vi "MC_8_27_12e_JW.vi"() -> ()   [LabVIEW 2011]
uses:
  <vilib>/Utility/file.llb/Read From Spreadsheet File (string).vi
  <vilib>/Utility/inputDevices.llb/keyboardAcquire.vi
  <vilib>/Utility/file.llb/Write To Spreadsheet File (DBL).vi
  <vilib>/Utility/file.llb/Write To Spreadsheet File (string).vi
  <vilib>/regexp/Match Regular Expression.xnode
panel:
  out "Vg Column":dbl[](array[numeric])
  out "Data Length":dbl
  in  "default (0 dbl) 6":ext format="%.2e"
  in  "default (0 dbl) 5":ext format="%.2e"
  in  "default (0 dbl) 4":ext format="%.2e"
  in  "default (0 dbl) 3":ext format="%.2e"
  in  "default (0 dbl)":ext format="%.2e"
  out "X Axis Display Type":string
  out "Opj X Axis":string
  in  "Room Temp":dbl=294.0
  out "No Image 2":path=path "\\\\acad1\\physics/Jurchescu-group/JW-PD/Image Not Found.png"
  out "Save1 Array":string[][](array[string])
  out "Lin Vd":dbl
  out "Lin-Vg Array-Used":dbl[](array[numeric])
  out "Lin Id-Used":dbl[](array[numeric])
  out "Rec: Comments":string
  out "Folder Index":dbl caption="Length"
  out "Current \nRecord":string[](array[string])
  out "Transformer \nHeaders":string[](array[string])
  out "Current Device ID":string
  out "Column":string
  out "Row":string
  out "Rec: Concentration":dbl
  out "Rec: Solvent":string
  out "Rec: Method":string
  in  "?":T1(tab)
  in  "Transport File":path
  out "Transport Folder":path
  out "Rec: Material":string
  out "Accel (RPM/s):":dbl
  in  "Transfer File":path
  out "Transfer Folder":path
  in  "Image Folder":path
  out "Image File":path=path "D:/UserData/Desktop/Jeremy/WFU/Research/Programs/VI mods/Image Not Found.png"
  in  "Manual Comments":bool
  in  "Comments:":string
  out "Calc: On/Off":dbl caption="On/Off-Sat" format="%#.2e"
  out "Calc: Off I-Sat":dbl caption="Off I-Sat" format="%#.2e"
  in  "Manuel-Dielectric":bool
  in  "Manuel-Length":bool
  out "Calc: VT-Lin":dbl
  out "New: VT-Lin":dbl
  out "Rec: VT-Lin":dbl caption="VT-Lin" format="%#_3g"
  out "Calc: Trap Density-STS":dbl format="%#.2e"
  out "New: Trap Density-STS":dbl format="%#.2e"
  out "Rec: Trap Density-STS":dbl caption="N-Sat (STS)" format="%#.2e"
  out "Calc: Trap Density-VT":dbl format="%#.2e"
  out "New: Trap Density-VT":dbl format="%#.2e"
  out "Rec: Trap Density-VT":dbl caption="N-Sat (VT)" format="%#.2e"
  out "Calc: Mobility-Lin":dbl format="%#.2e"
  out "New: Mobility-Lin":dbl format="%#_4e"
  out "Rec: Mobility-Lin":dbl caption="Mobility-Lin" format="%#_3e"
  out "Calc: Mobility-Sat":dbl format="%#.2e"
  out "Rec: Length":dbl caption="Length" format="%#_3g"
  out "Rec: Width":dbl caption="Width" format="%#_4g"
  out "Rec: Dielectric (d)":dbl caption="Dielectric (d)" format="%#_3g"
  in  "Cancel Button":bool
  in  "Up Button":bool
  in  "Down Button":bool
  out "Data Name:":string
  in  "Save Changes?":bool
  in  "New: Dielectric":dbl
  in  "New: Length":dbl
  in  "New: Width":dbl
  out "New: Mobility-Sat":dbl format="%#.2e"
  in  "Blank Button":bool
  in  "Zoom":i16(slide)=-3 scale=-5.0..5.0
  out "Image Out 2":T2(plugin-control)
  out "Image Out":T2(plugin-control)
  in  "Magnification":u16(ring) items=["5x", "10x", "20x", "50x", "80x"]
  out "Total Width":dbl
  out "Distances":dbl[](array[numeric])
  in  "Undo Button":bool
  in  "Remove Button":bool
  out "Rec: Mobility-Sat":dbl caption="Mobility-Sat" format="%#.2e"
  in  "Export":bool
  out "Calc: VT-Sat":dbl format="%#.2g"
  out "New: VT-Sat":dbl format="%#.2g"
  in  "Manual-Width":bool caption="Manual"
  out "Calc: STS":dbl format="%#.2g"
  out "New: STS":dbl format="%#.2g"
  out "Rec: VT-Sat":dbl caption="VT-Sat" format="%#.2g"
  out "Rec: STS":dbl caption="STS-Sat" format="%#.2g"
  out "Rec: On/Off":dbl caption="On/Off-Sat" format="%#.2e"
  in  "Save Changes? 2":bool
  in  "Save Changes? 3":bool
  out "Rec: Temp":dbl caption="Sample Temp" format="%.1f"
  in  "New: Temp":dbl format="%.1f"
  out "Rec: Off I-Sat":dbl caption="Off I-Sat" format="%#.2e"
  in  "Independant Variable":string(combo)="Length (um):"
  in  "Transfer Plots":T3(tab)=enum."Saturation"
  in  "Lin-Trans Slider":dbl(slide) step=1.0 scale=-22.0..89.0 scale format="%#_1p"
  out "Sqrt-Lin":cluster{dbl[], dbl[]}[](graph)
  in  "Next Sqrt Lin":bool
  in  "Previous Sqrt Lin":bool
  in  "Sat-Trans Slider":dbl(slide) step=1.0 scale=-40.0..40.0 scale format="%#_1p"
  out "Sqrt-Sat":cluster{dbl[], dbl[]}[](graph)
  in  "Previous Sqrt Sat":bool
  in  "Next Sqrt Sat":bool
  out "Raw- Lin":cluster{dbl[], dbl[]}[](graph)
  out "Raw- Sat":cluster{dbl[], dbl[]}[](graph)
  in  "Log Plots":enum32{"Linear", "Saturation", "Transport"}(tab)=enum."Saturation"
  in  "Lin-Log Slider":dbl(slide) step=1.0 scale=-1.0..82.0 scale format="%#_1p"
  in  "Previous Log Lin":bool
  in  "Next Log Lin":bool
  out "Log-Lin":cluster{dbl[], dbl[]}[](graph)
  in  "Sat-Log Slider":dbl(slide) step=1.0 scale=-1.0..82.0 scale format="%#_1p"
  in  "Previous Log Sat":bool
  in  "Next Log Sat":bool
  out "Sat-Log":cluster{dbl[], dbl[]}[](graph)
  out "Transport":cluster{dbl[], dbl[]}[](graph)
  in  "Manual-Temp":bool caption="Manual"
  out "Date Created":string caption="Fabricated"
  out "Date Recorded":string="Date Recorded" caption="Measured"
  out "Image Name":string
  out "Index":string
  in  "Num Pts":dbl=5.0
  in  "NumPoints Log":dbl=5.0 caption="Num Pts"
  in  "Ring":u16(ring) items=["Extra Small", "Small", "Medium", "Large", "Extra Large"]
  in  "Transport Line Color":u32(colorbox)
  in  "Origin Project File":path=path "\\\\acad1\\physics/Jurchescu-group/JW-PD/Group Library/Origin Project Files/DeviceData_8_10_12a_JW.opj"
  in  "No Image File":path=path "\\\\acad1\\physics/Jurchescu-group/JW-PD/Mega Awesome/Image Not Found.png"
  in  "Ramp (s):":dbl=3.0
  in  "Fabricator:":string="NaN"
  in  "Sample #:":dbl=1.0
  in  "Wait Time (s):":dbl=nan
  in  "RPM:":dbl=nan
  in  "Time (s):":dbl=nan
  in  "Room Temp (F):":dbl=nan
  in  "Relative Humidity (%):":dbl=nan
  in  "Solution Temp (C):":dbl=nan
  in  "# Drops*:":dbl=inf
  in  "Surface Treatment:":string="NaN"
  in  "Treatment Concentration (mM):":dbl=nan
  out "String":string
  out "Index 2":dbl
  out "Sat Id-Log-Used":dbl[](array[numeric])
  out "Vg Array-Log-Used":dbl[](array[numeric])
  out "ROI Descriptor out":T4 {"Contours"."Type" items=["No Selection", "Point", "Line", "Rectangle", "Oval", "Polygon", "Freehand Region", "Annulus", "Unused2", "Unused3", "Broken Line", "Freehand Line", "Rotated Rectangle"]}
  out "ROI Descriptor":T4 {"Contours"."Type" items=["No Selection", "Point", "Line", "Rectangle", "Oval", "Polygon", "Freehand Region", "Annulus", "Unused2", "Unused3", "Broken Line", "Freehand Line", "Rotated Rectangle"]}
  out "Numeric 3":dbl
  out "Array 6":dbl[][](array[numeric])
  out "Cluster":T5
  out "Array 5":dbl[](array[numeric])
  out "Array 4":dbl[](array[numeric])
  out "Array 3":dbl[](array[numeric])
  out "Numeric 2":dbl
  out "Numeric":dbl
  out "Sat Id-Used":dbl[](array[numeric])
  out "Sat Vg Array-Used":dbl[](array[numeric])
  out "MobVi Index":dbl
  in  "Row Start":dbl=20.0
  # "Data Locations"
  # "Transfer Location"
  # "Image Location"
  # "Recorded"
  # "Calculated"
  # "Re-Calculated"
  # "Manual"
  # "Used points display at y=0"
  # "Slider\nDoesn't\nWork"
  # "Slider\nDoesn't\nWork"
  # "No new points displayed"
  # "Sample Properties"
  # "*     Inf = Full coverage\n   NaN = Unknown or Not Applicable"
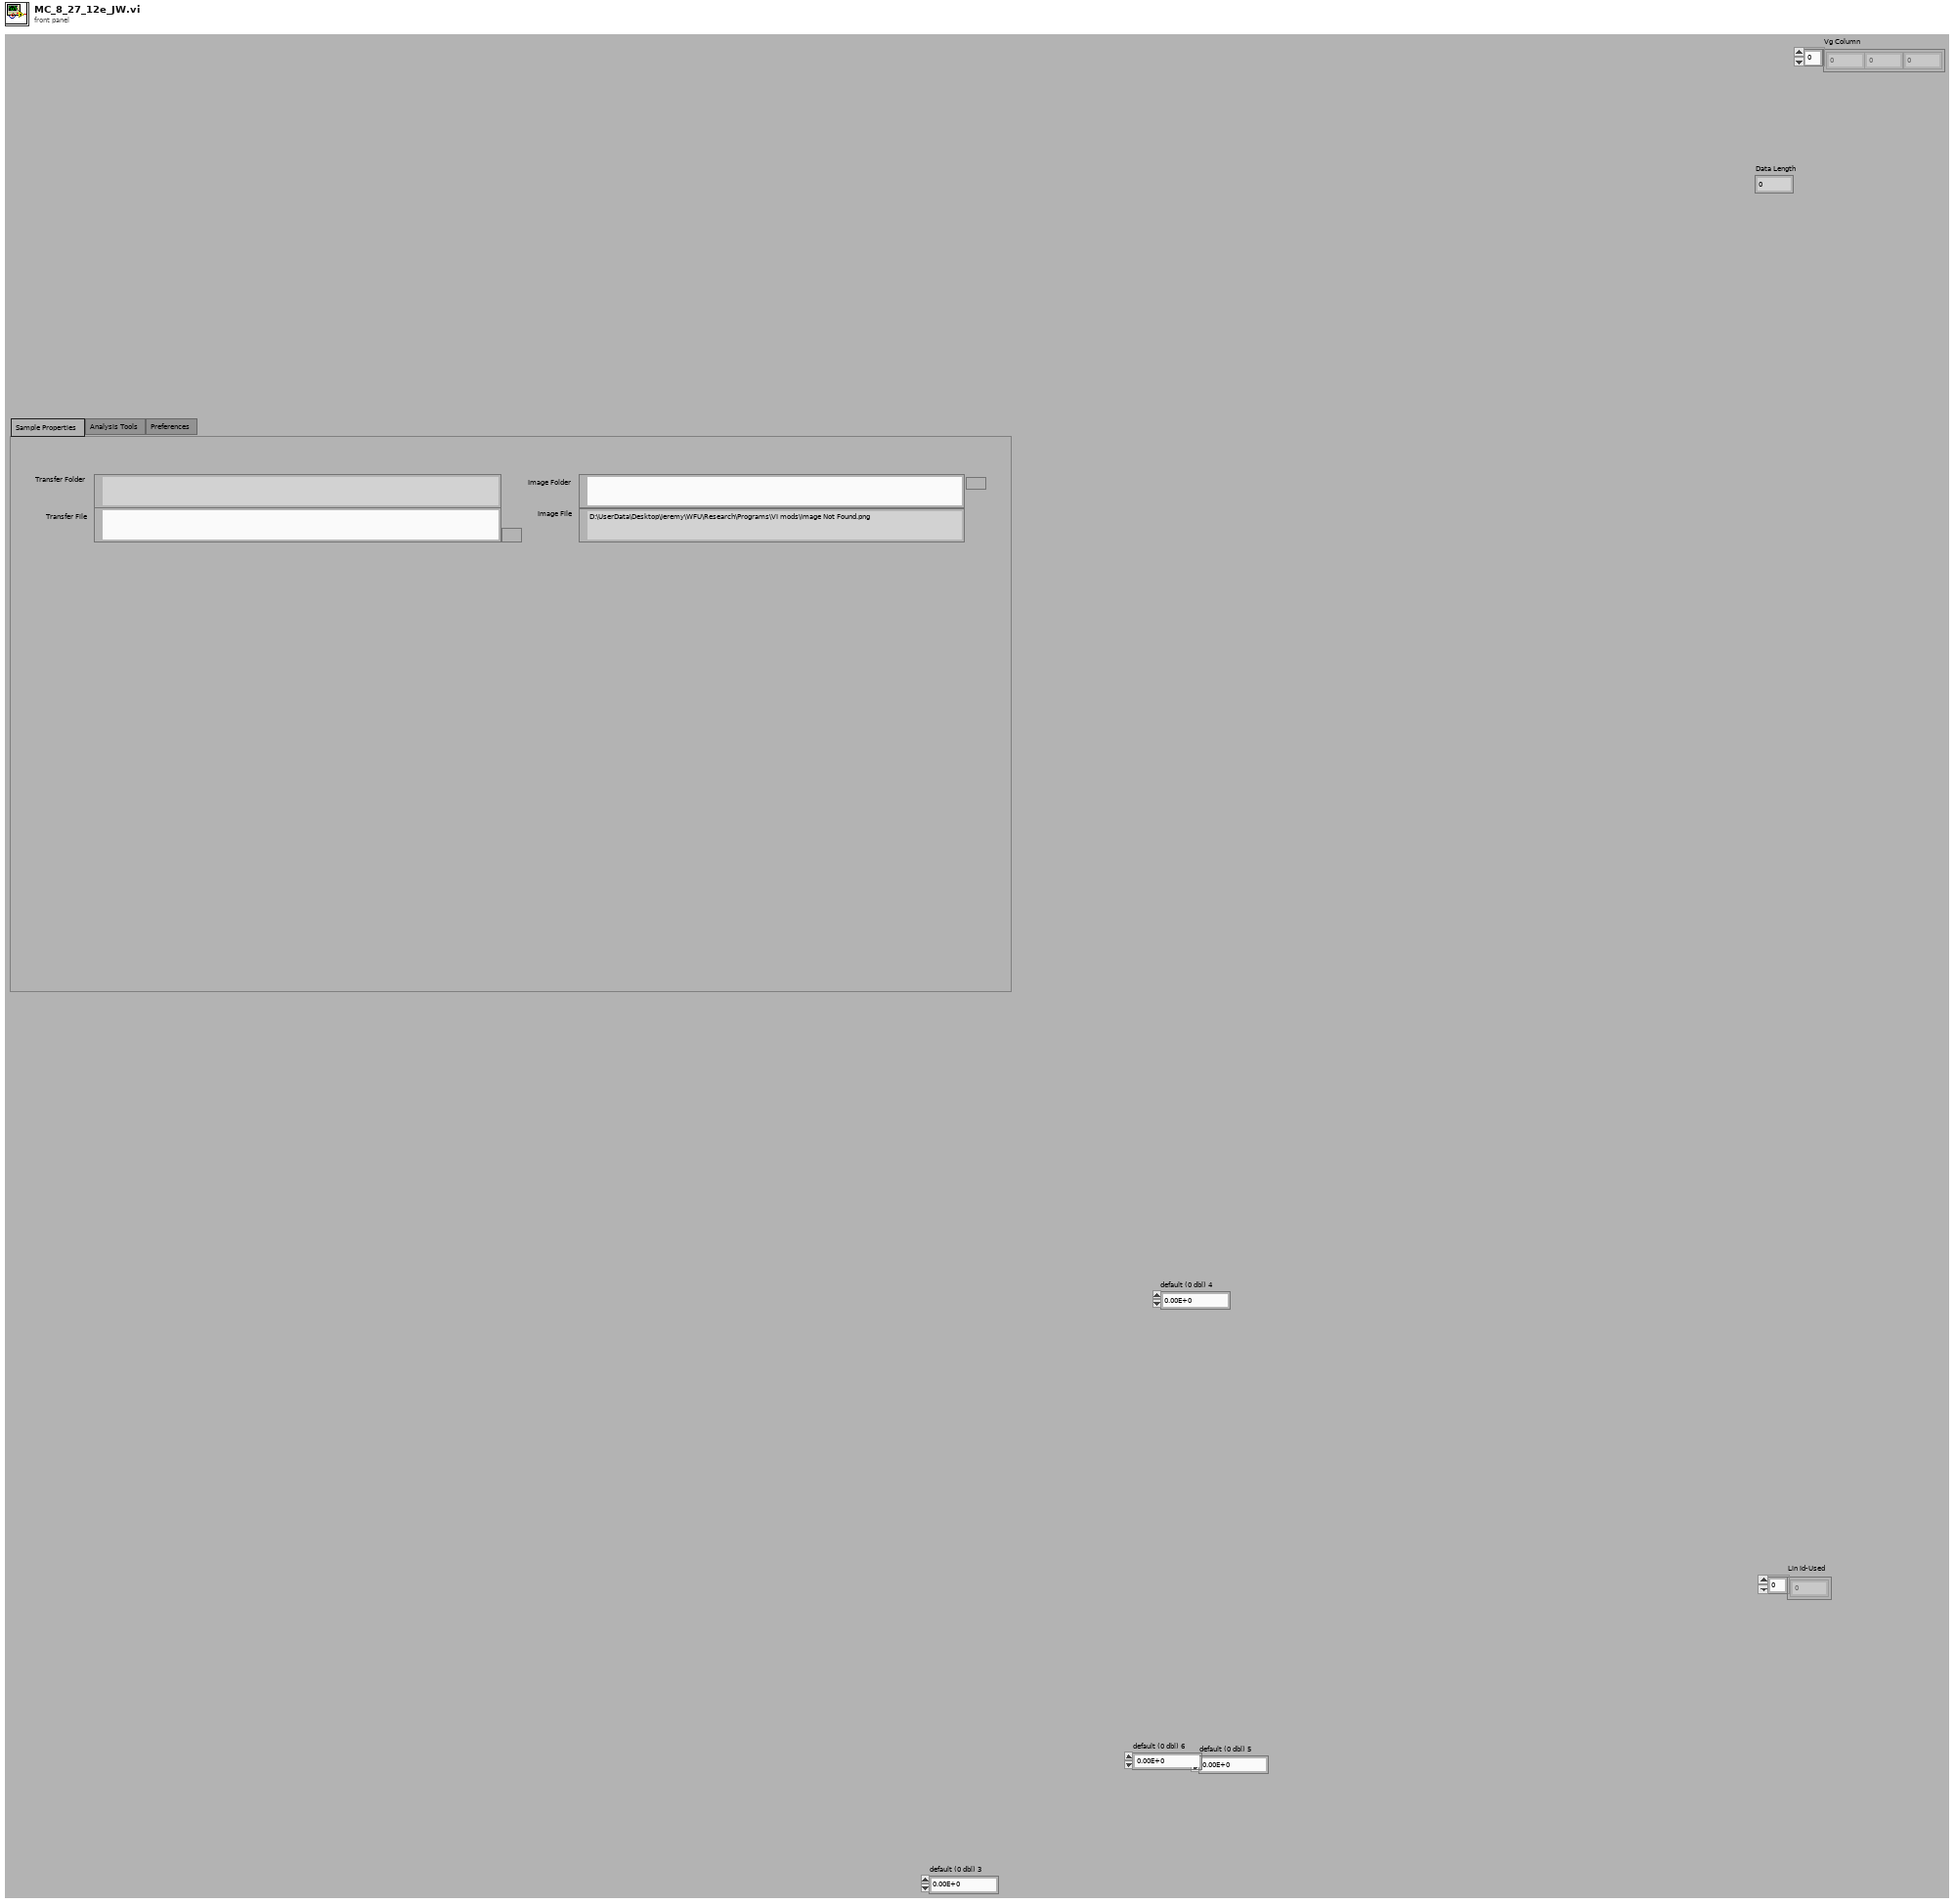
[diagram p1: front panel]
types:
  T1 = enum32{"Sample Properties", "Analysis Tools", "Preferences", "Current Database"}
  T2 = typedef "IMAQ Image.ctl" = refnum<image>
  T3 = enum32{"Linear", "Saturation", "Raw-Linear", "Raw-Saturation"}
  T4 = typedef "ROI Descriptor" = cluster{"Global Rectangle":i32[], "Contours":cluster{"ID":enum32{"External", "Internal"}, "Type":u32, "Coordinates":i32[]}[]}
  T5 = cluster{"Numeric":dbl, "Numeric 2":dbl, "Numeric 3":dbl, "Numeric 4":dbl}
  T6 = cluster{"Mobility-Sat":dbl, "Moblitity-Lin":dbl, "On/Off":dbl, "Off Current":dbl, "Vt-Sat":dbl, "STS":dbl, "Trap Density-VT":dbl, "Trap Density-STS":dbl}
  T7 = cluster{"Date Recorded":string, "Index":string, "Length":dbl, "Width":dbl, "Sample Temp":dbl}
  T8 = cluster{"Date Created":string, "Material":string, "Solvent":string, "Concentration":dbl, "Method":string, "Dielectric (nm)":dbl, "Treatment":string, "Comments":string}
  T9 = cluster{"Raw Sat":cluster{dbl[], dbl[]}[], "Sqrt Sat":cluster{dbl[], dbl[]}[], "Log Sat":cluster{dbl[], dbl[]}[], "Raw Lin":cluster{dbl[], dbl[]}[], "Sqrt Lin":cluster{dbl[], dbl[]}[], "Log Lin":cluster{dbl[], dbl[]}[]}
  T10 = cluster{"Mobility-Sat":dbl, "Vt-Sat":dbl, "Mobility-Lin":dbl, "Vt-Lin":dbl, "Off I-Sat":dbl, "On/Off I-Sat":dbl}
  T11 = cluster{"[0]":cluster{dbl[], dbl[]}, "[1]":cluster{dbl[], dbl[]}, "[2]":cluster{dbl[], dbl[]}, "[3]":cluster{dbl[], dbl[]}, "[4]":cluster{dbl[], dbl[]}, "[5]":cluster{dbl[], dbl[]}, "[6]":cluster{dbl[], dbl[]}, "[7]":cluster{dbl[], dbl[]}, "[8]":cluster{dbl[], dbl[]}}
  T12 = cluster{"Global Rectangle":i32[], "Contours":cluster{"Contour Type":u32, "ROI Type":u32, "Points":i32[]}[]}
  T13 = typedef "LVBoundsTypeDef.ctl" = cluster{"Width":u32, "Height":u32}
  T14 = enum16{"0", "1", "2", "3", "4", "5", "6", "7", "8", "9", "A", "B", "C", "D", "E", "F", "G", "H", "I", "J", "K", "L", "M", "N", "O", "P", "Q", "R", "S", "T", "U", "V", "W", "X", "Y", "Z", "F1", "F2", "F3", "F4", "F5", "F6", "F7", "F8", "F9", "F10", "F11", "F12", "F13", "F14", "F15", "ADD", "BACK", "BACKSLASH", "CAPITAL", "COMMA", "DECIMAL", "DELETE", "DIVIDE", "DOWN", "END", "EQUALS", "ESCAPE", "GRAVE (`)", "HOME", "INSERT", "LBRACKET", "LCONTROL", "LEFT", "L ALT", "LSHIFT", "LWIN", "MINUS", "MULTIPLY", "NEXT", "NUMLOCK", "NUMPAD_0", "NUMPAD_1", "NUMPAD_2", "NUMPAD_3", "NUMPAD_4", "NUMPAD_5", "NUMPAD_6", "NUMPAD_7", "NUMPAD_8", "NUMPAD_9", "PAUSE", "PERIOD", "PRIOR (PG UP)", "RBRACKET", "RCONTROL", "RETURN", "RIGHT", "R ALT", "RSHIFT", "RWIN", "SCROLL", "SEMICOLON", "SLASH", "SPACE", "SUBTRACT", "TAB", "UP", "ENTER (num pad)", "' (quote)"}[]
  T15 = enum16{"0", "1", "2", "3", "4", "5", "6", "7", "8", "9", "A", "B", "C", "D", "E", "F", "G", "H", "I", "J", "K", "L", "M", "N", "O", "P", "Q", "R", "S", "T", "U", "V", "W", "X", "Y", "Z", "F1", "F2", "F3", "F4", "F5", "F6", "F7", "F8", "F9", "F10", "F11", "F12", "F13", "F14", "F15", "ADD", "BACK", "BACKSLASH", "CAPITAL", "COMMA", "DECIMAL", "DELETE", "DIVIDE", "DOWN", "END", "EQUALS", "ESCAPE", "GRAVE (`)", "HOME", "INSERT", "LBRACKET", "LCONTROL", "LEFT", "L ALT", "LSHIFT", "LWIN", "MINUS", "MULTIPLY", "NEXT", "NUMLOCK", "NUMPAD_0", "NUMPAD_1", "NUMPAD_2", "NUMPAD_3", "NUMPAD_4", "NUMPAD_5", "NUMPAD_6", "NUMPAD_7", "NUMPAD_8", "NUMPAD_9", "PAUSE", "PERIOD", "PRIOR (PG UP)", "RBRACKET", "RCONTROL", "RETURN", "RIGHT", "R ALT", "RSHIFT", "RWIN", "SCROLL", "SEMICOLON", "SLASH", "SPACE", "SUBTRACT", "TAB", "UP", "ENTER (num pad)", "' (quote)"}
  T16 = cluster{"Contour Type":u32, "ROI Type":u32, "Points":i32[]}[]
  T17 = cluster{i32[], cluster{"Contour Type":u32, "ROI Type":u32, "Points":i32[]}[]}
  T18 = cluster{"Independant  Variable Indicator":string, "Parameter String Indicator":string}
  T19 = cluster{string, sgl, bool, bool, bool, bool, bool, bool, i32}
  T20 = cluster{i32, cluster{string, sgl, bool, bool, bool, bool, bool, bool, i32}, i32, i32}
  T21 = cluster{"Contour Type":u32, "ROI Type":u32, "Points":i32[]}
  T22 = cluster{"Points[0]":i32, "Points[1]":i32, "Points[2]":i32, "Points[3]":i32, "Points[4]":i32, "Points[5]":i32, "Points[6]":i32, "Points[7]":i32, "Points[8]":i32}
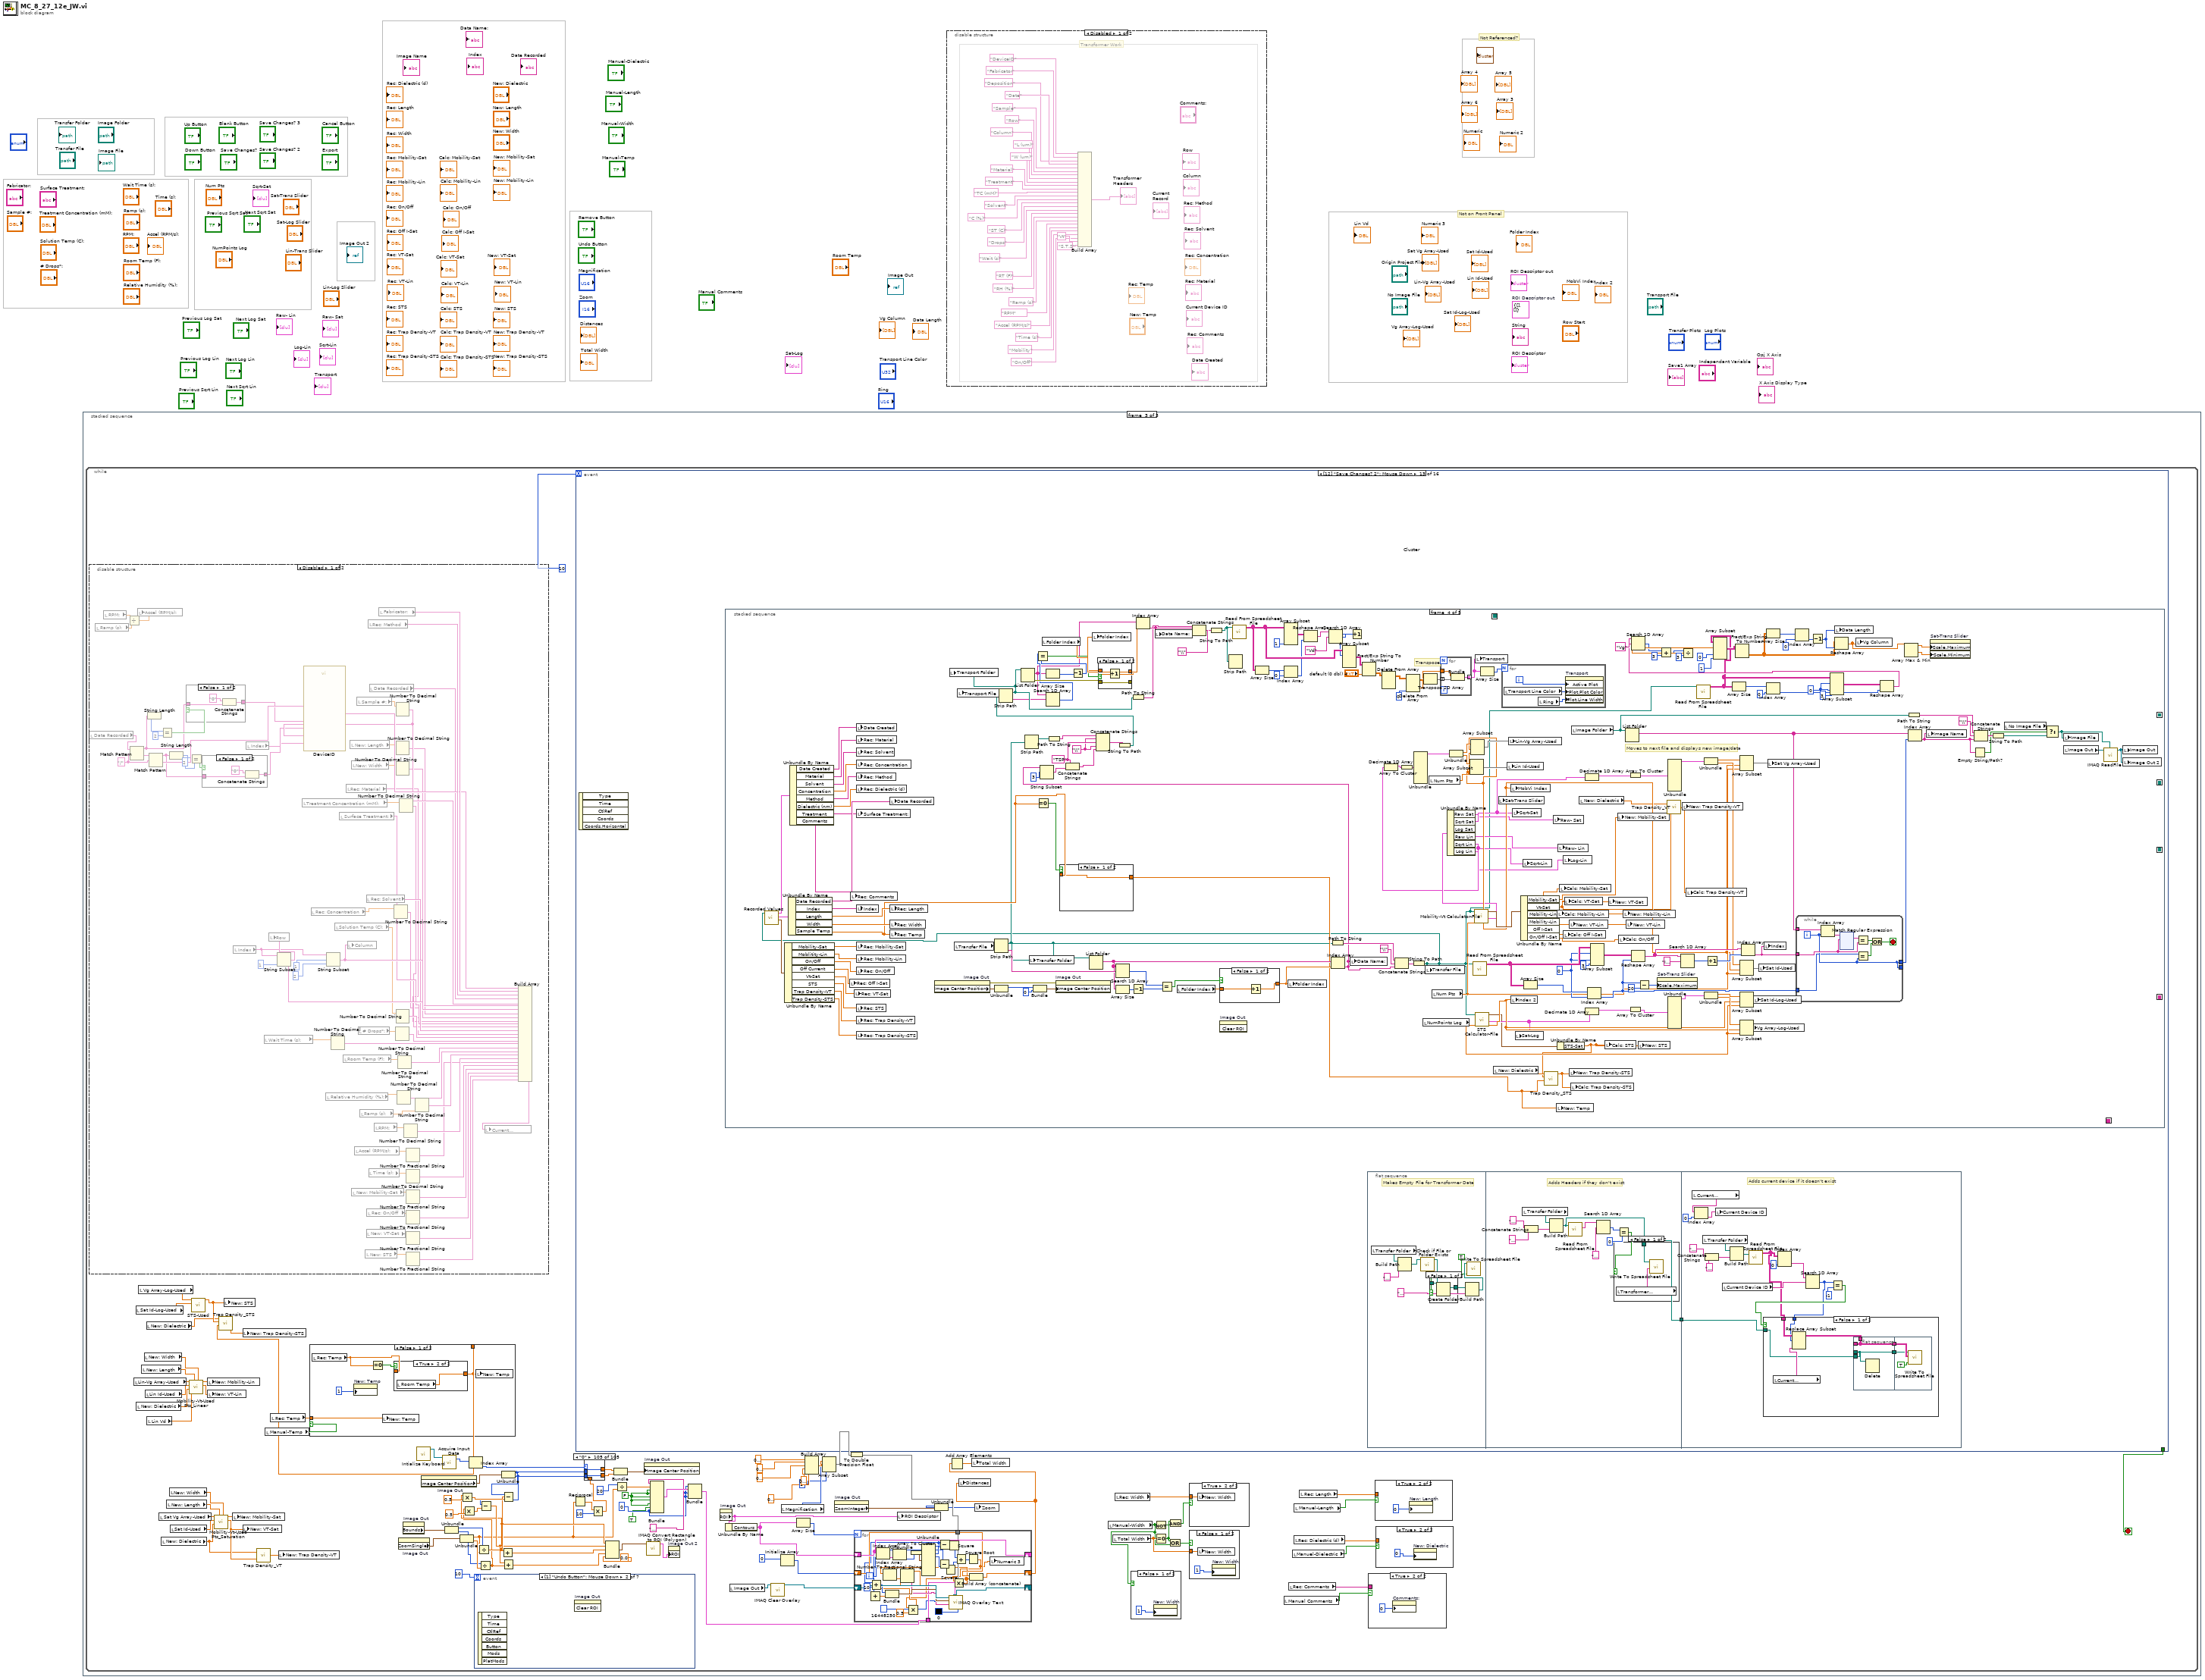
[diagram p0: block diagram]
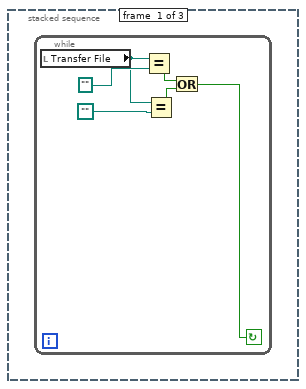
[diagram p3: hidden frame]
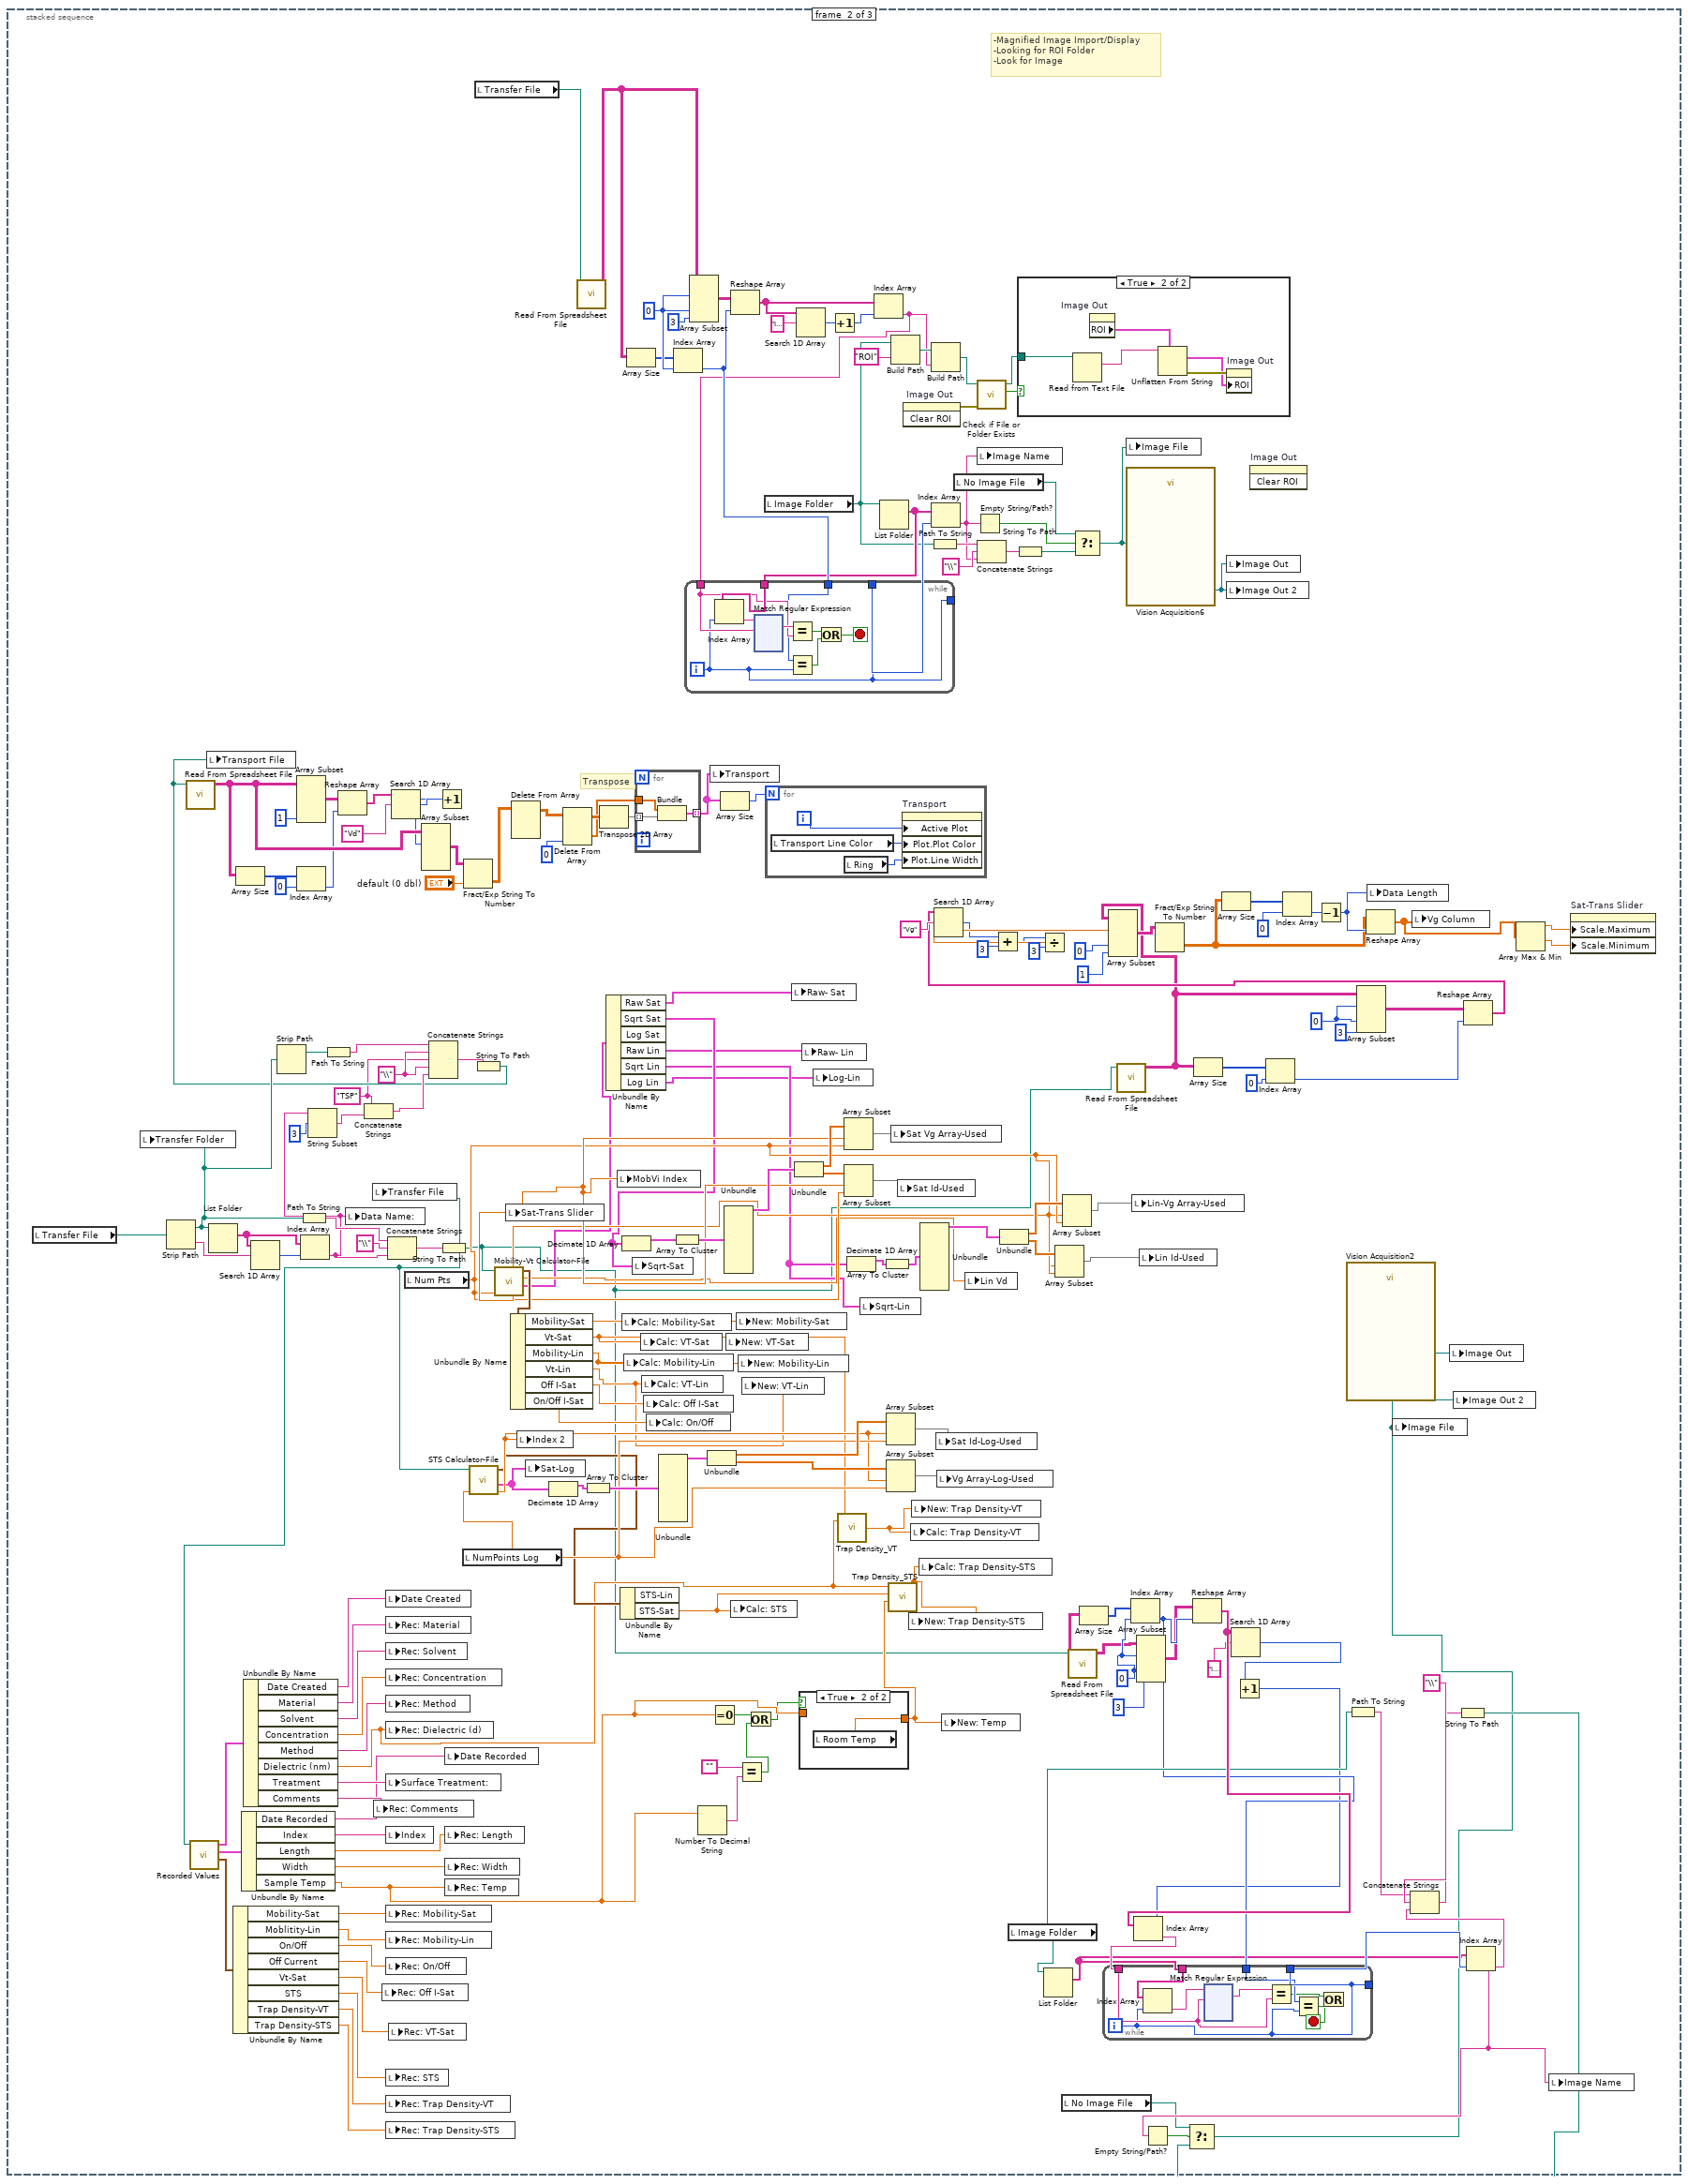
[diagram p4: hidden frame]
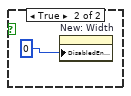
[diagram p10: hidden frame]
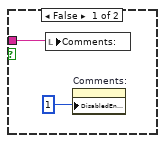
[diagram p11: hidden frame]
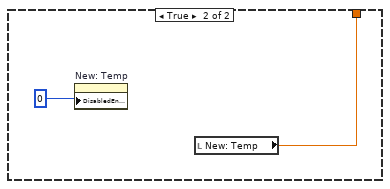
[diagram p13: hidden frame]
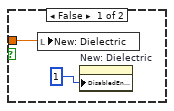
[diagram p14: hidden frame]
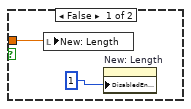
[diagram p15: hidden frame]
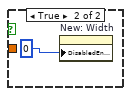
[diagram p17: hidden frame]
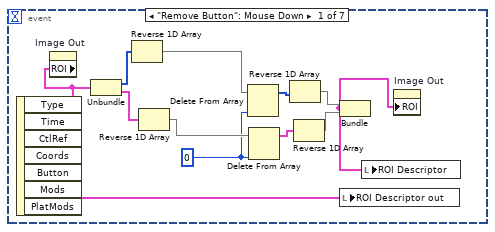
[diagram p18: hidden frame]
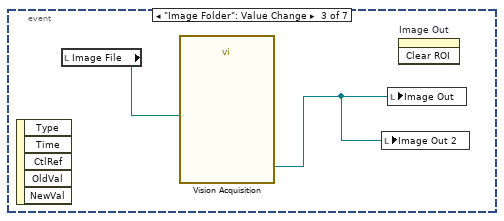
[diagram p19: hidden frame]
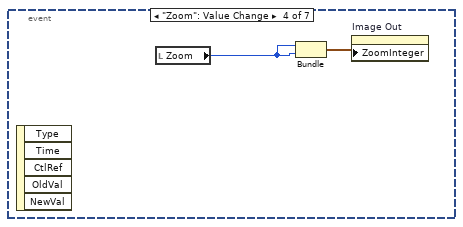
[diagram p20: hidden frame]
diagram:
  (unwired) T4 {"Global Rectangle"=[], "Contours"=[]}  # ROI Descriptor out
  # "Not Referenced?"
  # "Not on Front Panel"
  n1 = stacked-sequence {
    frame #0 {
      n2 = while {
        stop <- w1 continue-if-true
        n3 = local read "Transfer File"() -> (w3:path)
        n4 = Equal?(x=w3, y=path "") -> (x = y?=w5:bool)
        n5 = Equal?(x=w3, y=path "") -> (x = y?=w4:bool)
        n6 = Or(x=w5, y=w4) -> (x .or. y?=w1:bool)
      }
    }
    frame #1 {
      w29 = 0
      w35 = "\\"
      w34 = "TSP"
      w164 = 0
      w187 = 0
      # "Transpose"
      # "-Magnified Image Import/Display\n-Looking for ROI Folder\n-Look for Image"
      n7 = local read "Transfer File"() -> (w168:path)
      n8 = Strip Path(path=w168) -> (stripped path=w44:path, name=w155:string)
      n9 = local write "Transfer Folder"(w44) -> ()
      n10 = List Folder(path=w44) -> (filenames=w159:string[])  [unwired: 3 in, 3 out]
      n11 = Search 1D Array(1D array=w159, element=w155) -> (index of element=w158:i32)  [unwired: 1 in]
      n12 = Strip Path(path=w44) -> (stripped path=w40:path)  [unwired: 1 out]
      n13 = Path To String(path=w44) -> (string=w154:string)
      n14 = Index Array(array=w159, index=w158) -> (element=w43:string)
      n15 = String Subset(string=w43, offset (0)=3) -> (substring=w41:string)  [unwired: 1 in]
      n16 = Path To String(path=w40) -> (string=w36:string)
      n17 = local write "Data Name:"(w43) -> ()
      n18 = Concatenate Strings(w34, w41) -> (w39:string)
      n19 = Concatenate Strings(w154, "\\", w43) -> (w156:string)
      n20 = local read "Num Pts"() -> (w93:dbl)
      n21 = Concatenate Strings(w36, w35, w34, w35, w39) -> (w38:string)
      n22 = String To Path(string=w156) -> (path=w7:path)
      n23 = call "Recorded Values.vi"("Path"=w7) -> ("Recorded Char"=w123:T6, "Recorded Prop"=w122:T7, "Fabrication Prop"=w124:T8)  [unwired: 8 in]
      n24 = Unbundle By Name(w123) -> ("Mobility-Sat"=w111:dbl, "Moblitity-Lin"=w110:dbl, "On/Off"=w109:dbl, "Off Current"=w108:dbl, "Vt-Sat"=w74:dbl, "STS"=w107:dbl, "Trap Density-VT"=w106:dbl, "Trap Density-STS"=w105:dbl)
      n25 = Unbundle By Name(w122) -> ("Date Recorded"=w115:string, "Index"=w114:string, "Length"=w113:dbl, "Width"=w112:dbl, "Sample Temp"=w80:dbl)
      n26 = Unbundle By Name(w124) -> ("Date Created"=w104:string, "Material"=w121:string, "Solvent"=w120:string, "Concentration"=w119:dbl, "Method"=w118:string, "Dielectric (nm)"=w84:dbl, "Treatment"=w117:string, "Comments"=w116:string)
      n27 = local write "Transfer File"(w7) -> ()
      n28 = local write "Rec: Comments"(w116) -> ()
      n29 = local write "Rec: Off I-Sat"(w108) -> ()
      n30 = local write "Date Created"(w104) -> ()
      n31 = local write "Rec: Material"(w121) -> ()
      n32 = local write "Rec: Solvent"(w120) -> ()
      n33 = local write "Rec: Concentration"(w119) -> ()
      n34 = local write "Rec: Method"(w118) -> ()
      n35 = local write "Rec: Dielectric (d)"(w84) -> ()
      n36 = local write "Surface Treatment:"(w117) -> ()
      n37 = local write "Index"(w114) -> ()
      n38 = local write "Rec: Mobility-Sat"(w111) -> ()
      n39 = local write "Rec: Mobility-Lin"(w110) -> ()
      n40 = local write "Rec: On/Off"(w109) -> ()
      n41 = local write "Rec: STS"(w107) -> ()
      n42 = local write "Rec: Trap Density-VT"(w106) -> ()
      n43 = local write "Rec: Trap Density-STS"(w105) -> ()
      n44 = local write "Rec: VT-Sat"(w74) -> ()
      n45 = local write "Date Recorded"(w115) -> ()
      n46 = local write "Rec: Length"(w113) -> ()
      n47 = local write "Rec: Width"(w112) -> ()
      n48 = local write "Rec: Temp"(w80) -> ()
      n49 = local read "NumPoints Log"() -> (w101:dbl)
      n50 = call "STS Calculator-File.vi"("NumPts"=w101, "Path"=w7) -> ("STS Index-Sat"=w100:dbl, "XY Graph-Sat"=w33:cluster{dbl[], dbl[]}[], "Ouput"=w99:cluster{"STS-Sat":dbl, "STS-Lin":dbl})  [unwired: 5 in, 2 out]
      n51 = String To Path(string=w38) -> (path=w37:path)
      n52 = call-poly <vilib>:"Read From Spreadsheet File.vi"("file path (dialog if empty)"=w37) -> ("all rows"=w58:string[][])  [unwired: 6 in, 4 out]
      n53 = local write "Transport File"(w37) -> ()
      n54 = Array Size(array=w58) -> (size(s)=w64:i32[])
      n55 = Array Subset(array=w58, length (col)=1) -> (w60:string[][])  [unwired: 3 in]
      n56 = Index Array(array=w64, index=0) -> (element=w53:i32)
      n57 = Reshape Array(w60, w53) -> (w59:string[])
      n58 = Search 1D Array(1D array=w59, element="Vd") -> (index of element=w57:i32)  [unwired: 1 in]
      n59 = Increment(x=w57) -> (x+1=w56:i32)
      n60 = Array Subset(array=w58, index (row)=w56) -> (w54:string[][])  [unwired: 3 in]
      n61 = Fract/Exp String To Number(string=w54, default (0 dbl)="default (0 dbl)") -> (number=w46:ext[][])  [unwired: 2 in, 1 out]
      n62 = local read "Transfer File"() -> (w182:path)
      n63 = call "Mobility-Vt Calculator-File.vi"("NumPts"=w93, "Path"=w7) -> ("Graph Cluster"=w65:T9, "Lin Vd"=w89:dbl, "Output"=w103:T10, "Index-Sat"=w102:dbl, "Index-Lin"=w92:dbl)  [unwired: 5 in]
      n64 = local write "Sat-Trans Slider"(w102) -> ()
      n65 = Unbundle By Name(w103) -> ("Mobility-Sat"=w83:dbl, "Vt-Sat"=w82:dbl, "Mobility-Lin"=w73:dbl, "Vt-Lin"=w71:dbl, "Off I-Sat"=w88:dbl, "On/Off I-Sat"=w72:dbl)
      n66 = Delete From Array(array=w46) -> (array with subset deleted=w45:ext[][])  [unwired: 3 in, 1 out]
      n67 = local write "Index 2"(w100) -> ()
      n68 = local write "Sat-Log"(w33) -> ()
      n69 = Decimate 1D Array(w33) -> (w146:cluster{dbl[], dbl[]}[])  [unwired: 1 out]
      n70 = Delete From Array(array=w45, index (col)=0 ("Deaktivierter Index (Spalte)")) -> (deleted portion=w50:ext[], array with subset deleted=w51:ext[][])  [unwired: 2 in]
      n71 = call-poly <vilib>:"Read From Spreadsheet File.vi"("file path (dialog if empty)"=w182) -> ("all rows"=w185:string[][])  [unwired: 6 in, 4 out]
      n72 = Array To Cluster(array=w146) -> (cluster=w148:T11)
      n73 = Transpose 2D Array(2D array=w51) -> (transposed array=w52:ext[][])
      n74 = Unbundle By Name(w65) -> ("Raw Sat"=w68:cluster{dbl[], dbl[]}[], "Sqrt Sat"=w70:cluster{dbl[], dbl[]}[], "Raw Lin"=w67:cluster{dbl[], dbl[]}[], "Sqrt Lin"=w69:cluster{dbl[], dbl[]}[], "Log Lin"=w66:cluster{dbl[], dbl[]}[])  [unwired: 1 out]
      n75 = local write "MobVi Index"(w102) -> ()
      n76 = Unbundle By Name(w99) -> ("STS-Sat"=w87:dbl)  [unwired: 1 out]
      n77 = Decimate 1D Array(w70) -> (w181:cluster{dbl[], dbl[]}[])  [unwired: 1 out]
      n78 = local write "Calc: Mobility-Sat"(w83) -> ()
      n79 = local write "Calc: Mobility-Lin"(w73) -> ()
      n80 = Array Size(array=w185) -> (size(s)=w186:i32[])
      n81 = local write "Sqrt-Sat"(w70) -> ()
      n82 = for {
        tunnel: w50 -> [w203]
        tunnel: w52 -> [w204] mode=indexing
        tunnel: [w202] -> w48 mode=indexing
        n83 = Bundle(w203, w204) -> (w202:cluster{ext[], ext[]})  [unwired: 1 in]
      }
      n84 = local write "Calc: VT-Sat"(w82) -> ()
      n85 = local write "Calc: VT-Lin"(w71) -> ()
      n86 = local write "Calc: Off I-Sat"(w88) -> ()
      n87 = local write "Calc: On/Off"(w72) -> ()
      n88 = Unbundle(w148) -> ("[0]"=w147:cluster{dbl[], dbl[]})  [unwired: 8 out]
      n89 = Array To Cluster(array=w181) -> (cluster=w179:T11)
      n90 = Index Array(array=w186, index=w187) -> (element=w193:i32)
      n91 = Array Subset(array=w185, index (row)=w187, index (col)=w187, length (col)=3) -> (w184:string[][])  [unwired: 1 in]
      n92 = Number To Decimal String(number=w80) -> (decimal integer string=w78:string)  [unwired: 1 in]
      n93 = Unbundle(w147) -> (w144:dbl[], w143:dbl[])
      n94 = local write "Transport"(w48) -> ()
      n95 = Equal To 0?(x=w80) -> (x = 0?=w79:bool)
      n96 = Array Size(array=w48) -> (size(s)=w47:i32)
      n97 = Unbundle(w179) -> ("[0]"=w180:cluster{dbl[], dbl[]})  [unwired: 8 out]
      n98 = local write "New: VT-Sat"(w82) -> ()
      n99 = Reshape Array(w184, w193) -> (w198:string[])
      n100 = local write "Calc: STS"(w87) -> ()
      n101 = local write "New: Mobility-Sat"(w83) -> ()
      n102 = Equal?(x="", y=w78) -> (x = y?=w76:bool)
      n103 = local write "New: Mobility-Lin"(w73) -> ()
      n104 = local write "New: VT-Lin"(w71) -> ()
      n105 = Or(x=w79, y=w76) -> (x .or. y?=w75:bool)
      n106 = local read "Image Folder"() -> (w125:path)
      n107 = for {
        N: w47 -> [_]
        i -> [w201]
        n108 = local read "Transport Line Color"() -> (w200:u32)
        n109 = local read "Ring"() -> (w199:u16)
        n110 = property on="Transport" class="XYGraph (strict)"("Active Plot"=w201, "Plot.Plot Color"=w200, "Plot.Line Width"=w199) -> ()  [unwired: 2 in, 2 out]
      }
      n111 = local write "Raw- Sat"(w68) -> ()
      n112 = Unbundle(w180) -> (w145:dbl[], w149:dbl[])
      n113 = Search 1D Array(1D array=w198, element="Index:") -> (index of element=w190:i32)  [unwired: 1 in]
      n114 = case shown="True" w75 {
        tunnel: [w205 w206] -> w86
        tunnel: w80 -> [w205 _]
        frame False {
        }
        frame True {
          n115 = local read "Room Temp"() -> (w206:dbl)
        }
      }
      n116 = local write "Raw- Lin"(w67) -> ()
      n117 = local write "Log-Lin"(w66) -> ()
      n118 = Increment(x=w190) -> (x+1=w189:i32)
      n119 = call "Trap Density_VT.vi"("VT"=w82, "Dielectric"=w84) -> ("Trap Density-VT"=w81:dbl)
      n120 = Array Subset(array=w145, index=w102, length=w93) -> (w152:dbl[])
      n121 = Array Subset(array=w149, index=w102, length=w93) -> (w153:dbl[])
      n122 = Decimate 1D Array(w69) -> (w98:cluster{dbl[], dbl[]}[])  [unwired: 1 out]
      n123 = local write "Sqrt-Lin"(w69) -> ()
      n124 = Index Array(array=w198, index=w189) -> (element=w126:string)
      n125 = List Folder(path=w125) -> (filenames=w191:string[])  [unwired: 3 in, 3 out]
      n126 = while {
        tunnel: w191 -> [w339]
        tunnel: w126 -> [w337]
        tunnel: [w336] -> _
        tunnel: [w336] -> w192
        tunnel: w193 -> [w335]
        i -> [w336]
        stop <- w332 stop-if-true
        n127 = Index Array(array=w339, index=w336) -> (element=w340:string)
        n128 = xnode "Match Regular Expression"("input string"=w340, "regular expression"=w337) -> ("whole match"=w338:string)  [unwired: 4 in, 4 out]
        n129 = Equal?(x=w338, y=w337) -> (x = y?=w334:bool)
        n130 = Equal?(x=w335, y=w336) -> (x = y?=w333:bool)
        n131 = Or(x=w334, y=w333) -> (x .or. y?=w332:bool)
      }
      n132 = Array To Cluster(array=w98) -> (cluster=w97:T11)
      n133 = Array Subset(array=w144, index=w100, length=w101) -> (w151:dbl[])
      n134 = Array Subset(array=w143, index=w100, length=w101) -> (w150:dbl[])
      n135 = call "Trap Density_STS.vi"("Temp (T) [K]"=w86, "S.T.S. (S)"=w87, "Dielectric"=w84) -> ("Trap Density (N)"=w85:dbl)  [unwired: 8 in]
      n136 = Build Path(base path=w125, name or relative path="ROI") -> (appended path=w128:path)
      n137 = local write "Sat Vg Array-Used"(w152) -> ()
      n138 = local write "Sat Id-Used"(w153) -> ()
      n139 = invoke on="Image Out" class="ImageControl" method="Clear ROI"() -> (error out=w132:errorcluster)  [unwired: 3 in, 2 out]
      n140 = local write "New: Trap Density-STS"(w85) -> ()
      n141 = local write "Calc: Trap Density-VT"(w81) -> ()
      n142 = local write "New: Trap Density-VT"(w81) -> ()
      n143 = local write "Calc: Trap Density-STS"(w85) -> ()
      n144 = Unbundle(w97) -> ("[0]"=w96:cluster{dbl[], dbl[]})  [unwired: 8 out]
      n145 = Path To String(path=w125) -> (string=w195:string)
      n146 = Build Path(base path=w128, name or relative path=w126) -> (appended path=w127:path)
      n147 = Index Array(array=w191, index=w192) -> (element=w142:string)
      n148 = local write "Sat Id-Log-Used"(w151) -> ()
      n149 = local write "Vg Array-Log-Used"(w150) -> ()
      n150 = local write "New: Temp"(w86) -> ()
      n151 = local read "No Image File"() -> (w133:path)
      n152 = local write "Lin Vd"(w89) -> ()
      n153 = Empty String/Path?(string/path=w142) -> (empty?=w141:bool)
      n154 = call <vilib>:"Check if File or Folder Exists.vi"("error in (no error)"=w132, "path"=w127) -> ("file or folder exists?"=w130:bool, "dup path"=w131:path)  [unwired: 7 in, 1 out]
      n155 = local write "Image Name"(w142) -> ()
      n156 = Concatenate Strings(w195, "\\", w142) -> (w196:string)
      n157 = Unbundle(w96) -> (w95:dbl[], w94:dbl[])
      n158 = local read "Image Folder"() -> (w174:path)
      n159 = String To Path(string=w196) -> (path=w140:path)
      n160 = case shown="True" w130 {
        tunnel: w131 -> [_ w207]
        frame False {
        }
        frame True {
          n161 = Read from Text File(file (use dialog)=w207) -> (text=w211:string)  [unwired: 3 in, 3 out]
          n162 = property on="Image Out" class="ImageControl"() -> ("ROI"=w208:T12)  [unwired: 2 in, 2 out]
          n163 = Unflatten From String(type=w208, binary string=w211) -> (value=w209:T12, error out=w210:errorcluster)  [unwired: 3 in, 1 out]
          n164 = property on="Image Out" class="ImageControl"(error in=w210, "ROI"=w209) -> ()  [unwired: 1 in, 2 out]
        }
      }
      n165 = List Folder(path=w174) -> (filenames=w170:string[])  [unwired: 3 in, 3 out]
      n166 = Array Subset(array=w94, index=w92, length=w93) -> (w90:dbl[])
      n167 = local read "No Image File"() -> (w134:path)
      n168 = Array Subset(array=w95, index=w92, length=w93) -> (w91:dbl[])
      n169 = call-poly <vilib>:"Read From Spreadsheet File.vi"("file path (dialog if empty)"=w7) -> ("all rows"=w162:string[][])  [unwired: 6 in, 4 out]
      n170 = Select(t=w133, s=w141, f=w140) -> (s? t:f=w139:path)
      n171 = Array Size(array=w162) -> (size(s)=w163:i32[])
      n172 = call-poly <vilib>:"Read From Spreadsheet File.vi"("file path (dialog if empty)"=w7) -> ("all rows"=w11:string[][])  [unwired: 6 in, 4 out]
      n173 = local write "Image File"(w139) -> ()
      n174 = call "Vision Acquisition6"("Image Path"=w139) -> ("Image Out"=w194:T2)  [unwired: 25 in, 1 out]
      n175 = Index Array(array=w163, index=w164) -> (element=w173:i32)
      n176 = local write "Lin-Vg Array-Used"(w91) -> ()
      n177 = Array Subset(array=w162, index (row)=w164, index (col)=w164, length (col)=3) -> (w161:string[][])  [unwired: 1 in]
      n178 = local write "Lin Id-Used"(w90) -> ()
      n179 = Reshape Array(w161, w173) -> (w178:string[])
      n180 = Array Size(array=w11) -> (size(s)=w30:i32[])
      n181 = local write "Image Out"(w194) -> ()
      n182 = local write "Image Out 2"(w194) -> ()
      n183 = Search 1D Array(1D array=w178, element="Index:") -> (index of element=w167:i32)  [unwired: 1 in]
      n184 = Increment(x=w167) -> (x+1=w166:i32)
      n185 = Index Array(array=w178, index=w166) -> (element=w171:string)
      n186 = while {
        tunnel: w170 -> [w219]
        tunnel: w171 -> [w217]
        tunnel: [w216] -> _
        tunnel: [w216] -> w172
        tunnel: w173 -> [w215]
        i -> [w216]
        stop <- w212 stop-if-true
        n187 = Index Array(array=w219, index=w216) -> (element=w220:string)
        n188 = xnode "Match Regular Expression"("input string"=w220, "regular expression"=w217) -> ("whole match"=w218:string)  [unwired: 4 in, 4 out]
        n189 = Equal?(x=w218, y=w217) -> (x = y?=w214:bool)
        n190 = Equal?(x=w215, y=w216) -> (x = y?=w213:bool)
        n191 = Or(x=w214, y=w213) -> (x .or. y?=w212:bool)
      }
      n192 = invoke on="Image Out" class="ImageControl" method="Clear ROI"() -> ()  [unwired: 3 in, 3 out]
      n193 = Index Array(array=w30, index=0) -> (element=w28:i32)
      n194 = Path To String(path=w174) -> (string=w175:string)
      n195 = Array Subset(array=w11, index (row)=w29, index (col)=w29, length (col)=3) -> (w31:string[][])  [unwired: 1 in]
      n196 = Reshape Array(w31, w28) -> (w13:string[])
      n197 = Search 1D Array(1D array=w13, element="Vg") -> (index of element=w17:i32)  [unwired: 1 in]
      n198 = Add(x=w17, y=3) -> (x+y=w15:i32)
      n199 = Divide(x=w15, y=3) -> (x/y=w22:dbl)
      n200 = Array Subset(array=w11, index (row)=w22, index (col)=0, length (col)=1) -> (w21:string[][])  [unwired: 1 in]
      n201 = Fract/Exp String To Number(string=w21) -> (number=w25:dbl[][])  [unwired: 3 in, 1 out]
      n202 = Array Size(array=w25) -> (size(s)=w12:i32[])
      n203 = Index Array(array=w12, index=0) -> (element=w23:i32)
      n204 = Decrement(x=w23) -> (x-1=w26:i32)
      n205 = Reshape Array(w25, w26) -> (w10:dbl[])
      n206 = local write "Data Length"(w26) -> ()
      n207 = local write "Vg Column"(w10) -> ()
      n208 = Index Array(array=w170, index=w172) -> (element=w137:string)
      n209 = Empty String/Path?(string/path=w137) -> (empty?=w138:bool)
      n210 = Concatenate Strings(w175, "\\", w137) -> (w176:string)
      n211 = String To Path(string=w176) -> (path=w136:path)
      n212 = Select(t=w134, s=w138, f=w136) -> (s? t:f=w135:path)
      n213 = call "Vision Acquisition2"("Image Path"=w135) -> ("Image Out"=w169:T2)  [unwired: 25 in, 1 out]
      n214 = local write "Image File"(w135) -> ()
      n215 = local write "Image Out"(w169) -> ()
      n216 = local write "Image Out 2"(w169) -> ()
      n217 = Array Max & Min(array=w10) -> (max value=w9:dbl, min value=w8:dbl)  [unwired: 2 out]
      n218 = local write "Image Name"(w137) -> ()
      n219 = property on="Sat-Trans Slider" class="Slide (strict)"("Scale.Maximum"=w9, "Scale.Minimum"=w8) -> ()  [unwired: 2 in, 2 out]
    }
    frame #2 {
      n220 = while {
        stop <- w551 stop-if-true
        w501 = FALSE
        w499 = 0
        n221 = disable-structure shown="Disabled" {
          frame Disabled {
            w585 = "/"
            n222 = local read "Date Recorded"() -> (w588:string)
            n223 = local read "Ramp (s):"() -> (w555:dbl)
            n224 = local read "RPM:"() -> (w556:dbl)
            n225 = Divide(x=w556, y=w555) -> (x/y=w554:dbl)
            n226 = Match Pattern(string=w588, regular expression=w585) -> (before substring=w579:string, after substring=w586:string)  [unwired: 1 in, 2 out]
            n227 = local write "Accel (RPM/s):"(w554) -> ()
            n228 = String Length(string=w579) -> (length=w582:i32)
            n229 = Match Pattern(string=w586, regular expression=w585) -> (before substring=w573:string, after substring=w584:string)  [unwired: 1 in, 2 out]
            n230 = Equal?(x=w582, y=2) -> (x = y?=w580:bool)
            n231 = String Length(string=w573) -> (length=w575:i32)
            n232 = case shown="False" w580 {
              tunnel: w579 -> [w625 w627]
              tunnel: [w624 w627] -> w578
              frame False {
                n233 = Concatenate Strings("0", w625) -> (w624:string)
              }
              frame True {
              }
            }
            n234 = Equal?(x=w575, y=2) -> (x = y?=w577:bool)
            n235 = case shown="False" w577 {
              tunnel: w573 -> [w621 w623]
              tunnel: [w620 w623] -> w574
              frame False {
                n236 = Concatenate Strings("0", w621) -> (w620:string)
              }
              frame True {
              }
            }
            n237 = local read "Index"() -> (w558:string)
            n238 = local read "Index"() -> (w572:string)
            n239 = local read "Wait Time (s):"() -> (w618:dbl)
            n240 = String Subset(string=w558, length (rest)=1) -> (substring=w613:string)  [unwired: 1 in]
            n241 = local write "Row"(w613) -> ()
            n242 = local read "Treatment Concentration (mM):"() -> (w566:dbl)
            n243 = local read "Rec: Concentration"() -> (w553:dbl)
            n244 = local read "Relative Humidity (%):"() -> (w563:dbl)
            n245 = String Subset(string=w558, offset (0)=1, length (rest)=2) -> (substring=w614:string)
            n246 = Number To Decimal String(number=w618) -> (decimal integer string=w619:string)  [unwired: 1 in]
            n247 = local read "Solution Temp (C):"() -> (w607:dbl)
            n248 = local read "Surface Treatment:"() -> (w565:string)
            n249 = local read "Room Temp (F):"() -> (w611:dbl)
            n250 = local read "Rec: Material"() -> (w561:string)
            n251 = local write "Column"(w614) -> ()
            n252 = local read "New: Length"() -> (w571:dbl)
            n253 = local read "New: Width"() -> (w570:dbl)
            n254 = local read "New: Mobility-Sat"() -> (w600:dbl)
            n255 = local read "Accel (RPM/s):"() -> (w598:dbl)
            n256 = local read "Sample #:"() -> (w590:dbl)
            n257 = local read "# Drops*:"() -> (w608:dbl)
            n258 = local read "Ramp (s):"() -> (w616:dbl)
            n259 = local read "New: STS"() -> (w592:dbl)
            n260 = local read "Rec: Solvent"() -> (w567:string)
            n261 = local read "New: VT-Sat"() -> (w594:dbl)
            n262 = local read "Rec: On/Off"() -> (w596:dbl)
            n263 = local read "Rec: Method"() -> (w591:string)
            n264 = local read "Time (s):"() -> (w603:dbl)
            n265 = local read "Date Recorded"() -> (w587:string)
            n266 = local read "RPM:"() -> (w604:dbl)
            n267 = local read "Fabricator:"() -> (w612:string)
            n268 = Number To Decimal String(number=w553) -> (decimal integer string=w552:string)  [unwired: 1 in]
            n269 = Number To Decimal String(number=w608) -> (decimal integer string=w609:string)  [unwired: 1 in]
            n270 = Number To Decimal String(number=w590) -> (decimal integer string=w583:string)  [unwired: 1 in]
            n271 = call "DeviceID"("Sample"=w583, "Year"=w584, "Month"=w578, "Day"=w574, "Index"=w572) -> ("Result"=w589:string)  [unwired: 9 in, 1 out]
            n272 = Number To Decimal String(number=w571) -> (decimal integer string=w569:string)  [unwired: 1 in]
            n273 = Number To Decimal String(number=w570) -> (decimal integer string=w568:string)  [unwired: 1 in]
            n274 = Number To Decimal String(number=w607) -> (decimal integer string=w606:string)  [unwired: 1 in]
            n275 = Number To Decimal String(number=w563) -> (decimal integer string=w562:string)  [unwired: 1 in]
            n276 = Number To Decimal String(number=w611) -> (decimal integer string=w610:string)  [unwired: 1 in]
            n277 = Number To Decimal String(number=w566) -> (decimal integer string=w564:string)  [unwired: 1 in]
            n278 = Number To Decimal String(number=w604) -> (decimal integer string=w605:string)  [unwired: 1 in]
            n279 = Number To Fractional String(number=w598) -> (F-format string=w599:string)  [unwired: 3 in]
            n280 = Number To Decimal String(number=w603) -> (decimal integer string=w602:string)  [unwired: 1 in]
            n281 = Number To Fractional String(number=w600) -> (F-format string=w601:string)  [unwired: 3 in]
            n282 = Number To Fractional String(number=w596) -> (F-format string=w597:string)  [unwired: 3 in]
            n283 = Number To Fractional String(number=w594) -> (F-format string=w595:string)  [unwired: 3 in]
            n284 = Number To Fractional String(number=w592) -> (F-format string=w593:string)  [unwired: 3 in]
            n285 = Number To Decimal String(number=w616) -> (decimal integer string=w617:string)  [unwired: 1 in]
            n286 = Build Array(w589, w612, w591, w587, w583, w613, w614, w569, w568, w561, w565, w564, w567, w552, w606, w609, w619, w610, w562, w617, w605, w599, w602, w601, w597, w595, w593) -> (w615:string[])
            n287 = local write "Current \nRecord"(w615) -> ()
          }
          frame Enabled {
          }
        }
        n288 = local read "Lin-Vg Array-Used"() -> (w469:dbl[])
        n289 = local read "Sat Id-Log-Used"() -> (w473:dbl[])
        n290 = local read "New: Dielectric"() -> (w466:dbl)
        n291 = local read "Vg Array-Log-Used"() -> (w472:dbl[])
        n292 = local read "New: Length"() -> (w468:dbl)
        n293 = local read "New: Width"() -> (w465:dbl)
        n294 = local read "Lin Id-Used"() -> (w470:dbl[])
        n295 = local read "New: Dielectric"() -> (w462:dbl)
        n296 = local read "Lin Vd"() -> (w464:dbl)
        n297 = local read "Sat Vg Array-Used"() -> (w475:dbl[])
        n298 = local read "New: Dielectric"() -> (w460:dbl)
        n299 = local read "New: Length"() -> (w476:dbl)
        n300 = local read "New: Width"() -> (w478:dbl)
        n301 = local read "Sat Id-Used"() -> (w474:dbl[])
        n302 = call "Mobility-Vt-Used Pts_Linear.vi"("Width"=w465, "Length"=w468, "Vd"=w464, "Dielectric (d)"=w466, "Sat Id Used"=w470, "Vg Used"=w469) -> ("Vt"=w471:dbl, "Mobility"=w467:dbl)  [unwired: 3 in, 1 out]
        n303 = call "STS-Used.vi"("Id Used"=w473, "Vg-Used"=w472) -> ("STS"=w463:dbl)  [unwired: 9 in]
        n304 = local write "New: Mobility-Lin"(w467) -> ()
        n305 = local write "New: VT-Lin"(w471) -> ()
        n306 = call "Mobility-Vt-Used Pts_Saturation.vi"("Width"=w478, "Length"=w476, "Dielectric (d)"=w460, "Sat Id Used"=w474, "Vg Used"=w475) -> ("Vt"=w461:dbl, "Mobility"=w477:dbl)  [unwired: 4 in, 1 out]
        n307 = local write "New: STS"(w463) -> ()
        n308 = local write "New: Mobility-Sat"(w477) -> ()
        n309 = local write "New: VT-Sat"(w461) -> ()
        n310 = call "Trap Density_VT.vi"("VT"=w461, "Dielectric"=w460) -> ("Trap Density-VT"=w459:dbl)
        n311 = local read "Manual-Temp"() -> (w456:bool)
        n312 = local read "Rec: Temp"() -> (w457:dbl)
        n313 = local write "New: Trap Density-VT"(w459) -> ()
        n314 = case shown="False" w456 {
          tunnel: w457 -> [w637 _]
          tunnel: [w634 w641] -> w455
          frame False {
            n315 = local read "Rec: Temp"() -> (w635:dbl)
            n316 = property on="New: Temp" class="DigNum (strict)"("DisabledEnum"=1) -> ()  [unwired: 2 in, 2 out]
            n317 = Equal To 0?(x=w635) -> (x = 0?=w636:bool)
            n318 = local write "New: Temp"(w637) -> ()
            n319 = case shown="True" w636 {
              tunnel: [w638 w639] -> w634
              tunnel: w635 -> [w638 _]
              frame False {
              }
              frame True {
                n320 = local read "Room Temp"() -> (w639:dbl)
              }
            }
            n321 = local write "New: Temp"(w634) -> ()
          }
          frame True {
            n322 = property on="New: Temp" class="DigNum (strict)"("DisabledEnum"=0) -> ()  [unwired: 2 in, 2 out]
            n323 = local read "New: Temp"() -> (w641:dbl)
          }
        }
        n324 = call "Trap Density_STS.vi"("Temp (T) [K]"=w455, "S.T.S. (S)"=w463, "Dielectric"=w462) -> ("Trap Density (N)"=w458:dbl)  [unwired: 8 in]
        n325 = local write "New: Trap Density-STS"(w458) -> ()
        n326 = property on="Image Out" class="ImageControl"() -> ("ZoomSingle"=w519:cluster{"X":sgl, "Y":sgl})  [unwired: 2 in, 2 out]
        n327 = property on="Image Out" class="ImageControl"() -> ("Bounds"=w520:T13)  [unwired: 2 in, 2 out]
        n328 = call <vilib>:"Intialize Keyboard.vi"() -> ("device ID"=w531:refnum<k1>)  [unwired: 10 in, 1 out]
        n329 = property on="Image Out" class="ImageControl"() -> ("Image Center Position"=w526:cluster{"X":u32, "Y":u32})  [unwired: 2 in, 2 out]
        n330 = call-poly <vilib>:"Acquire Input Data.vi"("device ID"=w531) -> ("keys pressed"=w530:T14)  [unwired: 16 in, 2 out]
        n331 = Unbundle(w520) -> ("Width"=w517:u32, "Height"=w516:u32)
        n332 = Unbundle(w519) -> ("X"=w494:sgl, "Y"=w518:sgl)
        n333 = Index Array(array=w530) -> (element=w534:T15)  [unwired: 1 in]
        n334 = event shown="[1] \"Undo Button\": Mouse Down" {
          selector: _ -> [_ _ _ _ _ _ _]
          dyn-events: _ -> [_ _ _ _ _ _ _]
          timeout: 10 -> [_ _ _ _ _ _ _]
          event "Remove Button": Mouse Down {
            w654 = 0
            n335 = event-data() -> ()  [unwired: 1 in, 7 out]
            n336 = property on="Image Out" class="ImageControl"() -> ("ROI"=w652:T12)  [unwired: 2 in, 2 out]
            n337 = Unbundle(w652) -> ("Global Rectangle"=w655:i32[], "Contours"=w657:T16)
            n338 = Reverse 1D Array(array=w655) -> (reversed array=w656:i32[])
            n339 = Reverse 1D Array(array=w657) -> (reversed array=w658:T16)
            n340 = Delete From Array(array=w656, index=w654) -> (array with subset deleted=w659:i32[])  [unwired: 1 in, 1 out]
            n341 = Delete From Array(array=w658, index=w654) -> (array with subset deleted=w660:T16)  [unwired: 1 in, 1 out]
            n342 = Reverse 1D Array(array=w659) -> (reversed array=w661:i32[])
            n343 = Reverse 1D Array(array=w660) -> (reversed array=w662:T16)
            n344 = Bundle(w661, w662) -> (w653:T17)  [unwired: 1 in]
            n345 = local write "ROI Descriptor out"(w652) -> ()
            n346 = local write "ROI Descriptor"(w653) -> ()
            n347 = property on="Image Out" class="ImageControl"("ROI"=w653) -> ()  [unwired: 2 in, 2 out]
          }
          event "Undo Button": Mouse Down {
            n348 = event-data() -> ()  [unwired: 1 in, 7 out]
            n349 = invoke on="Image Out" class="ImageControl" method="Clear ROI"() -> ()  [unwired: 3 in, 3 out]
          }
          event "Image Folder": Value Change {
            n350 = event-data() -> ()  [unwired: 1 in, 5 out]
            n351 = local read "Image File"() -> (w664:path)
            n352 = call "Vision Acquisition"("Image Path"=w664) -> ("Image Out"=w663:T2)  [unwired: 25 in, 1 out]
            n353 = local write "Image Out 2"(w663) -> ()
            n354 = local write "Image Out"(w663) -> ()
            n355 = invoke on="Image Out" class="ImageControl" method="Clear ROI"() -> ()  [unwired: 3 in, 3 out]
          }
          event "Zoom": Value Change {
            n356 = event-data() -> ()  [unwired: 1 in, 5 out]
            n357 = local read "Zoom"() -> (w665:i16)
            n358 = Bundle("Zoom"=w665, "Zoom"=w665) -> (w666:cluster{"Zoom":i16, "Zoom":i16})  [unwired: 1 in]
            n359 = property on="Image Out" class="ImageControl"("ZoomInteger"=w666) -> ()  [unwired: 2 in, 2 out]
          }
          event Timeout {
            n360 = event-data() -> ()  [unwired: 1 in, 2 out]
          }
          event "Image Out": Mouse Enter {
            (unwired) 6
            n361 = event-data() -> ()  [unwired: 1 in, 3 out]
            n362 = call "Simulate_Keyboard.vi"("Action"=0, "Virtual Key"=162) -> ()  [unwired: 7 in, 1 out]
          }
          event "Image Out": Mouse Leave {
            n363 = event-data() -> ()  [unwired: 1 in, 3 out]
            n364 = flat-sequence {
              frame #0 {
                n365 = Wait (ms)(milliseconds to wait=10) -> ()  [unwired: 1 out]
              }
              frame #1 {
                (unwired) 6
                n366 = call "Simulate_Keyboard.vi"("Action"=2, "Virtual Key"=162) -> ()  [unwired: 7 in, 1 out]
              }
            }
          }
        }
        n367 = Divide(x=w517, y=w494) -> (x/y=w507:sgl)
        n368 = Multiply(x=w507, y=0.5) -> (x*y=w513:dbl)
        n369 = Divide(x=w516, y=w518) -> (x/y=w506:sgl)
        n370 = Multiply(x=w506, y=0.5) -> (x*y=w512:dbl)
        n371 = Unbundle(w526) -> ("X"=w508:u32, "Y"=w509:u32)
        n372 = Subtract(x=w509, y=w512) -> (x-y=w510:dbl)
        n373 = Subtract(x=w508, y=w513) -> (x-y=w511:dbl)
        n374 = Add(x=w511, y=w507) -> (x+y=w525:dbl)
        n375 = Add(x=w510, y=w506) -> (x+y=w524:dbl)
        n376 = Reciprocal(x=w494) -> (1/x=w493:sgl)
        n377 = event shown="[12] \"Save Changes? 2\": Mouse Down" {
          selector: _ -> [_ _ _ _ _ _ _ _ _ _ _ _ _ _ _ _]
          dyn-events: _ -> [_ _ _ _ _ _ _ _ _ _ _ _ _ _ _ _]
          timeout: 10 -> [_ _ _ _ _ _ _ _ _ _ _ _ _ _ _ _]
          tunnel: [_ _ _ _ _ _ _ _ _ _ _ _ _ TRUE _ TRUE] -> w551
          event Timeout {
            n378 = event-data() -> ()  [unwired: 1 in, 2 out]
          }
          event "Down Button": Mouse Down {
            w951 = "\\"
            w952 = "TSP"
            w1072 = 0
            # "Transpose"
            n379 = event-data() -> ()  [unwired: 1 in, 7 out]
            n380 = local read "Transfer File"() -> (w1076:path)
            n381 = Strip Path(path=w1076) -> (stripped path=w942:path, name=w1084:string)
            n382 = local write "Transfer Folder"(w942) -> ()
            n383 = property on="Image Out" class="ImageControl"() -> (error out=w1029:errorcluster, "Image Center Position"=w1033:cluster{"X":u32, "Y":u32})  [unwired: 2 in, 1 out]
            n384 = Strip Path(path=w942) -> (stripped path=w947:path)  [unwired: 1 out]
            n385 = List Folder(path=w942) -> (filenames=w1081:string[], error out=w1026:errorcluster)  [unwired: 3 in, 2 out]
            n386 = Path To String(path=w947) -> (string=w950:string)
            n387 = invoke on="Image Out" class="ImageControl" method="Clear ROI"() -> ()  [unwired: 3 in, 3 out]
            n388 = local read "Folder Index"() -> (w1028:dbl)
            n389 = Array Size(array=w1081) -> (size(s)=w1077:i32)
            n390 = Search 1D Array(1D array=w1081, element=w1084) -> (index of element=w1078:i32)  [unwired: 1 in]
            n391 = Unbundle(w1033) -> ("X"=w1031:u32)  [unwired: 1 out]
            n392 = Decrement(x=w1077) -> (x-1=w1079:i32)
            n393 = Equal?(x=w1078, y=w1079) -> (x = y?=w1080:bool)
            n394 = local read "Folder Index"() -> (w965:dbl)
            n395 = case shown="False" w1080 {
              tunnel: w1028 -> [w1248 _]
              tunnel: [w1247 0] -> w1027
              tunnel: w1026 -> [w1246 w1249]
              tunnel: [w1246 w1249] -> w1025
              frame False {
                n396 = Increment(x=w1248) -> (x+1=w1247:dbl)
              }
              frame True {
              }
            }
            n397 = local write "Folder Index"(w1027) -> ()
            n398 = Bundle("X"=w1031, 0) -> (w1032:cluster{"X":u32, i32})  [unwired: 1 in]
            n399 = property on="Image Out" class="ImageControl"(error in=w1029, "Image Center Position"=w1032) -> ()  [unwired: 1 in, 2 out]
            n400 = Path To String(path=w942) -> (string=w1085:string)
            n401 = Index Array(array=w1081, index=w1027) -> (element=w943:string)
            n402 = String Subset(string=w943, offset (0)=3) -> (substring=w946:string)  [unwired: 1 in]
            n403 = Concatenate Strings(w952, w946) -> (w948:string)
            n404 = Concatenate Strings(w950, w951, w952, w951, w948) -> (w949:string)
            n405 = String To Path(string=w949) -> (path=w944:path)
            n406 = local write "Transport File"(w944) -> ()
            n407 = Strip Path(path=w944) -> (stripped path=w964:path, name=w955:string)
            n408 = local write "Transport Folder"(w964) -> ()
            n409 = List Folder(path=w964) -> (filenames=w959:string[], error out=w967:errorcluster)  [unwired: 3 in, 2 out]
            n410 = Array Size(array=w959) -> (size(s)=w963:i32)
            n411 = Search 1D Array(1D array=w959, element=w955) -> (index of element=w962:i32)  [unwired: 1 in]
            n412 = Decrement(x=w963) -> (x-1=w961:i32)
            n413 = Equal?(x=w962, y=w961) -> (x = y?=w960:bool)
            n414 = case shown="False" w960 {
              tunnel: w965 -> [w1110 _]
              tunnel: [w1109 0] -> w966
              tunnel: w967 -> [w1108 w1111]
              tunnel: [w1108 w1111] -> _
              frame False {
                n415 = Increment(x=w1110) -> (x+1=w1109:dbl)
              }
              frame True {
              }
            }
            n416 = local write "Folder Index"(w966) -> ()
            n417 = local write "Data Name:"(w943) -> ()
            n418 = Path To String(path=w964) -> (string=w954:string)
            n419 = Index Array(array=w959, index=w966) -> (element=w958:string)
            n420 = local write "Data Name:"(w958) -> ()
            n421 = Concatenate Strings(w1085, "\\", w943) -> (w1083:string)
            n422 = Concatenate Strings(w954, "\\", w958) -> (w956:string)
            n423 = String To Path(string=w1083) -> (path=w1000:path)
            n424 = call "Recorded Values.vi"("Path"=w1000) -> ("Recorded Char"=w1087:T6, "Recorded Prop"=w1088:T7, "Fabrication Prop"=w1086:T8)  [unwired: 8 in]
            n425 = Unbundle By Name(w1087) -> ("Mobility-Sat"=w1100:dbl, "Moblitity-Lin"=w1101:dbl, "On/Off"=w1102:dbl, "Off Current"=w1103:dbl, "Vt-Sat"=w995:dbl, "STS"=w1104:dbl, "Trap Density-VT"=w1105:dbl, "Trap Density-STS"=w1106:dbl)
            n426 = Unbundle By Name(w1086) -> ("Date Created"=w1107:string, "Material"=w1089:string, "Solvent"=w1090:string, "Concentration"=w1091:dbl, "Method"=w1092:string, "Dielectric (nm)"=w1093:dbl, "Treatment"=w1094:string, "Comments"=w1095:string)
            n427 = Unbundle By Name(w1088) -> ("Date Recorded"=w1096:string, "Index"=w1097:string, "Length"=w1098:dbl, "Width"=w1099:dbl, "Sample Temp"=w997:dbl)
            n428 = local write "Date Created"(w1107) -> ()
            n429 = local write "Rec: Off I-Sat"(w1103) -> ()
            n430 = local write "Rec: Comments"(w1095) -> ()
            n431 = local write "Rec: Material"(w1089) -> ()
            n432 = local write "Rec: VT-Sat"(w995) -> ()
            n433 = local write "Rec: Concentration"(w1091) -> ()
            n434 = local write "Rec: Method"(w1092) -> ()
            n435 = local write "Rec: Dielectric (d)"(w1093) -> ()
            n436 = local write "Surface Treatment:"(w1094) -> ()
            n437 = local write "Index"(w1097) -> ()
            n438 = local write "Rec: Mobility-Sat"(w1100) -> ()
            n439 = local write "Rec: Mobility-Lin"(w1101) -> ()
            n440 = local write "Rec: On/Off"(w1102) -> ()
            n441 = local write "Rec: STS"(w1104) -> ()
            n442 = local write "Rec: Trap Density-VT"(w1105) -> ()
            n443 = local write "Rec: Trap Density-STS"(w1106) -> ()
            n444 = local write "Rec: Solvent"(w1090) -> ()
            n445 = local write "Date Recorded"(w1096) -> ()
            n446 = local write "Rec: Length"(w1098) -> ()
            n447 = local write "Rec: Width"(w1099) -> ()
            n448 = local write "Rec: Temp"(w997) -> ()
            n449 = Equal To 0?(x=w997) -> (x = 0?=w998:bool)
            n450 = case shown="True" w998 {
              tunnel: [w1119 w1120] -> w996
              tunnel: w997 -> [w1119 _]
              frame False {
              }
              frame True {
                n451 = local read "Room Temp"() -> (w1120:dbl)
              }
            }
            n452 = String To Path(string=w956) -> (path=w953:path)
            n453 = local read "NumPoints Log"() -> (w1021:dbl)
            n454 = local write "Transfer File"(w1000) -> ()
            n455 = local read "Num Pts"() -> (w1024:dbl)
            n456 = Strip Path(path=w953) -> ()  [unwired: 2 out]
            n457 = call-poly <vilib>:"Read From Spreadsheet File.vi"("file path (dialog if empty)"=w953) -> ("all rows"=w981:string[][])  [unwired: 6 in, 4 out]
            n458 = Array Size(array=w981) -> (size(s)=w987:i32[])
            n459 = call-poly <vilib>:"Read From Spreadsheet File.vi"("file path (dialog if empty)"=w1000) -> ("all rows"=w925:string[][])  [unwired: 6 in, 4 out]
            n460 = call "Mobility-Vt Calculator-File.vi"("NumPts"=w1024, "Path"=w1000) -> ("Graph Cluster"=w993:T9, "Output"=w1023:T10, "Index-Sat"=w1022:dbl, "Index-Lin"=w1008:dbl)  [unwired: 5 in, 1 out]
            n461 = local read "New: Dielectric"() -> (w1005:dbl)
            n462 = call "STS Calculator-File.vi"("NumPts"=w1021, "Path"=w1000) -> ("STS Index-Sat"=w1020:dbl, "XY Graph-Sat"=w1019:cluster{dbl[], dbl[]}[], "Ouput"=w1018:cluster{"STS-Sat":dbl, "STS-Lin":dbl})  [unwired: 5 in, 2 out]
            n463 = local write "Index 2"(w1020) -> ()
            n464 = Array Subset(array=w981, length (col)=1) -> (w983:string[][])  [unwired: 3 in]
            n465 = Index Array(array=w987, index=0) -> (element=w976:i32)
            n466 = local write "Sat-Trans Slider"(w1022) -> ()
            n467 = Array Size(array=w925) -> (size(s)=w1073:i32[])
            n468 = Unbundle By Name(w1023) -> ("Mobility-Sat"=w1017:dbl, "Vt-Sat"=w1004:dbl, "Mobility-Lin"=w1016:dbl, "Vt-Lin"=w1015:dbl, "Off I-Sat"=w1001:dbl, "On/Off I-Sat"=w994:dbl)
            n469 = Unbundle By Name(w1018) -> ("STS-Sat"=w999:dbl)  [unwired: 1 out]
            n470 = Reshape Array(w983, w976) -> (w982:string[])
            n471 = local write "MobVi Index"(w1022) -> ()
            n472 = local write "Sat-Log"(w1019) -> ()
            n473 = Search 1D Array(1D array=w982, element="Vd") -> (index of element=w980:i32)  [unwired: 1 in]
            n474 = Unbundle By Name(w993) -> ("Raw Sat"=w990:cluster{dbl[], dbl[]}[], "Sqrt Sat"=w992:cluster{dbl[], dbl[]}[], "Raw Lin"=w989:cluster{dbl[], dbl[]}[], "Sqrt Lin"=w991:cluster{dbl[], dbl[]}[], "Log Lin"=w988:cluster{dbl[], dbl[]}[])  [unwired: 1 out]
            n475 = local write "Sqrt-Sat"(w992) -> ()
            n476 = call "Trap Density_VT.vi"("VT"=w1004, "Dielectric"=w1005) -> ("Trap Density-VT"=w1003:dbl)
            n477 = Index Array(array=w1073, index=0) -> (element=w1057:i32)
            n478 = call "Trap Density_STS.vi"("Temp (T) [K]"=w996, "S.T.S. (S)"=w999, "Dielectric"=w1005) -> ("Trap Density (N)"=w1002:dbl)  [unwired: 8 in]
            n479 = local write "New: STS"(w999) -> ()
            n480 = local write "Calc: STS"(w999) -> ()
            n481 = Increment(x=w980) -> (x+1=w979:i32)
            n482 = Array Subset(array=w981, index (row)=w979) -> (w977:string[][])  [unwired: 3 in]
            n483 = Fract/Exp String To Number(string=w977, default (0 dbl)="default (0 dbl) 3") -> (number=w969:ext[][])  [unwired: 2 in, 1 out]
            n484 = local write "Calc: Mobility-Sat"(w1017) -> ()
            n485 = local write "Calc: Off I-Sat"(w1015) -> ()
            n486 = local write "Calc: Mobility-Lin"(w1016) -> ()
            n487 = Decimate 1D Array(w1019) -> (w1052:cluster{dbl[], dbl[]}[])  [unwired: 1 out]
            n488 = Decimate 1D Array(w992) -> (w1060:cluster{dbl[], dbl[]}[])  [unwired: 1 out]
            n489 = local write "Calc: Off I-Sat"(w1001) -> ()
            n490 = local write "Calc: On/Off"(w994) -> ()
            n491 = Decimate 1D Array(w991) -> (w1014:cluster{dbl[], dbl[]}[])  [unwired: 1 out]
            n492 = local write "Calc: VT-Sat"(w1004) -> ()
            n493 = Array Subset(array=w925, index (row)=w1072, index (col)=w1072, length (col)=3) -> (w1074:string[][])  [unwired: 1 in]
            n494 = Delete From Array(array=w969) -> (array with subset deleted=w968:ext[][])  [unwired: 3 in, 1 out]
            n495 = local write "Calc: Trap Density-VT"(w1003) -> ()
            n496 = local write "Calc: Trap Density-STS"(w1002) -> ()
            n497 = local write "New: Trap Density-STS"(w1002) -> ()
            n498 = local write "New: Trap Density-VT"(w1003) -> ()
            n499 = Array To Cluster(array=w1052) -> (cluster=w1050:T11)
            n500 = Array To Cluster(array=w1060) -> (cluster=w1062:T11)
            n501 = local write "Raw- Sat"(w990) -> ()
            n502 = local write "Sqrt-Lin"(w991) -> ()
            n503 = Delete From Array(array=w968, index (col)=0 ("Deaktivierter Index (Spalte)")) -> (deleted portion=w973:ext[], array with subset deleted=w974:ext[][])  [unwired: 2 in]
            n504 = local write "Raw- Lin"(w989) -> ()
            n505 = local write "New: VT-Lin"(w1015) -> ()
            n506 = local write "Log-Lin"(w988) -> ()
            n507 = local write "New: VT-Sat"(w1004) -> ()
            n508 = local write "New: Mobility-Sat"(w1017) -> ()
            n509 = Transpose 2D Array(2D array=w974) -> (transposed array=w975:ext[][])
            n510 = local write "New: Mobility-Lin"(w1016) -> ()
            n511 = Reshape Array(w1074, w1057) -> (w927:string[])
            n512 = Search 1D Array(1D array=w927, element="Vg") -> (index of element=w931:i32)  [unwired: 1 in]
            n513 = Add(x=w931, y=3) -> (x+y=w929:i32)
            n514 = Divide(x=w929, y=3) -> (x/y=w936:dbl)
            n515 = Array Subset(array=w925, index (row)=w936, index (col)=0, length (col)=1) -> (w935:string[][])  [unwired: 1 in]
            n516 = Fract/Exp String To Number(string=w935) -> (number=w939:dbl[][])  [unwired: 3 in, 1 out]
            n517 = Array Size(array=w939) -> (size(s)=w926:i32[])
            n518 = Index Array(array=w926, index=0) -> (element=w937:i32)
            n519 = Decrement(x=w937) -> (x-1=w940:i32)
            n520 = Reshape Array(w939, w940) -> (w924:dbl[])
            n521 = local write "Data Length"(w940) -> ()
            n522 = local write "Vg Column"(w924) -> ()
            n523 = Array To Cluster(array=w1014) -> (cluster=w1013:T11)
            n524 = for {
              tunnel: w973 -> [w1117]
              tunnel: w975 -> [w1118] mode=indexing
              tunnel: [w1116] -> w971 mode=indexing
              n525 = Bundle(w1117, w1118) -> (w1116:cluster{ext[], ext[]})  [unwired: 1 in]
            }
            n526 = Array Max & Min(array=w924) -> (max value=w923:dbl, min value=w922:dbl)  [unwired: 2 out]
            n527 = Unbundle(w1050) -> ("[0]"=w1051:cluster{dbl[], dbl[]})  [unwired: 8 out]
            n528 = Unbundle(w1062) -> ("[0]"=w1061:cluster{dbl[], dbl[]})  [unwired: 8 out]
            n529 = Unbundle(w1013) -> ("[0]"=w1010:cluster{dbl[], dbl[]})  [unwired: 8 out]
            n530 = Search 1D Array(1D array=w927, element="Index:") -> (index of element=w1069:i32)  [unwired: 1 in]
            n531 = local write "Transport"(w971) -> ()
            n532 = property on="Sat-Trans Slider" class="Slide (strict)"("Scale.Maximum"=w923, "Scale.Minimum"=w922) -> ()  [unwired: 2 in, 2 out]
            n533 = Array Size(array=w971) -> (size(s)=w970:i32)
            n534 = local read "Num Pts"() -> (w1009:dbl)
            n535 = Unbundle(w1010) -> (w1012:dbl[], w1011:dbl[])
            n536 = for {
              N: w970 -> [_]
              i -> [w1115]
              n537 = local read "Transport Line Color"() -> (w1114:u32)
              n538 = local read "Ring"() -> (w1113:u16)
              n539 = property on="Transport" class="XYGraph (strict)"("Active Plot"=w1115, "Plot.Plot Color"=w1114, "Plot.Line Width"=w1113) -> ()  [unwired: 2 in, 2 out]
            }
            n540 = Increment(x=w1069) -> (x+1=w1070:i32)
            n541 = Unbundle(w1051) -> (w1049:dbl[], w1048:dbl[])
            n542 = Unbundle(w1061) -> (w1054:dbl[], w1053:dbl[])
            n543 = Array Subset(array=w1012, index=w1008, length=w1009) -> (w1007:dbl[])
            n544 = Array Subset(array=w1011, index=w1008, length=w1009) -> (w1006:dbl[])
            n545 = Array Subset(array=w1049, index=w1020, length=w1021) -> (w1056:dbl[])
            n546 = Array Subset(array=w1048, index=w1020, length=w1021) -> (w1055:dbl[])
            n547 = Array Subset(array=w1054, index=w1022, length=w1024) -> (w1059:dbl[])
            n548 = Array Subset(array=w1053, index=w1022, length=w1024) -> (w1058:dbl[])
            n549 = Index Array(array=w927, index=w1070) -> (element=w1037:string)
            n550 = local write "Lin-Vg Array-Used"(w1007) -> ()
            n551 = local write "Sat Vg Array-Used"(w1059) -> ()
            n552 = local write "Vg Array-Log-Used"(w1055) -> ()
            n553 = local write "Lin Id-Used"(w1006) -> ()
            n554 = local read "Image Folder"() -> (w1035:path)
            n555 = local write "Sat Id-Used"(w1058) -> ()
            n556 = local write "Sat Id-Log-Used"(w1056) -> ()
            n557 = List Folder(path=w1035, error in=w1025) -> (filenames=w1068:string[], error out=w1038:errorcluster)  [unwired: 2 in, 2 out]
            n558 = while {
              tunnel: w1068 -> [w1133]
              tunnel: w1037 -> [w1131]
              tunnel: [w1130] -> _
              tunnel: [w1130] -> w1067
              tunnel: w1057 -> [w1129]
              i -> [w1130]
              stop <- w1126 stop-if-true
              n559 = Index Array(array=w1133, index=w1130) -> (element=w1134:string)
              n560 = xnode "Match Regular Expression"("input string"=w1134, "regular expression"=w1131) -> ("whole match"=w1132:string)  [unwired: 4 in, 4 out]
              n561 = Equal?(x=w1132, y=w1131) -> (x = y?=w1128:bool)
              n562 = Equal?(x=w1129, y=w1130) -> (x = y?=w1127:bool)
              n563 = Or(x=w1128, y=w1127) -> (x .or. y?=w1126:bool)
            }
            n564 = Build Path(base path=w1035, name or relative path="ROI") -> (appended path=w1034:path)
            n565 = Path To String(path=w1035) -> (string=w1065:string)
            n566 = Index Array(array=w1068, index=w1067) -> (element=w1046:string)
            n567 = invoke on="Image Out" class="ImageControl" method="Clear ROI"(error in=w1038) -> (error out=w1041:errorcluster)  [unwired: 2 in, 2 out]
            n568 = local write "Image Name"(w1046) -> ()
            n569 = Build Path(base path=w1034, name or relative path=w1037) -> (appended path=w1042:path)
            n570 = call <vilib>:"Check if File or Folder Exists.vi"("error in (no error)"=w1041, "path"=w1042) -> ("file or folder exists?"=w1039:bool, "dup path"=w1040:path)  [unwired: 7 in, 1 out]
            n571 = Concatenate Strings(w1065, "\\", w1046) -> (w1064:string)
            n572 = case shown="False" w1039 {
              tunnel: w1040 -> [_ w1121]
              frame False {
              }
              frame True {
                n573 = Read from Text File(file (use dialog)=w1121) -> (text=w1125:string)  [unwired: 3 in, 3 out]
                n574 = property on="Image Out" class="ImageControl"() -> ("ROI"=w1122:T12)  [unwired: 2 in, 2 out]
                n575 = Unflatten From String(type=w1122, binary string=w1125) -> (value=w1123:T12, error out=w1124:errorcluster)  [unwired: 3 in, 1 out]
                n576 = property on="Image Out" class="ImageControl"(error in=w1124, "ROI"=w1123) -> ()  [unwired: 1 in, 2 out]
              }
            }
            n577 = String To Path(string=w1064) -> (path=w1045:path)
            n578 = Empty String/Path?(string/path=w1046) -> (empty?=w1047:bool)
            n579 = local read "No Image File"() -> (w1043:path)
            n580 = Select(t=w1043, s=w1047, f=w1045) -> (s? t:f=w1044:path)
            n581 = local write "Image File"(w1044) -> ()
            n582 = call "Vision Acquisition4"("Image Path"=w1044) -> ("Image Out"=w1066:T2)  [unwired: 25 in, 1 out]
            n583 = local write "Image Out"(w1066) -> ()
            n584 = local write "Image Out 2"(w1066) -> ()
          }
          event "Transfer File": Value Change {
            w1273 = 0
            w1287 = "\\"
            w1288 = "TSP"
            w1423 = 0
            # "Transpose"
            n585 = event-data() -> ()  [unwired: 1 in, 5 out]
            n586 = local read "Transfer File"() -> (w1419:path)
            n587 = Strip Path(path=w1419) -> (stripped path=w1278:path, name=w1431:string)
            n588 = local write "Transfer Folder"(w1278) -> ()
            n589 = property on="Image Out" class="ImageControl"() -> (error out=w1377:errorcluster, "Image Center Position"=w1381:cluster{"X":u32, "Y":u32})  [unwired: 2 in, 1 out]
            n590 = List Folder(path=w1278) -> (filenames=w1428:string[], error out=w1387:errorcluster)  [unwired: 3 in, 2 out]
            n591 = Strip Path(path=w1278) -> (stripped path=w1283:path)  [unwired: 1 out]
            n592 = Search 1D Array(1D array=w1428, element=w1431) -> (index of element=w1376:i32)  [unwired: 1 in]
            n593 = Path To String(path=w1283) -> (string=w1286:string)
            n594 = local write "Folder Index"(w1376) -> ()
            n595 = Unbundle(w1381) -> ("X"=w1379:u32)  [unwired: 1 out]
            n596 = Path To String(path=w1278) -> (string=w1432:string)
            n597 = Index Array(array=w1428, index=w1376) -> (element=w1279:string)
            n598 = String Subset(string=w1279, offset (0)=3) -> (substring=w1282:string)  [unwired: 1 in]
            n599 = Concatenate Strings(w1288, w1282) -> (w1284:string)
            n600 = Concatenate Strings(w1286, w1287, w1288, w1287, w1284) -> (w1285:string)
            n601 = Bundle("X"=w1379, 0) -> (w1380:cluster{"X":u32, i32})  [unwired: 1 in]
            n602 = String To Path(string=w1285) -> (path=w1280:path)
            n603 = local write "Transport File"(w1280) -> ()
            n604 = Strip Path(path=w1280) -> (stripped path=w1309:path, name=w1314:string)
            n605 = local write "Transport Folder"(w1309) -> ()
            n606 = local write "Data Name:"(w1279) -> ()
            n607 = property on="Image Out" class="ImageControl"(error in=w1377, "Image Center Position"=w1380) -> ()  [unwired: 1 in, 2 out]
            n608 = List Folder(path=w1309) -> (filenames=w1310:string[])  [unwired: 3 in, 3 out]
            n609 = Search 1D Array(1D array=w1310, element=w1314) -> (index of element=w1277:i32)  [unwired: 1 in]
            n610 = Concatenate Strings(w1432, "\\", w1279) -> (w1430:string)
            n611 = String To Path(string=w1430) -> (path=w1251:path)
            n612 = call "Recorded Values.vi"("Path"=w1251) -> ("Recorded Char"=w1374:T6, "Recorded Prop"=w1373:T7, "Fabrication Prop"=w1375:T8)  [unwired: 8 in]
            n613 = Unbundle By Name(w1374) -> ("Mobility-Sat"=w1361:dbl, "Moblitity-Lin"=w1360:dbl, "On/Off"=w1359:dbl, "Off Current"=w1358:dbl, "Vt-Sat"=w1325:dbl, "STS"=w1357:dbl, "Trap Density-VT"=w1356:dbl, "Trap Density-STS"=w1355:dbl)
            n614 = Unbundle By Name(w1375) -> ("Date Created"=w1354:string, "Material"=w1372:string, "Solvent"=w1371:string, "Concentration"=w1370:dbl, "Method"=w1369:string, "Dielectric (nm)"=w1368:dbl, "Treatment"=w1367:string, "Comments"=w1366:string)
            n615 = Unbundle By Name(w1373) -> ("Date Recorded"=w1365:string, "Index"=w1364:string, "Length"=w1363:dbl, "Width"=w1362:dbl, "Sample Temp"=w1327:dbl)
            n616 = local write "Date Created"(w1354) -> ()
            n617 = local write "Rec: Material"(w1372) -> ()
            n618 = local write "Rec: Off I-Sat"(w1358) -> ()
            n619 = local write "Rec: Comments"(w1366) -> ()
            n620 = local write "Rec: VT-Sat"(w1325) -> ()
            n621 = local write "Rec: Concentration"(w1370) -> ()
            n622 = local write "Rec: Method"(w1369) -> ()
            n623 = local write "Rec: Dielectric (d)"(w1368) -> ()
            n624 = local write "Surface Treatment:"(w1367) -> ()
            n625 = local write "Index"(w1364) -> ()
            n626 = local write "Rec: Mobility-Sat"(w1361) -> ()
            n627 = local write "Rec: Mobility-Lin"(w1360) -> ()
            n628 = local write "Rec: On/Off"(w1359) -> ()
            n629 = local write "Rec: STS"(w1357) -> ()
            n630 = local write "Rec: Trap Density-VT"(w1356) -> ()
            n631 = local write "Rec: Trap Density-STS"(w1355) -> ()
            n632 = local write "Rec: Solvent"(w1371) -> ()
            n633 = local write "Date Recorded"(w1365) -> ()
            n634 = local write "Rec: Length"(w1363) -> ()
            n635 = local write "Rec: Width"(w1362) -> ()
            n636 = local write "Rec: Temp"(w1327) -> ()
            n637 = Equal To 0?(x=w1327) -> (x = 0?=w1328:bool)
            n638 = case shown="True" w1328 {
              tunnel: [w1439 w1440] -> w1326
              tunnel: w1327 -> [w1439 _]
              frame False {
              }
              frame True {
                n639 = local read "Room Temp"() -> (w1440:dbl)
              }
            }
            n640 = local write "Folder Index"(w1277) -> ()
            n641 = local read "NumPoints Log"() -> (w1350:dbl)
            n642 = local write "Transfer File"(w1251) -> ()
            n643 = local read "Num Pts"() -> (w1351:dbl)
            n644 = Path To String(path=w1309) -> (string=w1315:string)
            n645 = call-poly <vilib>:"Read From Spreadsheet File.vi"("file path (dialog if empty)"=w1251) -> ("all rows"=w1425:string[][])  [unwired: 6 in, 4 out]
            n646 = Index Array(array=w1310, index=w1277) -> (element=w1311:string)
            n647 = local read "New: Dielectric"() -> (w1334:dbl)
            n648 = call "STS Calculator-File.vi"("NumPts"=w1350, "Path"=w1251) -> ("STS Index-Sat"=w1348:dbl, "XY Graph-Sat"=w1349:cluster{dbl[], dbl[]}[], "Ouput"=w1347:cluster{"STS-Sat":dbl, "STS-Lin":dbl})  [unwired: 5 in, 2 out]
            n649 = call "Mobility-Vt Calculator-File.vi"("NumPts"=w1351, "Path"=w1251) -> ("Graph Cluster"=w1322:T9, "Output"=w1352:T10, "Index-Sat"=w1353:dbl, "Index-Lin"=w1340:dbl)  [unwired: 5 in, 1 out]
            n650 = local write "Data Name:"(w1311) -> ()
            n651 = Unbundle By Name(w1352) -> ("Mobility-Sat"=w1336:dbl, "Vt-Sat"=w1330:dbl, "Mobility-Lin"=w1335:dbl, "Vt-Lin"=w1323:dbl, "Off I-Sat"=w1329:dbl, "On/Off I-Sat"=w1324:dbl)
            n652 = local write "Index 2"(w1348) -> ()
            n653 = Unbundle By Name(w1347) -> ("STS-Sat"=w1331:dbl)  [unwired: 1 out]
            n654 = local write "MobVi Index"(w1353) -> ()
            n655 = local write "Sat-Log"(w1349) -> ()
            n656 = Concatenate Strings(w1315, "\\", w1311) -> (w1313:string)
            n657 = local write "Sat-Trans Slider"(w1353) -> ()
            n658 = Array Size(array=w1425) -> (size(s)=w1424:i32[])
            n659 = call "Trap Density_VT.vi"("VT"=w1330, "Dielectric"=w1334) -> ("Trap Density-VT"=w1333:dbl)
            n660 = call "Trap Density_STS.vi"("Temp (T) [K]"=w1326, "S.T.S. (S)"=w1331, "Dielectric"=w1334) -> ("Trap Density (N)"=w1332:dbl)  [unwired: 8 in]
            n661 = String To Path(string=w1313) -> (path=w1316:path)
            n662 = local write "Calc: Mobility-Lin"(w1335) -> ()
            n663 = local write "Calc: Mobility-Sat"(w1336) -> ()
            n664 = local write "Calc: VT-Sat"(w1330) -> ()
            n665 = local write "Calc: Off I-Sat"(w1329) -> ()
            n666 = local write "Calc: VT-Lin"(w1323) -> ()
            n667 = local write "Calc: On/Off"(w1324) -> ()
            n668 = local write "Calc: STS"(w1331) -> ()
            n669 = Strip Path(path=w1316) -> ()  [unwired: 2 out]
            n670 = Unbundle By Name(w1322) -> ("Raw Sat"=w1319:cluster{dbl[], dbl[]}[], "Sqrt Sat"=w1320:cluster{dbl[], dbl[]}[], "Raw Lin"=w1318:cluster{dbl[], dbl[]}[], "Sqrt Lin"=w1321:cluster{dbl[], dbl[]}[], "Log Lin"=w1317:cluster{dbl[], dbl[]}[])  [unwired: 1 out]
            n671 = call-poly <vilib>:"Read From Spreadsheet File.vi"("file path (dialog if empty)"=w1316) -> ("all rows"=w1295:string[][])  [unwired: 6 in, 4 out]
            n672 = Decimate 1D Array(w1321) -> (w1346:cluster{dbl[], dbl[]}[])  [unwired: 1 out]
            n673 = local write "Calc: Trap Density-VT"(w1333) -> ()
            n674 = local write "Calc: Trap Density-STS"(w1332) -> ()
            n675 = local write "New: Trap Density-STS"(w1332) -> ()
            n676 = local write "New: Trap Density-VT"(w1333) -> ()
            n677 = local write "Sqrt-Lin"(w1321) -> ()
            n678 = Array Size(array=w1295) -> (size(s)=w1289:i32[])
            n679 = local write "New: VT-Sat"(w1330) -> ()
            n680 = Decimate 1D Array(w1349) -> (w1402:cluster{dbl[], dbl[]}[])  [unwired: 1 out]
            n681 = Index Array(array=w1424, index=w1423) -> (element=w1406:i32)
            n682 = Decimate 1D Array(w1320) -> (w1409:cluster{dbl[], dbl[]}[])  [unwired: 1 out]
            n683 = local write "Sqrt-Sat"(w1320) -> ()
            n684 = local write "New: Mobility-Lin"(w1335) -> ()
            n685 = Array Subset(array=w1425, index (row)=w1423, index (col)=w1423, length (col)=3) -> (w1426:string[][])  [unwired: 1 in]
            n686 = local write "New: VT-Lin"(w1323) -> ()
            n687 = Array To Cluster(array=w1346) -> (cluster=w1345:T11)
            n688 = local write "New: STS"(w1331) -> ()
            n689 = local write "New: Mobility-Sat"(w1336) -> ()
            n690 = Array Subset(array=w1295, length (col)=1) -> (w1293:string[][])  [unwired: 3 in]
            n691 = Index Array(array=w1289, index=0) -> (element=w1300:i32)
            n692 = Array To Cluster(array=w1402) -> (cluster=w1400:T11)
            n693 = Array To Cluster(array=w1409) -> (cluster=w1411:T11)
            n694 = Reshape Array(w1426, w1406) -> (w1412:string[])
            n695 = local write "Raw- Sat"(w1319) -> ()
            n696 = Unbundle(w1345) -> ("[0]"=w1344:cluster{dbl[], dbl[]})  [unwired: 8 out]
            n697 = Reshape Array(w1293, w1300) -> (w1294:string[])
            n698 = local write "Raw- Lin"(w1318) -> ()
            n699 = local read "Num Pts"() -> (w1341:dbl)
            n700 = local write "Log-Lin"(w1317) -> ()
            n701 = Unbundle(w1344) -> (w1343:dbl[], w1342:dbl[])
            n702 = Unbundle(w1400) -> ("[0]"=w1401:cluster{dbl[], dbl[]})  [unwired: 8 out]
            n703 = Unbundle(w1411) -> ("[0]"=w1410:cluster{dbl[], dbl[]})  [unwired: 8 out]
            n704 = Search 1D Array(1D array=w1294, element="Vd") -> (index of element=w1296:i32)  [unwired: 1 in]
            n705 = Search 1D Array(1D array=w1412, element="Index:") -> (index of element=w1420:i32)  [unwired: 1 in]
            n706 = local read "Num Pts"() -> (w1337:dbl)
            n707 = Increment(x=w1296) -> (x+1=w1297:i32)
            n708 = Array Subset(array=w1295, index (row)=w1297) -> (w1299:string[][])  [unwired: 3 in]
            n709 = Array Subset(array=w1343, index=w1340, length=w1341) -> (w1339:dbl[])
            n710 = Array Subset(array=w1342, index=w1340, length=w1341) -> (w1338:dbl[])
            n711 = Increment(x=w1420) -> (x+1=w1421:i32)
            n712 = Unbundle(w1401) -> (w1398:dbl[], w1397:dbl[])
            n713 = Unbundle(w1410) -> (w1399:dbl[], w1403:dbl[])
            n714 = Fract/Exp String To Number(string=w1299, default (0 dbl)="default (0 dbl) 5") -> (number=w1307:ext[][])  [unwired: 2 in, 1 out]
            n715 = Delete From Array(array=w1307) -> (array with subset deleted=w1308:ext[][])  [unwired: 3 in, 1 out]
            n716 = local read "Image Folder"() -> (w1383:path)
            n717 = Delete From Array(array=w1308, index (col)=0 ("Deaktivierter Index (Spalte)")) -> (deleted portion=w1303:ext[], array with subset deleted=w1302:ext[][])  [unwired: 2 in]
            n718 = local write "Lin-Vg Array-Used"(w1339) -> ()
            n719 = Array Subset(array=w1398, index=w1348, length=w1350) -> (w1405:dbl[])
            n720 = Array Subset(array=w1397, index=w1348, length=w1350) -> (w1404:dbl[])
            n721 = Array Subset(array=w1399, index=w1353, length=w1337) -> (w1408:dbl[])
            n722 = Array Subset(array=w1403, index=w1353, length=w1337) -> (w1407:dbl[])
            n723 = Index Array(array=w1412, index=w1421) -> (element=w1385:string)
            n724 = local write "Lin Id-Used"(w1338) -> ()
            n725 = Transpose 2D Array(2D array=w1302) -> (transposed array=w1301:ext[][])
            n726 = local write "Sat Vg Array-Used"(w1408) -> ()
            n727 = local write "Vg Array-Log-Used"(w1404) -> ()
            n728 = for {
              tunnel: w1303 -> [w1437]
              tunnel: w1301 -> [w1438] mode=indexing
              tunnel: [w1436] -> w1305 mode=indexing
              n729 = Bundle(w1437, w1438) -> (w1436:cluster{ext[], ext[]})  [unwired: 1 in]
            }
            n730 = local write "Sat Id-Log-Used"(w1405) -> ()
            n731 = local write "Sat Id-Used"(w1407) -> ()
            n732 = local write "Index"(w1385) -> ()
            n733 = List Folder(path=w1383, error in=w1387) -> (filenames=w1417:string[], error out=w1386:errorcluster)  [unwired: 2 in, 2 out]
            n734 = Build Path(base path=w1383, name or relative path="ROI") -> (appended path=w1382:path)
            n735 = local write "Transport"(w1305) -> ()
            n736 = Array Size(array=w1305) -> (size(s)=w1306:i32)
            n737 = invoke on="Image Out" class="ImageControl" method="Clear ROI"(error in=w1386) -> (error out=w1390:errorcluster)  [unwired: 2 in, 2 out]
            n738 = Build Path(base path=w1382, name or relative path=w1385) -> (appended path=w1391:path)
            n739 = while {
              tunnel: w1417 -> [w1453]
              tunnel: w1385 -> [w1451]
              tunnel: [w1450] -> _
              tunnel: [w1450] -> w1416
              tunnel: w1406 -> [w1449]
              i -> [w1450]
              stop <- w1446 stop-if-true
              n740 = Index Array(array=w1453, index=w1450) -> (element=w1454:string)
              n741 = xnode "Match Regular Expression"("input string"=w1454, "regular expression"=w1451) -> ("whole match"=w1452:string)  [unwired: 4 in, 4 out]
              n742 = Equal?(x=w1452, y=w1451) -> (x = y?=w1448:bool)
              n743 = Equal?(x=w1449, y=w1450) -> (x = y?=w1447:bool)
              n744 = Or(x=w1448, y=w1447) -> (x .or. y?=w1446:bool)
            }
            n745 = for {
              N: w1306 -> [_]
              i -> [w1435]
              n746 = local read "Transport Line Color"() -> (w1434:u32)
              n747 = local read "Ring"() -> (w1433:u16)
              n748 = property on="Transport" class="XYGraph (strict)"("Active Plot"=w1435, "Plot.Plot Color"=w1434, "Plot.Line Width"=w1433) -> ()  [unwired: 2 in, 2 out]
            }
            n749 = call <vilib>:"Check if File or Folder Exists.vi"("error in (no error)"=w1390, "path"=w1391) -> ("file or folder exists?"=w1388:bool, "dup path"=w1389:path)  [unwired: 7 in, 1 out]
            n750 = case shown="True" w1388 {
              tunnel: w1389 -> [_ w1441]
              frame False {
              }
              frame True {
                n751 = Read from Text File(file (use dialog)=w1441) -> (text=w1445:string)  [unwired: 3 in, 3 out]
                n752 = property on="Image Out" class="ImageControl"() -> ("ROI"=w1442:T12)  [unwired: 2 in, 2 out]
                n753 = Unflatten From String(type=w1442, binary string=w1445) -> (value=w1443:T12, error out=w1444:errorcluster)  [unwired: 3 in, 1 out]
                n754 = property on="Image Out" class="ImageControl"(error in=w1444, "ROI"=w1443) -> ()  [unwired: 1 in, 2 out]
              }
            }
            n755 = invoke on="Image Out" class="ImageControl" method="Clear ROI"() -> ()  [unwired: 3 in, 3 out]
            n756 = call-poly <vilib>:"Read From Spreadsheet File.vi"("file path (dialog if empty)"=w1251) -> ("all rows"=w1255:string[][])  [unwired: 6 in, 4 out]
            n757 = Array Size(array=w1255) -> (size(s)=w1274:i32[])
            n758 = Index Array(array=w1274, index=0) -> (element=w1272:i32)
            n759 = Path To String(path=w1383) -> (string=w1415:string)
            n760 = Index Array(array=w1417, index=w1416) -> (element=w1395:string)
            n761 = Concatenate Strings(w1415, "\\", w1395) -> (w1414:string)
            n762 = Array Subset(array=w1255, index (row)=w1273, index (col)=w1273, length (col)=3) -> (w1275:string[][])  [unwired: 1 in]
            n763 = local write "Image Name"(w1395) -> ()
            n764 = String To Path(string=w1414) -> (path=w1394:path)
            n765 = Empty String/Path?(string/path=w1395) -> (empty?=w1396:bool)
            n766 = local read "No Image File"() -> (w1392:path)
            n767 = Reshape Array(w1275, w1272) -> (w1257:string[])
            n768 = Search 1D Array(1D array=w1257, element="Vg") -> (index of element=w1261:i32)  [unwired: 1 in]
            n769 = Add(x=w1261, y=3) -> (x+y=w1259:i32)
            n770 = Divide(x=w1259, y=3) -> (x/y=w1266:dbl)
            n771 = Array Subset(array=w1255, index (row)=w1266, index (col)=0, length (col)=1) -> (w1265:string[][])  [unwired: 1 in]
            n772 = Fract/Exp String To Number(string=w1265) -> (number=w1269:dbl[][])  [unwired: 3 in, 1 out]
            n773 = Array Size(array=w1269) -> (size(s)=w1256:i32[])
            n774 = Index Array(array=w1256, index=0) -> (element=w1267:i32)
            n775 = Decrement(x=w1267) -> (x-1=w1270:i32)
            n776 = Reshape Array(w1269, w1270) -> (w1254:dbl[])
            n777 = local write "Data Length"(w1270) -> ()
            n778 = local write "Vg Column"(w1254) -> ()
            n779 = Select(t=w1392, s=w1396, f=w1394) -> (s? t:f=w1393:path)
            n780 = local write "Image File"(w1393) -> ()
            n781 = Array Max & Min(array=w1254) -> (max value=w1253:dbl, min value=w1252:dbl)  [unwired: 2 out]
            n782 = property on="Sat-Trans Slider" class="Slide (strict)"("Scale.Maximum"=w1253, "Scale.Minimum"=w1252) -> ()  [unwired: 2 in, 2 out]
            n783 = call "Vision Acquisition3"("Image Path"=w1393) -> ("Image Out"=w1418:T2)  [unwired: 25 in, 1 out]
            n784 = local write "Image Out"(w1418) -> ()
            n785 = local write "Image Out 2"(w1418) -> ()
          }
          event "Up Button": Mouse Down {
            w1588 = 0
            w1604 = "\\"
            w1605 = "TSP"
            w1746 = 0
            # "Transpose"
            n786 = event-data() -> ()  [unwired: 1 in, 5 out]
            n787 = local read "Transfer File"() -> (w1742:path)
            n788 = Strip Path(path=w1742) -> (stripped path=w1596:path, name=w1756:string)
            n789 = local write "Transfer Folder"(w1596) -> ()
            n790 = List Folder(path=w1596) -> (filenames=w1751:string[], error out=w1709:errorcluster)  [unwired: 3 in, 2 out]
            n791 = Array Size(array=w1751) -> (size(s)=w1697:i32)
            n792 = Search 1D Array(1D array=w1751, element=w1756) -> (index of element=w1752:i32)  [unwired: 1 in]
            n793 = Equal To 0?(x=w1752) -> (x = 0?=w1753:bool)
            n794 = local read "Folder Index"() -> (w1696:dbl)
            n795 = property on="Image Out" class="ImageControl"() -> (error out=w1699:errorcluster, "Image Center Position"=w1703:cluster{"X":u32, "Y":u32})  [unwired: 2 in, 1 out]
            n796 = Strip Path(path=w1596) -> (stripped path=w1600:path)  [unwired: 1 out]
            n797 = Path To String(path=w1600) -> (string=w1603:string)
            n798 = case shown="True" w1753 {
              tunnel: w1696 -> [w1897 _]
              tunnel: [w1896 w1898] -> w1695
              tunnel: w1697 -> [_ w1899]
              frame False {
                n799 = Decrement(x=w1897) -> (x-1=w1896:dbl)
              }
              frame True {
                n800 = Decrement(x=w1899) -> (x-1=w1898:i32)
              }
            }
            n801 = Unbundle(w1703) -> ("X"=w1701:u32)  [unwired: 1 out]
            n802 = local write "Folder Index"(w1695) -> ()
            n803 = local read "Folder Index"() -> (w1628:dbl)
            n804 = Bundle("X"=w1701, 0) -> (w1702:cluster{"X":u32, i32})  [unwired: 1 in]
            n805 = Path To String(path=w1596) -> (string=w1757:string)
            n806 = Index Array(array=w1751, index=w1695) -> (element=w1597:string)
            n807 = String Subset(string=w1597, offset (0)=3) -> (substring=w1599:string)  [unwired: 1 in]
            n808 = Concatenate Strings(w1605, w1599) -> (w1601:string)
            n809 = Concatenate Strings(w1603, w1604, w1605, w1604, w1601) -> (w1602:string)
            n810 = String To Path(string=w1602) -> (path=w1595:path)
            n811 = local write "Transport File"(w1595) -> ()
            n812 = Strip Path(path=w1595) -> (stripped path=w1629:path, name=w1634:string)
            n813 = local write "Transport Folder"(w1629) -> ()
            n814 = List Folder(path=w1629) -> (filenames=w1630:string[], error out=w1626:errorcluster)  [unwired: 3 in, 2 out]
            n815 = Array Size(array=w1630) -> (size(s)=w1592:i32)
            n816 = Search 1D Array(1D array=w1630, element=w1634) -> (index of element=w1594:i32)  [unwired: 1 in]
            n817 = local write "Data Name:"(w1597) -> ()
            n818 = property on="Image Out" class="ImageControl"(error in=w1699, "Image Center Position"=w1702) -> ()  [unwired: 1 in, 2 out]
            n819 = Equal To 0?(x=w1594) -> (x = 0?=w1593:bool)
            n820 = case shown="False" w1593 {
              tunnel: w1628 -> [w1760 _]
              tunnel: [w1759 w1761] -> w1627
              tunnel: w1626 -> [w1758 w1762]
              tunnel: [w1758 w1762] -> _
              tunnel: w1592 -> [_ w1761]
              frame False {
                n821 = Decrement(x=w1760) -> (x-1=w1759:dbl)
              }
              frame True {
              }
            }
            n822 = local write "Folder Index"(w1627) -> ()
            n823 = Concatenate Strings(w1757, "\\", w1597) -> (w1755:string)
            n824 = Path To String(path=w1629) -> (string=w1635:string)
            n825 = Index Array(array=w1630, index=w1627) -> (element=w1631:string)
            n826 = String To Path(string=w1755) -> (path=w1566:path)
            n827 = call "Recorded Values.vi"("Path"=w1566) -> ("Recorded Char"=w1693:T6, "Recorded Prop"=w1692:T7, "Fabrication Prop"=w1694:T8)  [unwired: 8 in]
            n828 = Unbundle By Name(w1693) -> ("Mobility-Sat"=w1680:dbl, "Moblitity-Lin"=w1679:dbl, "On/Off"=w1678:dbl, "Off Current"=w1677:dbl, "Vt-Sat"=w1644:dbl, "STS"=w1676:dbl, "Trap Density-VT"=w1675:dbl, "Trap Density-STS"=w1674:dbl)
            n829 = Unbundle By Name(w1694) -> ("Date Created"=w1673:string, "Material"=w1691:string, "Solvent"=w1690:string, "Concentration"=w1689:dbl, "Method"=w1688:string, "Dielectric (nm)"=w1687:dbl, "Treatment"=w1686:string, "Comments"=w1685:string)
            n830 = Unbundle By Name(w1692) -> ("Date Recorded"=w1684:string, "Index"=w1683:string, "Length"=w1682:dbl, "Width"=w1681:dbl, "Sample Temp"=w1645:dbl)
            n831 = local write "Date Created"(w1673) -> ()
            n832 = local write "Rec: Material"(w1691) -> ()
            n833 = local write "Rec: Off I-Sat"(w1677) -> ()
            n834 = local write "Rec: Comments"(w1685) -> ()
            n835 = local write "Rec: VT-Sat"(w1644) -> ()
            n836 = local write "Rec: Solvent"(w1690) -> ()
            n837 = local write "Rec: Concentration"(w1689) -> ()
            n838 = local write "Rec: Method"(w1688) -> ()
            n839 = local write "Rec: Dielectric (d)"(w1687) -> ()
            n840 = local write "Surface Treatment:"(w1686) -> ()
            n841 = local write "Index"(w1683) -> ()
            n842 = local write "Rec: Mobility-Sat"(w1680) -> ()
            n843 = local write "Rec: Mobility-Lin"(w1679) -> ()
            n844 = local write "Rec: On/Off"(w1678) -> ()
            n845 = local write "Rec: STS"(w1676) -> ()
            n846 = local write "Rec: Trap Density-VT"(w1675) -> ()
            n847 = local write "Rec: Trap Density-STS"(w1674) -> ()
            n848 = local write "Date Recorded"(w1684) -> ()
            n849 = local write "Rec: Length"(w1682) -> ()
            n850 = local write "Rec: Width"(w1681) -> ()
            n851 = local write "Rec: Temp"(w1645) -> ()
            n852 = Equal To 0?(x=w1645) -> (x = 0?=w1647:bool)
            n853 = case shown="False" w1647 {
              tunnel: [w1769 w1770] -> w1646
              tunnel: w1645 -> [w1769 _]
              frame False {
              }
              frame True {
                n854 = local read "Room Temp"() -> (w1770:dbl)
              }
            }
            n855 = local write "Data Name:"(w1631) -> ()
            n856 = local read "NumPoints Log"() -> (w1669:dbl)
            n857 = local write "Transfer File"(w1566) -> ()
            n858 = local read "Num Pts"() -> (w1672:dbl)
            n859 = Concatenate Strings(w1635, "\\", w1631) -> (w1633:string)
            n860 = local read "New: Dielectric"() -> (w1653:dbl)
            n861 = call "Mobility-Vt Calculator-File.vi"("NumPts"=w1672, "Path"=w1566) -> ("Graph Cluster"=w1642:T9, "Output"=w1671:T10, "Index-Sat"=w1670:dbl, "Index-Lin"=w1657:dbl)  [unwired: 5 in, 1 out]
            n862 = call "STS Calculator-File.vi"("NumPts"=w1669, "Path"=w1566) -> ("STS Index-Sat"=w1668:dbl, "XY Graph-Sat"=w1667:cluster{dbl[], dbl[]}[], "Ouput"=w1666:cluster{"STS-Sat":dbl, "STS-Lin":dbl})  [unwired: 5 in, 2 out]
            n863 = call-poly <vilib>:"Read From Spreadsheet File.vi"("file path (dialog if empty)"=w1566) -> ("all rows"=w1748:string[][])  [unwired: 6 in, 4 out]
            n864 = String To Path(string=w1633) -> (path=w1636:path)
            n865 = Unbundle By Name(w1671) -> ("Mobility-Sat"=w1656:dbl, "Vt-Sat"=w1649:dbl, "Mobility-Lin"=w1655:dbl, "Vt-Lin"=w1654:dbl, "Off I-Sat"=w1648:dbl, "On/Off I-Sat"=w1643:dbl)
            n866 = Strip Path(path=w1636) -> ()  [unwired: 2 out]
            n867 = call-poly <vilib>:"Read From Spreadsheet File.vi"("file path (dialog if empty)"=w1636) -> ("all rows"=w1612:string[][])  [unwired: 6 in, 4 out]
            n868 = local write "Sat-Trans Slider"(w1670) -> ()
            n869 = Unbundle By Name(w1666) -> ("STS-Sat"=w1650:dbl)  [unwired: 1 out]
            n870 = local write "Index 2"(w1668) -> ()
            n871 = local write "MobVi Index"(w1670) -> ()
            n872 = local write "Sat-Log"(w1667) -> ()
            n873 = Array Size(array=w1612) -> (size(s)=w1606:i32[])
            n874 = local write "Calc: Mobility-Sat"(w1656) -> ()
            n875 = local write "Calc: VT-Sat"(w1649) -> ()
            n876 = local write "Calc: Mobility-Lin"(w1655) -> ()
            n877 = local write "Calc: Off I-Sat"(w1648) -> ()
            n878 = local write "Calc: On/Off"(w1643) -> ()
            n879 = Array Size(array=w1748) -> (size(s)=w1747:i32[])
            n880 = local write "Calc: VT-Lin"(w1654) -> ()
            n881 = call "Trap Density_VT.vi"("VT"=w1649, "Dielectric"=w1653) -> ("Trap Density-VT"=w1652:dbl)
            n882 = call "Trap Density_STS.vi"("Temp (T) [K]"=w1646, "S.T.S. (S)"=w1650, "Dielectric"=w1653) -> ("Trap Density (N)"=w1651:dbl)  [unwired: 8 in]
            n883 = Unbundle By Name(w1642) -> ("Raw Sat"=w1639:cluster{dbl[], dbl[]}[], "Sqrt Sat"=w1640:cluster{dbl[], dbl[]}[], "Raw Lin"=w1638:cluster{dbl[], dbl[]}[], "Sqrt Lin"=w1641:cluster{dbl[], dbl[]}[], "Log Lin"=w1637:cluster{dbl[], dbl[]}[])  [unwired: 1 out]
            n884 = local write "Sqrt-Sat"(w1640) -> ()
            n885 = local write "Calc: STS"(w1650) -> ()
            n886 = local write "New: STS"(w1650) -> ()
            n887 = Array Subset(array=w1612, length (col)=1) -> (w1610:string[][])  [unwired: 3 in]
            n888 = Index Array(array=w1606, index=0) -> (element=w1617:i32)
            n889 = Decimate 1D Array(w1641) -> (w1665:cluster{dbl[], dbl[]}[])  [unwired: 1 out]
            n890 = local write "Calc: Trap Density-VT"(w1652) -> ()
            n891 = local write "New: VT-Sat"(w1649) -> ()
            n892 = local write "Calc: Trap Density-STS"(w1651) -> ()
            n893 = local write "New: Trap Density-STS"(w1651) -> ()
            n894 = local write "New: Trap Density-VT"(w1652) -> ()
            n895 = Reshape Array(w1610, w1617) -> (w1611:string[])
            n896 = local write "New: VT-Lin"(w1654) -> ()
            n897 = local write "Sqrt-Lin"(w1641) -> ()
            n898 = local write "New: Mobility-Sat"(w1656) -> ()
            n899 = local write "New: Mobility-Lin"(w1655) -> ()
            n900 = Decimate 1D Array(w1667) -> (w1726:cluster{dbl[], dbl[]}[])  [unwired: 1 out]
            n901 = Index Array(array=w1747, index=w1746) -> (element=w1732:i32)
            n902 = Decimate 1D Array(w1640) -> (w1736:cluster{dbl[], dbl[]}[])  [unwired: 1 out]
            n903 = Array To Cluster(array=w1665) -> (cluster=w1664:T11)
            n904 = Array Subset(array=w1748, index (row)=w1746, index (col)=w1746, length (col)=3) -> (w1749:string[][])  [unwired: 1 in]
            n905 = Search 1D Array(1D array=w1611, element="Vd") -> (index of element=w1613:i32)  [unwired: 1 in]
            n906 = local write "Raw- Sat"(w1639) -> ()
            n907 = local write "Raw- Lin"(w1638) -> ()
            n908 = local write "Log-Lin"(w1637) -> ()
            n909 = Array To Cluster(array=w1726) -> (cluster=w1724:T11)
            n910 = Array To Cluster(array=w1736) -> (cluster=w1738:T11)
            n911 = Reshape Array(w1749, w1732) -> (w1739:string[])
            n912 = Increment(x=w1613) -> (x+1=w1614:i32)
            n913 = Array Subset(array=w1612, index (row)=w1614) -> (w1616:string[][])  [unwired: 3 in]
            n914 = Subtract(x=w1732, y=20) -> (x-y=w1731:i32)
            n915 = Unbundle(w1664) -> ("[0]"=w1661:cluster{dbl[], dbl[]})  [unwired: 8 out]
            n916 = Fract/Exp String To Number(string=w1616, default (0 dbl)="default (0 dbl) 6") -> (number=w1624:ext[][])  [unwired: 2 in, 1 out]
            n917 = Delete From Array(array=w1624) -> (array with subset deleted=w1625:ext[][])  [unwired: 3 in, 1 out]
            n918 = property on="Sat-Trans Slider" class="Slide (strict)"("Scale.Maximum"=w1731) -> ()  [unwired: 2 in, 2 out]
            n919 = Delete From Array(array=w1625, index (col)=0 ("Deaktivierter Index (Spalte)")) -> (deleted portion=w1620:ext[], array with subset deleted=w1619:ext[][])  [unwired: 2 in]
            n920 = local read "Num Pts"() -> (w1658:dbl)
            n921 = Unbundle(w1724) -> ("[0]"=w1725:cluster{dbl[], dbl[]})  [unwired: 8 out]
            n922 = Unbundle(w1738) -> ("[0]"=w1737:cluster{dbl[], dbl[]})  [unwired: 8 out]
            n923 = Unbundle(w1661) -> (w1660:dbl[], w1659:dbl[])
            n924 = Search 1D Array(1D array=w1739, element="Index:") -> (index of element=w1743:i32)  [unwired: 1 in]
            n925 = Transpose 2D Array(2D array=w1619) -> (transposed array=w1618:ext[][])
            n926 = Increment(x=w1743) -> (x+1=w1744:i32)
            n927 = Unbundle(w1725) -> (w1723:dbl[], w1722:dbl[])
            n928 = Unbundle(w1737) -> (w1730:dbl[], w1729:dbl[])
            n929 = for {
              tunnel: w1620 -> [w1767]
              tunnel: w1618 -> [w1768] mode=indexing
              tunnel: [w1766] -> w1622 mode=indexing
              n930 = Bundle(w1767, w1768) -> (w1766:cluster{ext[], ext[]})  [unwired: 1 in]
            }
            n931 = Array Subset(array=w1660, index=w1657, length=w1658) -> (w1662:dbl[])
            n932 = Array Subset(array=w1659, index=w1657, length=w1658) -> (w1663:dbl[])
            n933 = local read "Image Folder"() -> (w1698:path)
            n934 = local write "Lin-Vg Array-Used"(w1662) -> ()
            n935 = Array Subset(array=w1723, index=w1668, length=w1669) -> (w1728:dbl[])
            n936 = Array Subset(array=w1722, index=w1668, length=w1669) -> (w1727:dbl[])
            n937 = Array Subset(array=w1730, index=w1670, length=w1672) -> (w1735:dbl[])
            n938 = Array Subset(array=w1729, index=w1670, length=w1672) -> (w1734:dbl[])
            n939 = local write "Lin Id-Used"(w1663) -> ()
            n940 = local write "Transport"(w1622) -> ()
            n941 = Index Array(array=w1739, index=w1744) -> (element=w1705:string)
            n942 = Array Size(array=w1622) -> (size(s)=w1623:i32)
            n943 = for {
              N: w1623 -> [_]
              i -> [w1765]
              n944 = local read "Transport Line Color"() -> (w1764:u32)
              n945 = local read "Ring"() -> (w1763:u16)
              n946 = property on="Transport" class="XYGraph (strict)"("Active Plot"=w1765, "Plot.Plot Color"=w1764, "Plot.Line Width"=w1763) -> ()  [unwired: 2 in, 2 out]
            }
            n947 = local write "Sat Vg Array-Used"(w1735) -> ()
            n948 = local write "Vg Array-Log-Used"(w1727) -> ()
            n949 = local write "Sat Id-Log-Used"(w1728) -> ()
            n950 = local write "Sat Id-Used"(w1734) -> ()
            n951 = local write "Index"(w1705) -> ()
            n952 = List Folder(path=w1698, error in=w1709) -> (filenames=w1741:string[], error out=w1708:errorcluster)  [unwired: 2 in, 2 out]
            n953 = Build Path(base path=w1698, name or relative path="ROI") -> (appended path=w1706:path)
            n954 = invoke on="Image Out" class="ImageControl" method="Clear ROI"(error in=w1708) -> (error out=w1712:errorcluster)  [unwired: 2 in, 2 out]
            n955 = while {
              tunnel: w1741 -> [w1783]
              tunnel: w1705 -> [w1781]
              tunnel: [w1780] -> w1740
              tunnel: w1732 -> [w1779]
              i -> [w1780]
              stop <- w1776 stop-if-true
              n956 = Index Array(array=w1783, index=w1780) -> (element=w1784:string)
              n957 = xnode "Match Regular Expression"("input string"=w1784, "regular expression"=w1781) -> ("whole match"=w1782:string)  [unwired: 4 in, 4 out]
              n958 = Equal?(x=w1782, y=w1781) -> (x = y?=w1778:bool)
              n959 = Equal?(x=w1779, y=w1780) -> (x = y?=w1777:bool)
              n960 = Or(x=w1778, y=w1777) -> (x .or. y?=w1776:bool)
            }
            n961 = Build Path(base path=w1706, name or relative path=w1705) -> (appended path=w1704:path)
            n962 = call <vilib>:"Check if File or Folder Exists.vi"("error in (no error)"=w1712, "path"=w1704) -> ("file or folder exists?"=w1710:bool, "dup path"=w1711:path)  [unwired: 7 in, 1 out]
            n963 = case shown="True" w1710 {
              tunnel: w1711 -> [_ w1771]
              frame False {
              }
              frame True {
                n964 = Read from Text File(file (use dialog)=w1771) -> (text=w1775:string)  [unwired: 3 in, 3 out]
                n965 = property on="Image Out" class="ImageControl"() -> ("ROI"=w1772:T12)  [unwired: 2 in, 2 out]
                n966 = Unflatten From String(type=w1772, binary string=w1775) -> (value=w1773:T12, error out=w1774:errorcluster)  [unwired: 3 in, 1 out]
                n967 = property on="Image Out" class="ImageControl"(error in=w1774, "ROI"=w1773) -> ()  [unwired: 1 in, 2 out]
              }
            }
            n968 = call-poly <vilib>:"Read From Spreadsheet File.vi"("file path (dialog if empty)"=w1566) -> ("all rows"=w1570:string[][])  [unwired: 6 in, 4 out]
            n969 = Array Size(array=w1570) -> (size(s)=w1589:i32[])
            n970 = Index Array(array=w1589, index=0) -> (element=w1587:i32)
            n971 = Index Array(array=w1741, index=w1740) -> (element=w1714:string)
            n972 = local write "Image Name"(w1714) -> ()
            n973 = Array Subset(array=w1570, index (row)=w1588, index (col)=w1588, length (col)=3) -> (w1590:string[][])  [unwired: 1 in]
            n974 = Empty String/Path?(string/path=w1714) -> (empty?=w1721:bool)
            n975 = Build Path(base path=w1698, name or relative path=w1714) -> (appended path=w1713:path)
            n976 = local read "No Image File"() -> (w1720:path)
            n977 = Reshape Array(w1590, w1587) -> (w1572:string[])
            n978 = Search 1D Array(1D array=w1572, element="Vg") -> (index of element=w1576:i32)  [unwired: 1 in]
            n979 = Add(x=w1576, y=3) -> (x+y=w1574:i32)
            n980 = Divide(x=w1574, y=3) -> (x/y=w1581:dbl)
            n981 = Array Subset(array=w1570, index (row)=w1581, index (col)=0, length (col)=1) -> (w1580:string[][])  [unwired: 1 in]
            n982 = Fract/Exp String To Number(string=w1580) -> (number=w1584:dbl[][])  [unwired: 3 in, 1 out]
            n983 = Array Size(array=w1584) -> (size(s)=w1571:i32[])
            n984 = Index Array(array=w1571, index=0) -> (element=w1582:i32)
            n985 = Decrement(x=w1582) -> (x-1=w1585:i32)
            n986 = Reshape Array(w1584, w1585) -> (w1569:dbl[])
            n987 = local write "Data Length"(w1585) -> ()
            n988 = local write "Vg Column"(w1569) -> ()
            n989 = Array Max & Min(array=w1569) -> (max value=w1568:dbl, min value=w1567:dbl)  [unwired: 2 out]
            n990 = Select(t=w1720, s=w1721, f=w1713) -> (s? t:f=w1715:path)
            n991 = call <vilib>:"Get File Extension.vi"("file"=w1715) -> ("lowercase file extension"=w1717:string)  [unwired: 7 in, 3 out]
            n992 = local write "Image File"(w1715) -> ()
            n993 = local write "String"(w1717) -> ()
            n994 = property on="Sat-Trans Slider" class="Slide (strict)"("Scale.Maximum"=w1568, "Scale.Minimum"=w1567) -> ()  [unwired: 2 in, 2 out]
            n995 = Search 1D Array(1D array=string[] ["bmp", "jpeg", "png", "jpg", "gif"], element=w1717) -> (index of element=w1716:i32)  [unwired: 1 in]
            n996 = call "Vision Acquisition5"("Image Path"=w1715) -> ("Image Out"=w1719:T2)  [unwired: 25 in, 1 out]
            n997 = Less Than 0?(x=w1716) -> ()  [unwired: 1 out]
            n998 = local write "Image Out"(w1719) -> ()
            n999 = local write "Image Out 2"(w1719) -> ()
          }
          event "Save Changes? 3": Mouse Down {
            n1000 = event-data() -> ()  [unwired: 1 in, 7 out]
            n1001 = local read "Image Folder"() -> (w1900:path)
            n1002 = Build Path(base path=w1900, name or relative path="ROI") -> (appended path=w1907:path)
            n1003 = call <vilib>:"Check if File or Folder Exists.vi"("path"=w1907) -> ("file or folder exists?"=w1909:bool, "dup path"=w1906:path)  [unwired: 8 in, 1 out]
            n1004 = case shown="False" w1909 {
              tunnel: w1906 -> [w1911 w1912]
              tunnel: [w1910 w1912] -> w1901
              frame False {
                n1005 = Create Folder(path (use dialog)=w1911) -> (created path=w1910:path)  [unwired: 2 in, 2 out]
              }
              frame True {
              }
            }
            n1006 = local read "Index"() -> (w1903:string)
            n1007 = property on="Image Out" class="ImageControl"() -> ("ROI"=w1905:T12)  [unwired: 2 in, 2 out]
            n1008 = Build Path(base path=w1901, name or relative path=w1903) -> (appended path=w1902:path)
            n1009 = Flatten To String(anything=w1905) -> (data string=w1904:string)  [unwired: 3 in, 2 out]
            n1010 = Write to Text File(file (use dialog)=w1902, text=w1904) -> ()  [unwired: 2 in, 3 out]
          }
          event "Next Sqrt Sat": Mouse Down {
            n1011 = event-data() -> ()  [unwired: 1 in, 5 out]
            n1012 = local read "Sqrt-Sat"() -> (w1925:cluster{dbl[], dbl[]}[])
            n1013 = Decimate 1D Array(w1925) -> (w1921:cluster{dbl[], dbl[]}[], w1920:cluster{dbl[], dbl[]}[])
            n1014 = Array To Cluster(array=w1921) -> (cluster=w1931:T11)
            n1015 = Unbundle(w1931) -> ("[0]"=w1930:cluster{dbl[], dbl[]})  [unwired: 8 out]
            n1016 = local read "MobVi Index"() -> (w1927:dbl)
            n1017 = local read "Num Pts"() -> (w1926:dbl)
            n1018 = Unbundle(w1930) -> (w1929:dbl[], w1928:dbl[])
            n1019 = Increment(x=w1927) -> (x+1=w1922:dbl)
            n1020 = local read "New: Dielectric"() -> (w1916:dbl)
            n1021 = local read "New: Length"() -> (w1915:dbl)
            n1022 = local read "New: Width"() -> (w1914:dbl)
            n1023 = local write "MobVi Index"(w1922) -> ()
            n1024 = Array Subset(array=w1929, index=w1922, length=w1926) -> (w1918:dbl[])
            n1025 = Array Subset(array=w1928, index=w1922, length=w1926) -> (w1917:dbl[])
            n1026 = local write "Sat Vg Array-Used"(w1918) -> ()
            n1027 = local write "Sat Id-Used"(w1917) -> ()
            n1028 = call "Mobility-Vt-Used Pts_Saturation.vi"("Width"=w1914, "Length"=w1915, "Dielectric (d)"=w1916, "Sat Id Used"=w1917, "Vg Used"=w1918) -> ("Vt"=w1913:dbl, "Mobility"=w1919:dbl)  [unwired: 4 in, 1 out]
            n1029 = Bundle(w1918, w1917) -> (w1924:cluster{dbl[], dbl[]})  [unwired: 1 in]
            n1030 = Build Array (concatenate)(w1921, w1920, w1924) -> (w1923:cluster{dbl[], dbl[]}[])
            n1031 = local write "New: Mobility-Sat"(w1919) -> ()
            n1032 = local write "New: VT-Sat"(w1913) -> ()
            n1033 = local write "Sqrt-Sat"(w1923) -> ()
          }
          event "Next Log Sat": Mouse Down {
            n1034 = event-data() -> ()  [unwired: 1 in, 7 out]
            n1035 = local read "Sat-Log"() -> (w1940:cluster{dbl[], dbl[]}[])
            n1036 = Decimate 1D Array(w1940) -> (w1936:cluster{dbl[], dbl[]}[], w1935:cluster{dbl[], dbl[]}[])
            n1037 = Array To Cluster(array=w1936) -> (cluster=w1946:T11)
            n1038 = local read "Index 2"() -> (w1942:dbl)
            n1039 = local read "NumPoints Log"() -> (w1941:dbl)
            n1040 = Unbundle(w1946) -> ("[0]"=w1945:cluster{dbl[], dbl[]})  [unwired: 8 out]
            n1041 = Unbundle(w1945) -> (w1944:dbl[], w1943:dbl[])
            n1042 = Increment(x=w1942) -> (x+1=w1937:dbl)
            n1043 = local write "Index 2"(w1937) -> ()
            n1044 = Array Subset(array=w1943, index=w1937, length=w1941) -> (w1932:dbl[])
            n1045 = Array Subset(array=w1944, index=w1937, length=w1941) -> (w1933:dbl[])
            n1046 = call "STS-Used.vi"("Id Used"=w1933, "Vg-Used"=w1932) -> ("STS"=w1934:dbl)  [unwired: 9 in]
            n1047 = Bundle(w1933, w1932) -> (w1939:cluster{dbl[], dbl[]})  [unwired: 1 in]
            n1048 = local write "Vg Array-Log-Used"(w1932) -> ()
            n1049 = local write "Sat Id-Log-Used"(w1933) -> ()
            n1050 = local write "New: STS"(w1934) -> ()
            n1051 = Build Array (concatenate)(w1936, w1935, w1939) -> (w1938:cluster{dbl[], dbl[]}[])
            n1052 = local write "Sat-Log"(w1938) -> ()
          }
          event "Previous Log Sat": Mouse Down {
            n1053 = event-data() -> ()  [unwired: 1 in, 7 out]
            n1054 = local read "Sat-Log"() -> (w1956:cluster{dbl[], dbl[]}[])
            n1055 = Decimate 1D Array(w1956) -> (w1953:cluster{dbl[], dbl[]}[], w1952:cluster{dbl[], dbl[]}[])
            n1056 = Array To Cluster(array=w1953) -> (cluster=w1961:T11)
            n1057 = local read "Index 2"() -> (w1949:dbl)
            n1058 = local read "NumPoints Log"() -> (w1957:dbl)
            n1059 = Unbundle(w1961) -> ("[0]"=w1960:cluster{dbl[], dbl[]})  [unwired: 8 out]
            n1060 = Unbundle(w1960) -> (w1959:dbl[], w1958:dbl[])
            n1061 = Decrement(x=w1949) -> (x-1=w1950:dbl)
            n1062 = local write "Index 2"(w1950) -> ()
            n1063 = Array Subset(array=w1959, index=w1950, length=w1957) -> (w1947:dbl[])
            n1064 = Array Subset(array=w1958, index=w1950, length=w1957) -> (w1948:dbl[])
            n1065 = local write "Sat Id-Log-Used"(w1947) -> ()
            n1066 = Bundle(w1947, w1948) -> (w1955:cluster{dbl[], dbl[]})  [unwired: 1 in]
            n1067 = call "STS-Used.vi"("Id Used"=w1947, "Vg-Used"=w1948) -> ("STS"=w1951:dbl)  [unwired: 9 in]
            n1068 = local write "Vg Array-Log-Used"(w1948) -> ()
            n1069 = Build Array (concatenate)(w1953, w1952, w1955) -> (w1954:cluster{dbl[], dbl[]}[])
            n1070 = local write "New: STS"(w1951) -> ()
            n1071 = local write "Sat-Log"(w1954) -> ()
          }
          event "Previous Sqrt Sat": Mouse Down {
            n1072 = event-data() -> ()  [unwired: 1 in, 5 out]
            n1073 = local read "Sqrt-Sat"() -> (w1975:cluster{dbl[], dbl[]}[])
            n1074 = Decimate 1D Array(w1975) -> (w1972:cluster{dbl[], dbl[]}[], w1971:cluster{dbl[], dbl[]}[])
            n1075 = Array To Cluster(array=w1972) -> (cluster=w1980:T11)
            n1076 = local read "MobVi Index"() -> (w1970:dbl)
            n1077 = Unbundle(w1980) -> ("[0]"=w1979:cluster{dbl[], dbl[]})  [unwired: 8 out]
            n1078 = local read "Num Pts"() -> (w1976:dbl)
            n1079 = Unbundle(w1979) -> (w1978:dbl[], w1977:dbl[])
            n1080 = Decrement(x=w1970) -> (x-1=w1969:dbl)
            n1081 = local read "New: Dielectric"() -> (w1963:dbl)
            n1082 = local read "New: Length"() -> (w1964:dbl)
            n1083 = local read "New: Width"() -> (w1965:dbl)
            n1084 = local write "MobVi Index"(w1969) -> ()
            n1085 = Array Subset(array=w1978, index=w1969, length=w1976) -> (w1968:dbl[])
            n1086 = Array Subset(array=w1977, index=w1969, length=w1976) -> (w1967:dbl[])
            n1087 = local write "Sat Vg Array-Used"(w1968) -> ()
            n1088 = local write "Sat Id-Used"(w1967) -> ()
            n1089 = call "Mobility-Vt-Used Pts_Linear.vi"("Width"=w1965, "Length"=w1964, "Dielectric (d)"=w1963, "Sat Id Used"=w1967, "Vg Used"=w1968) -> ("Vt"=w1962:dbl, "Mobility"=w1966:dbl)  [unwired: 4 in, 1 out]
            n1090 = Bundle(w1968, w1967) -> (w1974:cluster{dbl[], dbl[]})  [unwired: 1 in]
            n1091 = local write "New: VT-Sat"(w1962) -> ()
            n1092 = Build Array (concatenate)(w1972, w1971, w1974) -> (w1973:cluster{dbl[], dbl[]}[])
            n1093 = local write "New: Mobility-Sat"(w1966) -> ()
            n1094 = local write "Sqrt-Sat"(w1973) -> ()
          }
          event "Sat-Trans Slider": Value Change {
            n1095 = event-data() -> ()  [unwired: 1 in, 5 out]
            n1096 = local read "Sqrt-Sat"() -> (w1993:cluster{dbl[], dbl[]}[])
            n1097 = Decimate 1D Array(w1993) -> (w1990:cluster{dbl[], dbl[]}[], w1989:cluster{dbl[], dbl[]}[])
            n1098 = Array To Cluster(array=w1990) -> (cluster=w1998:T11)
            n1099 = Unbundle(w1998) -> ("[0]"=w1997:cluster{dbl[], dbl[]})  [unwired: 8 out]
            n1100 = local read "Sat-Trans Slider"() -> (w1982:dbl)
            n1101 = local read "Num Pts"() -> (w1994:dbl)
            n1102 = Unbundle(w1997) -> (w1996:dbl[], w1995:dbl[])
            n1103 = local read "New: Dielectric"() -> (w1983:dbl)
            n1104 = local read "New: Length"() -> (w1984:dbl)
            n1105 = local read "New: Width"() -> (w1985:dbl)
            n1106 = local write "MobVi Index"(w1982) -> ()
            n1107 = Array Subset(array=w1996, index=w1982, length=w1994) -> (w1988:dbl[])
            n1108 = Array Subset(array=w1995, index=w1982, length=w1994) -> (w1987:dbl[])
            n1109 = local write "Sat Vg Array-Used"(w1988) -> ()
            n1110 = local write "Sat Id-Used"(w1987) -> ()
            n1111 = call "Mobility-Vt-Used Pts_Linear.vi"("Width"=w1985, "Length"=w1984, "Dielectric (d)"=w1983, "Sat Id Used"=w1987, "Vg Used"=w1988) -> ("Vt"=w1981:dbl, "Mobility"=w1986:dbl)  [unwired: 4 in, 1 out]
            n1112 = Bundle(w1988, w1987) -> (w1992:cluster{dbl[], dbl[]})  [unwired: 1 in]
            n1113 = local write "New: VT-Sat"(w1981) -> ()
            n1114 = Build Array (concatenate)(w1990, w1989, w1992) -> (w1991:cluster{dbl[], dbl[]}[])
            n1115 = local write "New: Mobility-Sat"(w1986) -> ()
            n1116 = local write "Sqrt-Sat"(w1991) -> ()
          }
          event "Sat-Log Slider": Value Change {
            n1117 = event-data() -> ()  [unwired: 1 in, 5 out]
            n1118 = local read "Sat-Log"() -> (w2007:cluster{dbl[], dbl[]}[])
            n1119 = Decimate 1D Array(w2007) -> (w2004:cluster{dbl[], dbl[]}[], w2003:cluster{dbl[], dbl[]}[])
            n1120 = Array To Cluster(array=w2004) -> (cluster=w2012:T11)
            n1121 = Unbundle(w2012) -> ("[0]"=w2011:cluster{dbl[], dbl[]})  [unwired: 8 out]
            n1122 = local read "NumPoints Log"() -> (w2008:dbl)
            n1123 = local read "Sat-Log Slider"() -> (w2002:dbl)
            n1124 = Unbundle(w2011) -> (w2010:dbl[], w2009:dbl[])
            n1125 = local write "Index 2"(w2002) -> ()
            n1126 = Array Subset(array=w2010, index=w2002, length=w2008) -> (w2000:dbl[])
            n1127 = Array Subset(array=w2009, index=w2002, length=w2008) -> (w1999:dbl[])
            n1128 = local write "Vg Array-Log-Used"(w1999) -> ()
            n1129 = local write "Sat Id-Log-Used"(w2000) -> ()
            n1130 = call "STS-Used.vi"("Id Used"=w2000, "Vg-Used"=w1999) -> ("STS"=w2001:dbl)  [unwired: 9 in]
            n1131 = Bundle(w2000, w1999) -> (w2006:cluster{dbl[], dbl[]})  [unwired: 1 in]
            n1132 = local write "New: STS"(w2001) -> ()
            n1133 = Build Array (concatenate)(w2004, w2003, w2006) -> (w2005:cluster{dbl[], dbl[]}[])
            n1134 = local write "Sat-Log"(w2005) -> ()
          }
          event "Save Changes?": Mouse Down {
            n1135 = event-data() -> ()  [unwired: 1 in, 5 out]
            n1136 = flat-sequence {
              tunnel: [w2019] -> w2017
              tunnel: [w2027] -> w2016
              tunnel: [w2020] -> w2015
              tunnel: w2017 -> [w2559]
              tunnel: w2016 -> [w2556]
              tunnel: [w2557] -> w2014
              tunnel: w2015 -> [w2557]
              tunnel: [w2556] -> w2013
              tunnel: w2014 -> [w2564]
              tunnel: w2013 -> [w2563]
              frame #0 {
                n1137 = Wait (ms)(milliseconds to wait=1) -> ()  [unwired: 1 out]
              }
              frame #1 {
                n1138 = local read "Transfer File"() -> (w2019:path)
                n1139 = local read "New: Temp"() -> (w2021:dbl)
                n1140 = local read "New: Length"() -> (w2025:dbl)
                n1141 = local read "New: Width"() -> (w2023:dbl)
                n1142 = To Single Precision Float(number=w2021) -> (single precision float=w2022:sgl)
                n1143 = Number To Decimal String(number=w2022) -> (decimal integer string=w2030:string)  [unwired: 1 in]
                n1144 = To Single Precision Float(number=w2023) -> (single precision float=w2024:sgl)
                n1145 = To Single Precision Float(number=w2025) -> (single precision float=w2026:sgl)
                n1146 = local read "Index"() -> (w2035:string)
                n1147 = Strip Path(path=w2019) -> (stripped path=w2040:path)  [unwired: 1 out]
                n1148 = Number To Decimal String(number=w2026) -> (decimal integer string=w2033:string)  [unwired: 1 in]
                n1149 = Number To Decimal String(number=w2024) -> (decimal integer string=w2034:string)  [unwired: 1 in]
                n1150 = Concatenate Strings("_", w2030, "K") -> (w2028:string)
                n1151 = call "Build Text"("Temp"=w2028, "Index"=w2035, "Length"=w2033, "Width"=w2034) -> ("Result"=w2036:string)  [unwired: 10 in, 1 out]
                n1152 = flat-sequence {
                  tunnel: [w2513] -> w2032
                  tunnel: w2032 -> [w2530]
                  frame #0 {
                    # "Makes Empty File for Transformer Data"
                    n1153 = local read "Transfer Folder"() -> (w2502:path)
                    n1154 = Build Path(base path=w2502, name or relative path="Stats") -> (appended path=w2504:path)
                    n1155 = call <vilib>:"Check if File or Folder Exists.vi"("path"=w2504) -> ("file or folder exists?"=w2505:bool, "dup path"=w2506:path)  [unwired: 8 in, 1 out]
                    n1156 = case shown="False" w2505 {
                      tunnel: [w2510 w2512] -> w2507
                      tunnel: w2506 -> [w2511 w2512]
                      frame False {
                        n1157 = Create Folder(path (use dialog)=w2511) -> (created path=w2510:path)  [unwired: 2 in, 2 out]
                      }
                      frame True {
                      }
                    }
                    n1158 = Build Path(base path=w2507, name or relative path="Tranformer Data.txt") -> (appended path=w2509:path)
                    n1159 = call-poly <vilib>:"Write To Spreadsheet File.vi"("append to file? (new file:F)"=TRUE, "file path (dialog if empty)"=w2509) -> ()  [unwired: 6 in, 1 out]
                  }
                  frame #1 {
                    # "Adds Headers if they don't exist"
                    n1160 = local read "Transfer Folder"() -> (w2519:path)
                    n1161 = Concatenate Strings("Stats\\", "Tranformer Data.txt") -> (w2520:string)
                    n1162 = Build Path(base path=w2519, name or relative path=w2520) -> (appended path=w2513:path)
                    n1163 = call-poly <vilib>:"Read From Spreadsheet File.vi"("file path (dialog if empty)"=w2513) -> ("first row"=w2518:string[])  [unwired: 6 in, 4 out]
                    n1164 = Search 1D Array(1D array=w2518, element="DeviceID") -> (index of element=w2516:i32)  [unwired: 1 in]
                    n1165 = Equal?(x=w2516, y=0) -> (x = y?=w2514:bool)
                    n1166 = case shown="False" w2514 {
                      tunnel: w2513 -> [w2524 _]
                      frame False {
                        n1167 = local read "Transformer \nHeaders"() -> (w2523:string[])
                        n1168 = call-poly <vilib>:"Write To Spreadsheet File.vi"("1D data"=w2523, "file path (dialog if empty)"=w2524) -> ()  [unwired: 6 in, 1 out]
                      }
                      frame True {
                      }
                    }
                  }
                  frame #2 {
                    # "Adds current device if it doesn't exist"
                    n1169 = local read "Current \nRecord"() -> (w2529:string[])
                    n1170 = Index Array(array=w2529, index=0) -> (element=w2528:string)
                    n1171 = local read "Transfer Folder"() -> (w2532:path)
                    n1172 = Concatenate Strings("Stats\\", "Tranformer Data.txt") -> (w2533:string)
                    n1173 = local write "Current Device ID"(w2528) -> ()
                    n1174 = local read "Current Device ID"() -> (w2538:string)
                    n1175 = Build Path(base path=w2532, name or relative path=w2533) -> (appended path=w2531:path)
                    n1176 = call-poly <vilib>:"Read From Spreadsheet File.vi"("file path (dialog if empty)"=w2531) -> ("all rows"=w2525:string[][])  [unwired: 6 in, 4 out]
                    n1177 = Index Array(array=w2525, index (col)=0) -> (element=w2526:string[])  [unwired: 1 in]
                    n1178 = Search 1D Array(1D array=w2526, element=w2538) -> (index of element=w2527:i32)  [unwired: 1 in]
                    n1179 = Equal?(x=w2527, y=-1) -> (x = y?=w2540:bool)
                    n1180 = case shown="False" w2540 {
                      tunnel: w2530 -> [w2543 w2554]
                      tunnel: w2527 -> [w2546 _]
                      tunnel: w2525 -> [w2547 _]
                      frame False {
                        n1181 = local read "Current \nRecord"() -> (w2545:string[])
                        n1182 = Replace Array Subset(array=w2547, new element=w2545, index (row)=w2546) -> (w2544:string[][])  [unwired: 1 in]
                        n1183 = flat-sequence {
                          tunnel: w2543 -> [w2548]
                          tunnel: w2544 -> [w2549]
                          tunnel: [w2549] -> w2542
                          tunnel: [w2548] -> w2541
                          tunnel: w2542 -> [w2551]
                          tunnel: w2541 -> [w2550]
                          frame #0 {
                            n1184 = Delete(path (use dialog)=w2548) -> ()  [unwired: 4 in, 3 out]
                          }
                          frame #1 {
                            n1185 = call-poly <vilib>:"Write To Spreadsheet File.vi"("append to file? (new file:F)"=TRUE, "2D data"=w2551, "file path (dialog if empty)"=w2550) -> ()  [unwired: 5 in, 1 out]
                          }
                        }
                      }
                      frame True {
                        n1186 = local read "Current \nRecord"() -> (w2553:string[])
                        n1187 = call-poly <vilib>:"Write To Spreadsheet File.vi"("append to file? (new file:F)"=TRUE, "1D data"=w2553, "file path (dialog if empty)"=w2554) -> ()  [unwired: 5 in, 1 out]
                      }
                    }
                  }
                }
                n1188 = Path To String(path=w2040) -> (string=w2038:string)
                n1189 = stacked-sequence {
                  tunnel: [_ _ _ _ _ _ _ _ _ _ _ _ _ w2473] -> w2020
                  tunnel: w2019 -> [w2042 _ _ _ _ _ _ _ _ _ _ _ _ _]
                  frame #0 {
                    n1190 = call-poly <vilib>:"Read From Spreadsheet File.vi"("file path (dialog if empty)"=w2042) -> ("all rows"=w2041:string[][])  [unwired: 6 in, 4 out]
                    n1191 = Array Size(array=w2041) -> (size(s)=w2046:i32[])
                    n1192 = Array Subset(array=w2041, index (row)=0, index (col)=0, length (col)=3) -> (w2050:string[][])  [unwired: 1 in]
                    n1193 = Index Array(array=w2046, index=0) -> (element=w2044:i32)
                    n1194 = Reshape Array(w2050, w2044) -> (w2043:string[])
                    n1195 = Search 1D Array(1D array=w2043, element="Dielectric (nm):") -> (index of element=w2053:i32)  [unwired: 1 in]
                    n1196 = Equal?(x=w2053, y=-1) -> (x = y?=w2052:bool)
                    n1197 = case shown="False" w2052 {
                      tunnel: w2041 -> [w2061 w2065]
                      tunnel: w2053 -> [w2057 _]
                      tunnel: [w2056 w2065] -> w2051
                      frame False {
                        n1198 = local read "New: Dielectric"() -> (w2063:dbl)
                        n1199 = Number To Fractional String(number=w2063) -> (F-format string=w2058:string)  [unwired: 3 in]
                        n1200 = Divide(x=w2057, y=3) -> (x/y=w2060:dbl)
                        n1201 = To Word Integer(number=w2060) -> (16bit integer=w2059:i16)
                        n1202 = Replace Array Subset(array=w2061, new element=w2058, index (row)=w2059, index (col)=1) -> (w2056:string[][])
                      }
                      frame True {
                      }
                    }
                    n1203 = local write "Save1 Array"(w2051) -> ()
                  }
                  frame #1 {
                    n1204 = local read "Save1 Array"() -> (w2067:string[][])
                    n1205 = Array Size(array=w2067) -> (size(s)=w2070:i32[])
                    n1206 = Array Subset(array=w2067, index (row)=0, index (col)=0, length (col)=3) -> (w2074:string[][])  [unwired: 1 in]
                    n1207 = Index Array(array=w2070, index=0) -> (element=w2068:i32)
                    n1208 = Reshape Array(w2074, w2068) -> (w2066:string[])
                    n1209 = Search 1D Array(1D array=w2066, element="Comments:") -> (index of element=w2077:i32)  [unwired: 1 in]
                    n1210 = Equal?(x=w2077, y=-1) -> (x = y?=w2076:bool)
                    n1211 = case shown="False" w2076 {
                      tunnel: w2067 -> [w2085 w2088]
                      tunnel: w2077 -> [w2082 _]
                      tunnel: [w2081 w2088] -> w2075
                      frame False {
                        n1212 = local read "Comments:"() -> (w2080:string)
                        n1213 = Divide(x=w2082, y=3) -> (x/y=w2084:dbl)
                        n1214 = To Word Integer(number=w2084) -> (16bit integer=w2083:i16)
                        n1215 = Replace Array Subset(array=w2085, new element=w2080, index (row)=w2083, index (col)=1) -> (w2081:string[][])
                      }
                      frame True {
                      }
                    }
                    n1216 = local write "Save1 Array"(w2075) -> ()
                  }
                  frame #2 {
                    n1217 = local read "Save1 Array"() -> (w2090:string[][])
                    n1218 = Array Size(array=w2090) -> (size(s)=w2093:i32[])
                    n1219 = Array Subset(array=w2090, index (row)=0, index (col)=0, length (col)=3) -> (w2097:string[][])  [unwired: 1 in]
                    n1220 = Index Array(array=w2093, index=0) -> (element=w2091:i32)
                    n1221 = Reshape Array(w2097, w2091) -> (w2089:string[])
                    n1222 = Search 1D Array(1D array=w2089, element="Length (um):") -> (index of element=w2100:i32)  [unwired: 1 in]
                    n1223 = Equal?(x=w2100, y=-1) -> (x = y?=w2099:bool)
                    n1224 = case shown="False" w2099 {
                      tunnel: w2090 -> [w2110 w2113]
                      tunnel: w2100 -> [w2107 _]
                      tunnel: [w2106 w2113] -> w2098
                      frame False {
                        n1225 = local read "New: Length"() -> (w2103:dbl)
                        n1226 = Divide(x=w2107, y=3) -> (x/y=w2109:dbl)
                        n1227 = Format Value(format string="%#g", value (0)=w2103) -> (output string=w2104:string)  [unwired: 1 in]
                        n1228 = To Word Integer(number=w2109) -> (16bit integer=w2108:i16)
                        n1229 = Replace Array Subset(array=w2110, new element=w2104, index (row)=w2108, index (col)=1) -> (w2106:string[][])
                      }
                      frame True {
                      }
                    }
                    n1230 = local write "Save1 Array"(w2098) -> ()
                  }
                  frame #3 {
                    n1231 = local read "Save1 Array"() -> (w2115:string[][])
                    n1232 = Array Size(array=w2115) -> (size(s)=w2120:i32[])
                    n1233 = Array Subset(array=w2115, index (row)=0, index (col)=0, length (col)=3) -> (w2116:string[][])  [unwired: 1 in]
                    n1234 = Index Array(array=w2120, index=0) -> (element=w2122:i32)
                    n1235 = Reshape Array(w2116, w2122) -> (w2114:string[])
                    n1236 = Search 1D Array(1D array=w2114, element="Width (um):") -> (index of element=w2125:i32)  [unwired: 1 in]
                    n1237 = Equal?(x=w2125, y=-1) -> (x = y?=w2124:bool)
                    n1238 = case shown="False" w2124 {
                      tunnel: w2125 -> [w2133 _]
                      tunnel: w2115 -> [w2132 w2138]
                      tunnel: [w2131 w2138] -> w2123
                      frame False {
                        n1239 = local read "New: Width"() -> (w2128:dbl)
                        n1240 = Divide(x=w2133, y=3) -> (x/y=w2135:dbl)
                        n1241 = To Word Integer(number=w2135) -> (16bit integer=w2134:i16)
                        n1242 = Format Value(format string="%#g", value (0)=w2128) -> (output string=w2129:string)  [unwired: 1 in]
                        n1243 = Replace Array Subset(array=w2132, new element=w2129, index (row)=w2134, index (col)=1) -> (w2131:string[][])
                      }
                      frame True {
                      }
                    }
                    n1244 = local write "Save1 Array"(w2123) -> ()
                  }
                  frame #4 {
                    w2148 = "Sample Temp (K):"
                    n1245 = local read "Save1 Array"() -> (w2140:string[][])
                    n1246 = Array Size(array=w2140) -> (size(s)=w2145:i32[])
                    n1247 = Array Subset(array=w2140, index (row)=0, index (col)=0, length (col)=3) -> (w2141:string[][])  [unwired: 1 in]
                    n1248 = Index Array(array=w2145, index=0) -> (element=w2147:i32)
                    n1249 = Reshape Array(w2141, w2147) -> (w2139:string[])
                    n1250 = Search 1D Array(1D array=w2139, element=w2148) -> (index of element=w2151:i32)  [unwired: 1 in]
                    n1251 = Equal?(x=w2151, y=-1) -> (x = y?=w2150:bool)
                    n1252 = case shown="True" w2150 {
                      tunnel: w2140 -> [w2160 w2174]
                      tunnel: w2151 -> [w2157 _]
                      tunnel: [w2156 w2173] -> w2149
                      tunnel: w2139 -> [_ w2176]
                      tunnel: w2148 -> [_ w2163]
                      frame False {
                        n1253 = local read "New: Temp"() -> (w2154:dbl)
                        n1254 = Divide(x=w2157, y=3) -> (x/y=w2159:dbl)
                        n1255 = Format Value(format string="%#g", value (0)=w2154) -> (output string=w2153:string)  [unwired: 1 in]
                        n1256 = To Word Integer(number=w2159) -> (16bit integer=w2158:i16)
                        n1257 = Replace Array Subset(array=w2160, new element=w2153, index (row)=w2158, index (col)=1) -> (w2156:string[][])
                      }
                      frame True {
                        n1258 = local read "New: Temp"() -> (w2165:dbl)
                        n1259 = Search 1D Array(1D array=w2176, element="Width (um):") -> (index of element=w2170:i32)  [unwired: 1 in]
                        n1260 = Divide(x=w2170, y=3) -> (x/y=w2171:dbl)
                        n1261 = To Word Integer(number=w2171) -> (16bit integer=w2169:i16)
                        n1262 = Format Value(format string="%#g", value (0)=w2165) -> (output string=w2164:string)  [unwired: 1 in]
                        n1263 = Build Array(w2163, w2164) -> (w2167:string[])
                        n1264 = Increment(x=w2169) -> (x+1=w2168:i16)
                        n1265 = Insert Into Array(array=w2174, index (row)=w2168, new element=w2167) -> (w2173:string[][])  [unwired: 1 in]
                      }
                    }
                    n1266 = local write "Save1 Array"(w2149) -> ()
                  }
                  frame #5 {
                    w2186 = "Mobility-Sat (cm^2/Vs):"
                    n1267 = local read "Save1 Array"() -> (w2178:string[][])
                    n1268 = Array Size(array=w2178) -> (size(s)=w2183:i32[])
                    n1269 = Array Subset(array=w2178, index (row)=0, index (col)=0, length (col)=3) -> (w2179:string[][])  [unwired: 1 in]
                    n1270 = Index Array(array=w2183, index=0) -> (element=w2185:i32)
                    n1271 = Reshape Array(w2179, w2185) -> (w2177:string[])
                    n1272 = Search 1D Array(1D array=w2177, element=w2186) -> (index of element=w2189:i32)  [unwired: 1 in]
                    n1273 = Equal?(x=w2189, y=-1) -> (x = y?=w2188:bool)
                    n1274 = case shown="True" w2188 {
                      tunnel: w2178 -> [w2198 w2206]
                      tunnel: w2189 -> [w2195 _]
                      tunnel: [w2194 w2205] -> w2187
                      tunnel: w2177 -> [_ w2203]
                      tunnel: w2186 -> [_ w2201]
                      frame False {
                        n1275 = local read "New: Mobility-Sat"() -> (w2191:dbl)
                        n1276 = Divide(x=w2195, y=3) -> (x/y=w2197:dbl)
                        n1277 = To Word Integer(number=w2197) -> (16bit integer=w2196:i16)
                        n1278 = Format Value(format string="%#g", value (0)=w2191) -> (output string=w2192:string)  [unwired: 1 in]
                        n1279 = Replace Array Subset(array=w2198, new element=w2192, index (row)=w2196, index (col)=1) -> (w2194:string[][])
                      }
                      frame True {
                        n1280 = local read "New: Mobility-Sat"() -> (w2207:dbl)
                        n1281 = Search 1D Array(1D array=w2203, element="Mobility (cm^2/Vs):") -> (index of element=w2210:i32)  [unwired: 1 in]
                        n1282 = Divide(x=w2210, y=3) -> (x/y=w2211:dbl)
                        n1283 = To Word Integer(number=w2211) -> (16bit integer=w2202:i16)
                        n1284 = Format Value(format string="%#g", value (0)=w2207) -> (output string=w2204:string)  [unwired: 1 in]
                        n1285 = Build Array(w2201, w2204) -> (w2209:string[])
                        n1286 = Replace Array Subset(array=w2206, new element=w2209, index (row)=w2202) -> (w2205:string[][])  [unwired: 1 in]
                      }
                    }
                    n1287 = local write "Save1 Array"(w2187) -> ()
                  }
                  frame #6 {
                    w2223 = "Mobility-Lin (cm^2/Vs):"
                    n1288 = local read "Save1 Array"() -> (w2214:string[][])
                    n1289 = Array Size(array=w2214) -> (size(s)=w2220:i32[])
                    n1290 = Array Subset(array=w2214, index (row)=0, index (col)=0, length (col)=3) -> (w2216:string[][])  [unwired: 1 in]
                    n1291 = Index Array(array=w2220, index=0) -> (element=w2222:i32)
                    n1292 = Reshape Array(w2216, w2222) -> (w2215:string[])
                    n1293 = Search 1D Array(1D array=w2215, element=w2223) -> (index of element=w2226:i32)  [unwired: 1 in]
                    n1294 = Equal?(x=w2226, y=-1) -> (x = y?=w2225:bool)
                    n1295 = case shown="True" w2225 {
                      tunnel: w2214 -> [w2235 w2241]
                      tunnel: w2226 -> [w2232 _]
                      tunnel: [w2231 w2240] -> w2224
                      tunnel: w2215 -> [_ w2239]
                      tunnel: w2223 -> [_ w2238]
                      frame False {
                        n1296 = local read "Calc: Mobility-Lin"() -> (w2228:dbl)
                        n1297 = Divide(x=w2232, y=3) -> (x/y=w2234:dbl)
                        n1298 = To Word Integer(number=w2234) -> (16bit integer=w2233:i16)
                        n1299 = Format Value(format string="%#g", value (0)=w2228) -> (output string=w2229:string)  [unwired: 1 in]
                        n1300 = Replace Array Subset(array=w2235, new element=w2229, index (row)=w2233, index (col)=1) -> (w2231:string[][])
                      }
                      frame True {
                        n1301 = local read "Calc: Mobility-Lin"() -> (w2242:dbl)
                        n1302 = Search 1D Array(1D array=w2239, element="Mobility-Sat (cm^2/Vs):") -> (index of element=w2247:i32)  [unwired: 1 in]
                        n1303 = Divide(x=w2247, y=3) -> (x/y=w2248:dbl)
                        n1304 = To Word Integer(number=w2248) -> (16bit integer=w2246:i16)
                        n1305 = Format Value(format string="%#g", value (0)=w2242) -> (output string=w2251:string)  [unwired: 1 in]
                        n1306 = Build Array(w2238, w2251) -> (w2244:string[])
                        n1307 = Increment(x=w2246) -> (x+1=w2245:i16)
                        n1308 = Insert Into Array(array=w2241, index (row)=w2245, new element=w2244) -> (w2240:string[][])  [unwired: 1 in]
                      }
                    }
                    n1309 = local write "Save1 Array"(w2224) -> ()
                  }
                  frame #7 {
                    w2261 = "On/Off I-Sat:"
                    n1310 = local read "Save1 Array"() -> (w2252:string[][])
                    n1311 = Array Size(array=w2252) -> (size(s)=w2258:i32[])
                    n1312 = Array Subset(array=w2252, index (row)=0, index (col)=0, length (col)=3) -> (w2254:string[][])  [unwired: 1 in]
                    n1313 = Index Array(array=w2258, index=0) -> (element=w2260:i32)
                    n1314 = Reshape Array(w2254, w2260) -> (w2253:string[])
                    n1315 = Search 1D Array(1D array=w2253, element=w2261) -> (index of element=w2264:i32)  [unwired: 1 in]
                    n1316 = Equal?(x=w2264, y=-1) -> (x = y?=w2263:bool)
                    n1317 = case shown="True" w2263 {
                      tunnel: w2252 -> [w2273 w2280]
                      tunnel: w2264 -> [w2270 _]
                      tunnel: [w2269 w2281] -> w2262
                      tunnel: w2253 -> [_ w2278]
                      tunnel: w2261 -> [_ w2276]
                      frame False {
                        n1318 = local read "Calc: On/Off"() -> (w2266:dbl)
                        n1319 = Divide(x=w2270, y=3) -> (x/y=w2272:dbl)
                        n1320 = To Word Integer(number=w2272) -> (16bit integer=w2271:i16)
                        n1321 = Format Value(format string="%#g", value (0)=w2266) -> (output string=w2267:string)  [unwired: 1 in]
                        n1322 = Replace Array Subset(array=w2273, new element=w2267, index (row)=w2271, index (col)=1) -> (w2269:string[][])
                      }
                      frame True {
                        n1323 = local read "Calc: On/Off"() -> (w2282:dbl)
                        n1324 = Search 1D Array(1D array=w2278, element="On/Off Current:") -> (index of element=w2285:i32)  [unwired: 1 in]
                        n1325 = Divide(x=w2285, y=3) -> (x/y=w2286:dbl)
                        n1326 = To Word Integer(number=w2286) -> (16bit integer=w2277:i16)
                        n1327 = Format Value(format string="%#g", value (0)=w2282) -> (output string=w2279:string)  [unwired: 1 in]
                        n1328 = Build Array(w2276, w2279) -> (w2284:string[])
                        n1329 = Replace Array Subset(array=w2280, new element=w2284, index (row)=w2277) -> (w2281:string[][])  [unwired: 1 in]
                      }
                    }
                    n1330 = local write "Save1 Array"(w2262) -> ()
                  }
                  frame #8 {
                    w2298 = "Off I-Sat (A):"
                    n1331 = local read "Save1 Array"() -> (w2289:string[][])
                    n1332 = Array Size(array=w2289) -> (size(s)=w2295:i32[])
                    n1333 = Array Subset(array=w2289, index (row)=0, index (col)=0, length (col)=3) -> (w2291:string[][])  [unwired: 1 in]
                    n1334 = Index Array(array=w2295, index=0) -> (element=w2297:i32)
                    n1335 = Reshape Array(w2291, w2297) -> (w2290:string[])
                    n1336 = Search 1D Array(1D array=w2290, element=w2298) -> (index of element=w2301:i32)  [unwired: 1 in]
                    n1337 = Equal?(x=w2301, y=-1) -> (x = y?=w2300:bool)
                    n1338 = case shown="True" w2300 {
                      tunnel: w2289 -> [w2310 w2316]
                      tunnel: w2301 -> [w2307 _]
                      tunnel: [w2306 w2315] -> w2299
                      tunnel: w2290 -> [_ w2314]
                      tunnel: w2298 -> [_ w2313]
                      frame False {
                        n1339 = local read "Calc: Off I-Sat"() -> (w2305:dbl)
                        n1340 = Divide(x=w2307, y=3) -> (x/y=w2309:dbl)
                        n1341 = Format Value(format string="%#g", value (0)=w2305) -> (output string=w2303:string)  [unwired: 1 in]
                        n1342 = To Word Integer(number=w2309) -> (16bit integer=w2308:i16)
                        n1343 = Replace Array Subset(array=w2310, new element=w2303, index (row)=w2308, index (col)=1) -> (w2306:string[][])
                      }
                      frame True {
                        n1344 = local read "Calc: Off I-Sat"() -> (w2317:dbl)
                        n1345 = Search 1D Array(1D array=w2314, element="On/Off I-Sat:") -> (index of element=w2322:i32)  [unwired: 1 in]
                        n1346 = Divide(x=w2322, y=3) -> (x/y=w2323:dbl)
                        n1347 = To Word Integer(number=w2323) -> (16bit integer=w2321:i16)
                        n1348 = Format Value(format string="%#g", value (0)=w2317) -> (output string=w2326:string)  [unwired: 1 in]
                        n1349 = Build Array(w2313, w2326) -> (w2319:string[])
                        n1350 = Increment(x=w2321) -> (x+1=w2320:i16)
                        n1351 = Insert Into Array(array=w2316, index (row)=w2320, new element=w2319) -> (w2315:string[][])  [unwired: 1 in]
                      }
                    }
                    n1352 = local write "Save1 Array"(w2299) -> ()
                  }
                  frame #9 {
                    w2328 = "Vt-Sat (V):"
                    n1353 = local read "Save1 Array"() -> (w2329:string[][])
                    n1354 = Array Size(array=w2329) -> (size(s)=w2334:i32[])
                    n1355 = Array Subset(array=w2329, index (row)=0, index (col)=0, length (col)=3) -> (w2330:string[][])  [unwired: 1 in]
                    n1356 = Index Array(array=w2334, index=0) -> (element=w2336:i32)
                    n1357 = Reshape Array(w2330, w2336) -> (w2327:string[])
                    n1358 = Search 1D Array(1D array=w2327, element=w2328) -> (index of element=w2339:i32)  [unwired: 1 in]
                    n1359 = Equal?(x=w2339, y=-1) -> (x = y?=w2338:bool)
                    n1360 = case shown="True" w2338 {
                      tunnel: w2329 -> [w2346 w2355]
                      tunnel: w2339 -> [w2342 _]
                      tunnel: [w2341 w2354] -> w2337
                      tunnel: w2328 -> [_ w2353]
                      tunnel: w2327 -> [_ w2352]
                      frame False {
                        n1361 = local read "New: VT-Sat"() -> (w2348:dbl)
                        n1362 = Number To Fractional String(number=w2348) -> (F-format string=w2343:string)  [unwired: 3 in]
                        n1363 = Divide(x=w2342, y=3) -> (x/y=w2345:dbl)
                        n1364 = To Word Integer(number=w2345) -> (16bit integer=w2344:i16)
                        n1365 = Replace Array Subset(array=w2346, new element=w2343, index (row)=w2344, index (col)=1) -> (w2341:string[][])
                      }
                      frame True {
                        n1366 = local read "New: VT-Sat"() -> (w2356:dbl)
                        n1367 = Search 1D Array(1D array=w2352, element="Threshold V (V):") -> (index of element=w2351:i32)  [unwired: 1 in]
                        n1368 = Divide(x=w2351, y=3) -> (x/y=w2359:dbl)
                        n1369 = To Word Integer(number=w2359) -> (16bit integer=w2350:i16)
                        n1370 = Format Value(format string="%#g", value (0)=w2356) -> (output string=w2362:string)  [unwired: 1 in]
                        n1371 = Build Array(w2353, w2362) -> (w2358:string[])
                        n1372 = Replace Array Subset(array=w2355, new element=w2358, index (row)=w2350) -> (w2354:string[][])  [unwired: 1 in]
                      }
                    }
                    n1373 = local write "Save1 Array"(w2337) -> ()
                  }
                  frame #10 {
                    n1374 = local read "Save1 Array"() -> (w2363:string[][])
                    n1375 = Array Size(array=w2363) -> (size(s)=w2369:i32[])
                    n1376 = Array Subset(array=w2363, index (row)=0, index (col)=0, length (col)=3) -> (w2365:string[][])  [unwired: 1 in]
                    n1377 = Index Array(array=w2369, index=0) -> (element=w2371:i32)
                    n1378 = Reshape Array(w2365, w2371) -> (w2364:string[])
                    n1379 = Search 1D Array(1D array=w2364, element="VT-Lin (V):") -> (index of element=w2374:i32)  [unwired: 1 in]
                    n1380 = Equal?(x=w2374, y=-1) -> (x = y?=w2373:bool)
                    n1381 = case shown="False" w2373 {
                      tunnel: w2363 -> [w2384 w2387]
                      tunnel: w2374 -> [w2381 _]
                      tunnel: [w2380 w2387] -> w2372
                      frame False {
                        n1382 = local read "New: VT-Lin"() -> (w2378:dbl)
                        n1383 = Divide(x=w2381, y=3) -> (x/y=w2383:dbl)
                        n1384 = Format Value(format string="%#g", value (0)=w2378) -> (output string=w2377:string)  [unwired: 1 in]
                        n1385 = To Word Integer(number=w2383) -> (16bit integer=w2382:i16)
                        n1386 = Replace Array Subset(array=w2384, new element=w2377, index (row)=w2382, index (col)=1) -> (w2380:string[][])
                      }
                      frame True {
                      }
                    }
                    n1387 = local write "Save1 Array"(w2372) -> ()
                  }
                  frame #11 {
                    w2388 = "STS-Sat (V/decade):"
                    n1388 = local read "Save1 Array"() -> (w2390:string[][])
                    n1389 = Array Size(array=w2390) -> (size(s)=w2395:i32[])
                    n1390 = Array Subset(array=w2390, index (row)=0, index (col)=0, length (col)=3) -> (w2391:string[][])  [unwired: 1 in]
                    n1391 = Index Array(array=w2395, index=0) -> (element=w2397:i32)
                    n1392 = Reshape Array(w2391, w2397) -> (w2389:string[])
                    n1393 = Search 1D Array(1D array=w2389, element=w2388) -> (index of element=w2400:i32)  [unwired: 1 in]
                    n1394 = Equal?(x=w2400, y=-1) -> (x = y?=w2399:bool)
                    n1395 = case shown="True" w2399 {
                      tunnel: w2390 -> [w2409 w2415]
                      tunnel: w2400 -> [w2406 _]
                      tunnel: [w2405 w2416] -> w2398
                      tunnel: w2389 -> [_ w2414]
                      tunnel: w2388 -> [_ w2413]
                      frame False {
                        n1396 = local read "New: STS"() -> (w2403:dbl)
                        n1397 = Divide(x=w2406, y=3) -> (x/y=w2408:dbl)
                        n1398 = Format Value(format string="%#g", value (0)=w2403) -> (output string=w2402:string)  [unwired: 1 in]
                        n1399 = To Word Integer(number=w2408) -> (16bit integer=w2407:i16)
                        n1400 = Replace Array Subset(array=w2409, new element=w2402, index (row)=w2407, index (col)=1) -> (w2405:string[][])
                      }
                      frame True {
                        n1401 = local read "New: STS"() -> (w2417:dbl)
                        n1402 = Search 1D Array(1D array=w2414, element="S.T.S. (V/decade):") -> (index of element=w2420:i32)  [unwired: 1 in]
                        n1403 = Divide(x=w2420, y=3) -> (x/y=w2421:dbl)
                        n1404 = To Word Integer(number=w2421) -> (16bit integer=w2412:i16)
                        n1405 = Format Value(format string="%#g", value (0)=w2417) -> (output string=w2424:string)  [unwired: 1 in]
                        n1406 = Build Array(w2413, w2424) -> (w2419:string[])
                        n1407 = Replace Array Subset(array=w2415, new element=w2419, index (row)=w2412) -> (w2416:string[][])  [unwired: 1 in]
                      }
                    }
                    n1408 = local write "Save1 Array"(w2398) -> ()
                  }
                  frame #12 {
                    w2425 = "Trap Density-VT (Traps/Vcm^2):"
                    n1409 = local read "Save1 Array"() -> (w2427:string[][])
                    n1410 = Array Size(array=w2427) -> (size(s)=w2432:i32[])
                    n1411 = Array Subset(array=w2427, index (row)=0, index (col)=0, length (col)=3) -> (w2428:string[][])  [unwired: 1 in]
                    n1412 = Index Array(array=w2432, index=0) -> (element=w2434:i32)
                    n1413 = Reshape Array(w2428, w2434) -> (w2426:string[])
                    n1414 = Search 1D Array(1D array=w2426, element=w2425) -> (index of element=w2437:i32)  [unwired: 1 in]
                    n1415 = Equal?(x=w2437, y=-1) -> (x = y?=w2436:bool)
                    n1416 = case shown="True" w2436 {
                      tunnel: w2427 -> [w2446 w2451]
                      tunnel: w2437 -> [w2442 _]
                      tunnel: [w2441 w2452] -> w2435
                      tunnel: w2426 -> [_ w2450]
                      tunnel: w2425 -> [_ w2449]
                      frame False {
                        n1417 = local read "New: Trap Density-VT"() -> (w2440:dbl)
                        n1418 = Format Value(format string="%#g", value (0)=w2440) -> (output string=w2443:string)  [unwired: 1 in]
                        n1419 = Divide(x=w2442, y=3) -> (x/y=w2445:dbl)
                        n1420 = To Word Integer(number=w2445) -> (16bit integer=w2444:i16)
                        n1421 = Replace Array Subset(array=w2446, new element=w2443, index (row)=w2444, index (col)=1) -> (w2441:string[][])
                      }
                      frame True {
                        n1422 = local read "New: Trap Density-VT"() -> (w2462:dbl)
                        n1423 = Search 1D Array(1D array=w2450, element="STS-Sat (V/decade):") -> (index of element=w2457:i32)  [unwired: 1 in]
                        n1424 = Divide(x=w2457, y=3) -> (x/y=w2456:dbl)
                        n1425 = To Word Integer(number=w2456) -> (16bit integer=w2458:i16)
                        n1426 = Format Value(format string="%#g", value (0)=w2462) -> (output string=w2453:string)  [unwired: 1 in]
                        n1427 = Build Array(w2449, w2453) -> (w2460:string[])
                        n1428 = Increment(x=w2458) -> (x+1=w2459:i16)
                        n1429 = Insert Into Array(array=w2451, index (row)=w2459, new element=w2460) -> (w2452:string[][])  [unwired: 1 in]
                      }
                    }
                    n1430 = local write "Save1 Array"(w2435) -> ()
                  }
                  frame #13 {
                    w2463 = "Trap Density-STS (Traps/Vcm^2):"
                    n1431 = local read "Save1 Array"() -> (w2465:string[][])
                    n1432 = Array Size(array=w2465) -> (size(s)=w2470:i32[])
                    n1433 = Array Subset(array=w2465, index (row)=0, index (col)=0, length (col)=3) -> (w2466:string[][])  [unwired: 1 in]
                    n1434 = Index Array(array=w2470, index=0) -> (element=w2472:i32)
                    n1435 = Reshape Array(w2466, w2472) -> (w2464:string[])
                    n1436 = Search 1D Array(1D array=w2464, element=w2463) -> (index of element=w2475:i32)  [unwired: 1 in]
                    n1437 = Equal?(x=w2475, y=-1) -> (x = y?=w2474:bool)
                    n1438 = case shown="True" w2474 {
                      tunnel: w2465 -> [w2484 w2489]
                      tunnel: w2475 -> [w2481 _]
                      tunnel: [w2480 w2490] -> w2473
                      tunnel: w2464 -> [_ w2488]
                      tunnel: w2463 -> [_ w2487]
                      frame False {
                        n1439 = local read "New: Trap Density-STS"() -> (w2478:dbl)
                        n1440 = Divide(x=w2481, y=3) -> (x/y=w2483:dbl)
                        n1441 = To Word Integer(number=w2483) -> (16bit integer=w2482:i16)
                        n1442 = Format Value(format string="%#g", value (0)=w2478) -> (output string=w2477:string)  [unwired: 1 in]
                        n1443 = Replace Array Subset(array=w2484, new element=w2477, index (row)=w2482, index (col)=1) -> (w2480:string[][])
                      }
                      frame True {
                        n1444 = local read "New: Trap Density-STS"() -> (w2491:dbl)
                        n1445 = Search 1D Array(1D array=w2488, element="Trap Density-VT (Traps/Vcm^2):") -> (index of element=w2496:i32)  [unwired: 1 in]
                        n1446 = Divide(x=w2496, y=3) -> (x/y=w2497:dbl)
                        n1447 = To Word Integer(number=w2497) -> (16bit integer=w2495:i16)
                        n1448 = Format Value(format string="%#g", value (0)=w2491) -> (output string=w2500:string)  [unwired: 1 in]
                        n1449 = Build Array(w2487, w2500) -> (w2493:string[])
                        n1450 = Increment(x=w2495) -> (x+1=w2494:i16)
                        n1451 = Insert Into Array(array=w2489, index (row)=w2494, new element=w2493) -> (w2490:string[][])  [unwired: 1 in]
                      }
                    }
                    n1452 = local write "Save1 Array"(w2473) -> ()
                  }
                }
                n1453 = Concatenate Strings(w2038, "\\", w2036) -> (w2037:string)
                n1454 = String To Path(string=w2037) -> (path=w2027:path)
                n1455 = disable-structure shown="Disabled" {
                  frame Disabled {
                  }
                  frame Enabled {
                  }
                }
              }
              frame #2 {
                n1456 = Equal?(x=w2559, y=w2556) -> (x = y?=w2558:bool)
                n1457 = case shown="False" w2558 {
                  tunnel: w2559 -> [w2562 _]
                  tunnel: w2556 -> [w2561 _]
                  frame False {
                    n1458 = Move(source path=w2562, 9:TRUE, 10:w2561) -> ()  [unwired: 2 in, 3 out]
                  }
                  frame True {
                  }
                }
              }
              frame #3 {
                n1459 = local write "Transfer File"(w2563) -> ()
                n1460 = call-poly <vilib>:"Write To Spreadsheet File.vi"("2D data"=w2564, "file path (dialog if empty)"=w2563) -> ()  [unwired: 6 in, 1 out]
              }
            }
          }
          event "Save Changes? 2": Mouse Down {
            n1461 = event-data() -> ()  [unwired: 1 in, 5 out]
            n1462 = stacked-sequence {
              seq-local: [w2622 _ _ _ _] -> [_ w3105 _ _ _]
              seq-local: [w2621 _ _ _ _] -> [_ w3106 _ _ _]
              seq-local: [w2621 _ _ _ _] -> [_ w3104 _ _ _]
              seq-local: [w2623 _ _ _ _] -> [_ w3102 _ _ _]
              seq-local: [_ w3106 _ _ _] -> [_ _ w3111 _ _]
              seq-local: [_ w3102 _ _ _] -> [_ _ w3110 _ _]
              frame #0 {
                n1463 = local read "Transfer File"() -> (w2622:path)
                n1464 = local read "New: Temp"() -> (w2625:dbl)
                n1465 = local read "New: Length"() -> (w2628:dbl)
                n1466 = local read "New: Width"() -> (w2626:dbl)
                n1467 = To Word Integer(number=w2625) -> (16bit integer=w2624:i16)
                n1468 = Number To Decimal String(number=w2624) -> (decimal integer string=w2632:string)  [unwired: 1 in]
                n1469 = To Single Precision Float(number=w2626) -> (single precision float=w2627:sgl)
                n1470 = To Single Precision Float(number=w2628) -> (single precision float=w2629:sgl)
                n1471 = local read "Index"() -> (w2636:string)
                n1472 = Strip Path(path=w2622) -> (stripped path=w2641:path)  [unwired: 1 out]
                n1473 = Number To Decimal String(number=w2629) -> (decimal integer string=w2634:string)  [unwired: 1 in]
                n1474 = Number To Decimal String(number=w2627) -> (decimal integer string=w2635:string)  [unwired: 1 in]
                n1475 = Concatenate Strings("_", w2632, "K") -> (w2630:string)
                n1476 = call "Build Text2"("Temp"=w2630, "Index"=w2636, "Length"=w2634, "Width"=w2635) -> ("Result"=w2637:string)  [unwired: 10 in, 1 out]
                n1477 = Path To String(path=w2641) -> (string=w2639:string)
                n1478 = Concatenate Strings(w2639, "\\", w2637) -> (w2638:string)
                n1479 = stacked-sequence {
                  tunnel: [_ _ _ _ _ _ _ _ _ _ _ _ _ w3064] -> _
                  tunnel: w2622 -> [w2643 _ _ _ _ _ _ _ _ _ _ _ _ _]
                  tunnel: [_ _ _ _ _ _ _ _ _ _ _ _ _ w3064] -> w2623
                  frame #0 {
                    n1480 = call-poly <vilib>:"Read From Spreadsheet File.vi"("file path (dialog if empty)"=w2643) -> ("all rows"=w2642:string[][])  [unwired: 6 in, 4 out]
                    n1481 = Array Size(array=w2642) -> (size(s)=w2647:i32[])
                    n1482 = Array Subset(array=w2642, index (row)=0, index (col)=0, length (col)=3) -> (w2651:string[][])  [unwired: 1 in]
                    n1483 = Index Array(array=w2647, index=0) -> (element=w2645:i32)
                    n1484 = Reshape Array(w2651, w2645) -> (w2644:string[])
                    n1485 = Search 1D Array(1D array=w2644, element="Dielectric (nm):") -> (index of element=w2654:i32)  [unwired: 1 in]
                    n1486 = Equal?(x=w2654, y=-1) -> (x = y?=w2653:bool)
                    n1487 = case shown="False" w2653 {
                      tunnel: w2642 -> [w2662 w2666]
                      tunnel: w2654 -> [w2658 _]
                      tunnel: [w2657 w2666] -> w2652
                      frame False {
                        n1488 = local read "New: Dielectric"() -> (w2664:dbl)
                        n1489 = Number To Fractional String(number=w2664) -> (F-format string=w2659:string)  [unwired: 3 in]
                        n1490 = Divide(x=w2658, y=3) -> (x/y=w2661:dbl)
                        n1491 = To Word Integer(number=w2661) -> (16bit integer=w2660:i16)
                        n1492 = Replace Array Subset(array=w2662, new element=w2659, index (row)=w2660, index (col)=1) -> (w2657:string[][])
                      }
                      frame True {
                      }
                    }
                    n1493 = local write "Save1 Array"(w2652) -> ()
                  }
                  frame #1 {
                    n1494 = local read "Save1 Array"() -> (w2668:string[][])
                    n1495 = Array Size(array=w2668) -> (size(s)=w2671:i32[])
                    n1496 = Array Subset(array=w2668, index (row)=0, index (col)=0, length (col)=3) -> (w2675:string[][])  [unwired: 1 in]
                    n1497 = Index Array(array=w2671, index=0) -> (element=w2669:i32)
                    n1498 = Reshape Array(w2675, w2669) -> (w2667:string[])
                    n1499 = Search 1D Array(1D array=w2667, element="Comments:") -> (index of element=w2678:i32)  [unwired: 1 in]
                    n1500 = Equal?(x=w2678, y=-1) -> (x = y?=w2677:bool)
                    n1501 = case shown="False" w2677 {
                      tunnel: w2668 -> [w2686 w2689]
                      tunnel: w2678 -> [w2683 _]
                      tunnel: [w2682 w2689] -> w2676
                      frame False {
                        n1502 = local read "Comments:"() -> (w2681:string)
                        n1503 = Divide(x=w2683, y=3) -> (x/y=w2685:dbl)
                        n1504 = To Word Integer(number=w2685) -> (16bit integer=w2684:i16)
                        n1505 = Replace Array Subset(array=w2686, new element=w2681, index (row)=w2684, index (col)=1) -> (w2682:string[][])
                      }
                      frame True {
                      }
                    }
                    n1506 = local write "Save1 Array"(w2676) -> ()
                  }
                  frame #2 {
                    n1507 = local read "Save1 Array"() -> (w2691:string[][])
                    n1508 = Array Size(array=w2691) -> (size(s)=w2694:i32[])
                    n1509 = Array Subset(array=w2691, index (row)=0, index (col)=0, length (col)=3) -> (w2698:string[][])  [unwired: 1 in]
                    n1510 = Index Array(array=w2694, index=0) -> (element=w2692:i32)
                    n1511 = Reshape Array(w2698, w2692) -> (w2690:string[])
                    n1512 = Search 1D Array(1D array=w2690, element="Length (um):") -> (index of element=w2701:i32)  [unwired: 1 in]
                    n1513 = Equal?(x=w2701, y=-1) -> (x = y?=w2700:bool)
                    n1514 = case shown="False" w2700 {
                      tunnel: w2691 -> [w2711 w2714]
                      tunnel: w2701 -> [w2708 _]
                      tunnel: [w2707 w2714] -> w2699
                      frame False {
                        n1515 = local read "New: Length"() -> (w2704:dbl)
                        n1516 = Divide(x=w2708, y=3) -> (x/y=w2710:dbl)
                        n1517 = Format Value(format string="%#g", value (0)=w2704) -> (output string=w2705:string)  [unwired: 1 in]
                        n1518 = To Word Integer(number=w2710) -> (16bit integer=w2709:i16)
                        n1519 = Replace Array Subset(array=w2711, new element=w2705, index (row)=w2709, index (col)=1) -> (w2707:string[][])
                      }
                      frame True {
                      }
                    }
                    n1520 = local write "Save1 Array"(w2699) -> ()
                  }
                  frame #3 {
                    n1521 = local read "Save1 Array"() -> (w2716:string[][])
                    n1522 = Array Size(array=w2716) -> (size(s)=w2721:i32[])
                    n1523 = Array Subset(array=w2716, index (row)=0, index (col)=0, length (col)=3) -> (w2717:string[][])  [unwired: 1 in]
                    n1524 = Index Array(array=w2721, index=0) -> (element=w2723:i32)
                    n1525 = Reshape Array(w2717, w2723) -> (w2715:string[])
                    n1526 = Search 1D Array(1D array=w2715, element="Width (um):") -> (index of element=w2726:i32)  [unwired: 1 in]
                    n1527 = Equal?(x=w2726, y=-1) -> (x = y?=w2725:bool)
                    n1528 = case shown="False" w2725 {
                      tunnel: w2726 -> [w2734 _]
                      tunnel: w2716 -> [w2733 w2739]
                      tunnel: [w2732 w2739] -> w2724
                      frame False {
                        n1529 = local read "New: Width"() -> (w2729:dbl)
                        n1530 = Divide(x=w2734, y=3) -> (x/y=w2736:dbl)
                        n1531 = To Word Integer(number=w2736) -> (16bit integer=w2735:i16)
                        n1532 = Format Value(format string="%#g", value (0)=w2729) -> (output string=w2730:string)  [unwired: 1 in]
                        n1533 = Replace Array Subset(array=w2733, new element=w2730, index (row)=w2735, index (col)=1) -> (w2732:string[][])
                      }
                      frame True {
                      }
                    }
                    n1534 = local write "Save1 Array"(w2724) -> ()
                  }
                  frame #4 {
                    w2749 = "Sample Temp (K):"
                    n1535 = local read "Save1 Array"() -> (w2741:string[][])
                    n1536 = Array Size(array=w2741) -> (size(s)=w2746:i32[])
                    n1537 = Array Subset(array=w2741, index (row)=0, index (col)=0, length (col)=3) -> (w2742:string[][])  [unwired: 1 in]
                    n1538 = Index Array(array=w2746, index=0) -> (element=w2748:i32)
                    n1539 = Reshape Array(w2742, w2748) -> (w2740:string[])
                    n1540 = Search 1D Array(1D array=w2740, element=w2749) -> (index of element=w2752:i32)  [unwired: 1 in]
                    n1541 = Equal?(x=w2752, y=-1) -> (x = y?=w2751:bool)
                    n1542 = case shown="True" w2751 {
                      tunnel: w2741 -> [w2761 w2775]
                      tunnel: w2752 -> [w2758 _]
                      tunnel: [w2757 w2774] -> w2750
                      tunnel: w2740 -> [_ w2777]
                      tunnel: w2749 -> [_ w2764]
                      frame False {
                        n1543 = local read "New: Temp"() -> (w2755:dbl)
                        n1544 = Divide(x=w2758, y=3) -> (x/y=w2760:dbl)
                        n1545 = Format Value(format string="%#g", value (0)=w2755) -> (output string=w2754:string)  [unwired: 1 in]
                        n1546 = To Word Integer(number=w2760) -> (16bit integer=w2759:i16)
                        n1547 = Replace Array Subset(array=w2761, new element=w2754, index (row)=w2759, index (col)=1) -> (w2757:string[][])
                      }
                      frame True {
                        n1548 = local read "New: Temp"() -> (w2766:dbl)
                        n1549 = Search 1D Array(1D array=w2777, element="Width (um):") -> (index of element=w2771:i32)  [unwired: 1 in]
                        n1550 = Divide(x=w2771, y=3) -> (x/y=w2772:dbl)
                        n1551 = To Word Integer(number=w2772) -> (16bit integer=w2770:i16)
                        n1552 = Format Value(format string="%#g", value (0)=w2766) -> (output string=w2765:string)  [unwired: 1 in]
                        n1553 = Build Array(w2764, w2765) -> (w2768:string[])
                        n1554 = Increment(x=w2770) -> (x+1=w2769:i16)
                        n1555 = Insert Into Array(array=w2775, index (row)=w2769, new element=w2768) -> (w2774:string[][])  [unwired: 1 in]
                      }
                    }
                    n1556 = local write "Save1 Array"(w2750) -> ()
                  }
                  frame #5 {
                    w2787 = "Mobility-Sat (cm^2/Vs):"
                    n1557 = local read "Save1 Array"() -> (w2779:string[][])
                    n1558 = Array Size(array=w2779) -> (size(s)=w2784:i32[])
                    n1559 = Array Subset(array=w2779, index (row)=0, index (col)=0, length (col)=3) -> (w2780:string[][])  [unwired: 1 in]
                    n1560 = Index Array(array=w2784, index=0) -> (element=w2786:i32)
                    n1561 = Reshape Array(w2780, w2786) -> (w2778:string[])
                    n1562 = Search 1D Array(1D array=w2778, element=w2787) -> (index of element=w2790:i32)  [unwired: 1 in]
                    n1563 = Equal?(x=w2790, y=-1) -> (x = y?=w2789:bool)
                    n1564 = case shown="True" w2789 {
                      tunnel: w2779 -> [w2799 w2807]
                      tunnel: w2790 -> [w2796 _]
                      tunnel: [w2795 w2806] -> w2788
                      tunnel: w2778 -> [_ w2804]
                      tunnel: w2787 -> [_ w2802]
                      frame False {
                        n1565 = local read "New: Mobility-Sat"() -> (w2792:dbl)
                        n1566 = Divide(x=w2796, y=3) -> (x/y=w2798:dbl)
                        n1567 = To Word Integer(number=w2798) -> (16bit integer=w2797:i16)
                        n1568 = Format Value(format string="%#g", value (0)=w2792) -> (output string=w2793:string)  [unwired: 1 in]
                        n1569 = Replace Array Subset(array=w2799, new element=w2793, index (row)=w2797, index (col)=1) -> (w2795:string[][])
                      }
                      frame True {
                        n1570 = local read "New: Mobility-Sat"() -> (w2808:dbl)
                        n1571 = Search 1D Array(1D array=w2804, element="Mobility (cm^2/Vs):") -> (index of element=w2811:i32)  [unwired: 1 in]
                        n1572 = Divide(x=w2811, y=3) -> (x/y=w2812:dbl)
                        n1573 = To Word Integer(number=w2812) -> (16bit integer=w2803:i16)
                        n1574 = Format Value(format string="%#g", value (0)=w2808) -> (output string=w2805:string)  [unwired: 1 in]
                        n1575 = Build Array(w2802, w2805) -> (w2810:string[])
                        n1576 = Replace Array Subset(array=w2807, new element=w2810, index (row)=w2803) -> (w2806:string[][])  [unwired: 1 in]
                      }
                    }
                    n1577 = local write "Save1 Array"(w2788) -> ()
                  }
                  frame #6 {
                    w2824 = "Mobility-Lin (cm^2/Vs):"
                    n1578 = local read "Save1 Array"() -> (w2815:string[][])
                    n1579 = Array Size(array=w2815) -> (size(s)=w2821:i32[])
                    n1580 = Array Subset(array=w2815, index (row)=0, index (col)=0, length (col)=3) -> (w2817:string[][])  [unwired: 1 in]
                    n1581 = Index Array(array=w2821, index=0) -> (element=w2823:i32)
                    n1582 = Reshape Array(w2817, w2823) -> (w2816:string[])
                    n1583 = Search 1D Array(1D array=w2816, element=w2824) -> (index of element=w2827:i32)  [unwired: 1 in]
                    n1584 = Equal?(x=w2827, y=-1) -> (x = y?=w2826:bool)
                    n1585 = case shown="True" w2826 {
                      tunnel: w2815 -> [w2836 w2842]
                      tunnel: w2827 -> [w2833 _]
                      tunnel: [w2832 w2841] -> w2825
                      tunnel: w2816 -> [_ w2840]
                      tunnel: w2824 -> [_ w2839]
                      frame False {
                        n1586 = local read "Calc: Mobility-Lin"() -> (w2829:dbl)
                        n1587 = Divide(x=w2833, y=3) -> (x/y=w2835:dbl)
                        n1588 = To Word Integer(number=w2835) -> (16bit integer=w2834:i16)
                        n1589 = Format Value(format string="%#g", value (0)=w2829) -> (output string=w2830:string)  [unwired: 1 in]
                        n1590 = Replace Array Subset(array=w2836, new element=w2830, index (row)=w2834, index (col)=1) -> (w2832:string[][])
                      }
                      frame True {
                        n1591 = local read "Calc: Mobility-Lin"() -> (w2843:dbl)
                        n1592 = Search 1D Array(1D array=w2840, element="Mobility-Sat (cm^2/Vs):") -> (index of element=w2848:i32)  [unwired: 1 in]
                        n1593 = Divide(x=w2848, y=3) -> (x/y=w2849:dbl)
                        n1594 = To Word Integer(number=w2849) -> (16bit integer=w2847:i16)
                        n1595 = Format Value(format string="%#g", value (0)=w2843) -> (output string=w2852:string)  [unwired: 1 in]
                        n1596 = Build Array(w2839, w2852) -> (w2845:string[])
                        n1597 = Increment(x=w2847) -> (x+1=w2846:i16)
                        n1598 = Insert Into Array(array=w2842, index (row)=w2846, new element=w2845) -> (w2841:string[][])  [unwired: 1 in]
                      }
                    }
                    n1599 = local write "Save1 Array"(w2825) -> ()
                  }
                  frame #7 {
                    w2862 = "On/Off I-Sat:"
                    n1600 = local read "Save1 Array"() -> (w2853:string[][])
                    n1601 = Array Size(array=w2853) -> (size(s)=w2859:i32[])
                    n1602 = Array Subset(array=w2853, index (row)=0, index (col)=0, length (col)=3) -> (w2855:string[][])  [unwired: 1 in]
                    n1603 = Index Array(array=w2859, index=0) -> (element=w2861:i32)
                    n1604 = Reshape Array(w2855, w2861) -> (w2854:string[])
                    n1605 = Search 1D Array(1D array=w2854, element=w2862) -> (index of element=w2865:i32)  [unwired: 1 in]
                    n1606 = Equal?(x=w2865, y=-1) -> (x = y?=w2864:bool)
                    n1607 = case shown="True" w2864 {
                      tunnel: w2853 -> [w2874 w2881]
                      tunnel: w2865 -> [w2871 _]
                      tunnel: [w2870 w2882] -> w2863
                      tunnel: w2854 -> [_ w2879]
                      tunnel: w2862 -> [_ w2877]
                      frame False {
                        n1608 = local read "Calc: On/Off"() -> (w2867:dbl)
                        n1609 = Divide(x=w2871, y=3) -> (x/y=w2873:dbl)
                        n1610 = To Word Integer(number=w2873) -> (16bit integer=w2872:i16)
                        n1611 = Format Value(format string="%#g", value (0)=w2867) -> (output string=w2868:string)  [unwired: 1 in]
                        n1612 = Replace Array Subset(array=w2874, new element=w2868, index (row)=w2872, index (col)=1) -> (w2870:string[][])
                      }
                      frame True {
                        n1613 = local read "Calc: On/Off"() -> (w2883:dbl)
                        n1614 = Search 1D Array(1D array=w2879, element="On/Off Current:") -> (index of element=w2886:i32)  [unwired: 1 in]
                        n1615 = Divide(x=w2886, y=3) -> (x/y=w2887:dbl)
                        n1616 = To Word Integer(number=w2887) -> (16bit integer=w2878:i16)
                        n1617 = Format Value(format string="%#g", value (0)=w2883) -> (output string=w2880:string)  [unwired: 1 in]
                        n1618 = Build Array(w2877, w2880) -> (w2885:string[])
                        n1619 = Replace Array Subset(array=w2881, new element=w2885, index (row)=w2878) -> (w2882:string[][])  [unwired: 1 in]
                      }
                    }
                    n1620 = local write "Save1 Array"(w2863) -> ()
                  }
                  frame #8 {
                    w2899 = "Off I-Sat (A):"
                    n1621 = local read "Save1 Array"() -> (w2890:string[][])
                    n1622 = Array Size(array=w2890) -> (size(s)=w2896:i32[])
                    n1623 = Array Subset(array=w2890, index (row)=0, index (col)=0, length (col)=3) -> (w2892:string[][])  [unwired: 1 in]
                    n1624 = Index Array(array=w2896, index=0) -> (element=w2898:i32)
                    n1625 = Reshape Array(w2892, w2898) -> (w2891:string[])
                    n1626 = Search 1D Array(1D array=w2891, element=w2899) -> (index of element=w2902:i32)  [unwired: 1 in]
                    n1627 = Equal?(x=w2902, y=-1) -> (x = y?=w2901:bool)
                    n1628 = case shown="True" w2901 {
                      tunnel: w2890 -> [w2911 w2917]
                      tunnel: w2902 -> [w2908 _]
                      tunnel: [w2907 w2916] -> w2900
                      tunnel: w2891 -> [_ w2915]
                      tunnel: w2899 -> [_ w2914]
                      frame False {
                        n1629 = local read "Calc: Off I-Sat"() -> (w2906:dbl)
                        n1630 = Divide(x=w2908, y=3) -> (x/y=w2910:dbl)
                        n1631 = Format Value(format string="%#g", value (0)=w2906) -> (output string=w2904:string)  [unwired: 1 in]
                        n1632 = To Word Integer(number=w2910) -> (16bit integer=w2909:i16)
                        n1633 = Replace Array Subset(array=w2911, new element=w2904, index (row)=w2909, index (col)=1) -> (w2907:string[][])
                      }
                      frame True {
                        n1634 = local read "Calc: Off I-Sat"() -> (w2918:dbl)
                        n1635 = Search 1D Array(1D array=w2915, element="On/Off I-Sat:") -> (index of element=w2923:i32)  [unwired: 1 in]
                        n1636 = Divide(x=w2923, y=3) -> (x/y=w2924:dbl)
                        n1637 = To Word Integer(number=w2924) -> (16bit integer=w2922:i16)
                        n1638 = Format Value(format string="%#g", value (0)=w2918) -> (output string=w2927:string)  [unwired: 1 in]
                        n1639 = Build Array(w2914, w2927) -> (w2920:string[])
                        n1640 = Increment(x=w2922) -> (x+1=w2921:i16)
                        n1641 = Insert Into Array(array=w2917, index (row)=w2921, new element=w2920) -> (w2916:string[][])  [unwired: 1 in]
                      }
                    }
                    n1642 = local write "Save1 Array"(w2900) -> ()
                  }
                  frame #9 {
                    w2929 = "Vt-Sat (V):"
                    n1643 = local read "Save1 Array"() -> (w2930:string[][])
                    n1644 = Array Size(array=w2930) -> (size(s)=w2935:i32[])
                    n1645 = Array Subset(array=w2930, index (row)=0, index (col)=0, length (col)=3) -> (w2931:string[][])  [unwired: 1 in]
                    n1646 = Index Array(array=w2935, index=0) -> (element=w2937:i32)
                    n1647 = Reshape Array(w2931, w2937) -> (w2928:string[])
                    n1648 = Search 1D Array(1D array=w2928, element=w2929) -> (index of element=w2940:i32)  [unwired: 1 in]
                    n1649 = Equal?(x=w2940, y=-1) -> (x = y?=w2939:bool)
                    n1650 = case shown="True" w2939 {
                      tunnel: w2930 -> [w2947 w2956]
                      tunnel: w2940 -> [w2943 _]
                      tunnel: [w2942 w2955] -> w2938
                      tunnel: w2929 -> [_ w2954]
                      tunnel: w2928 -> [_ w2953]
                      frame False {
                        n1651 = local read "New: VT-Sat"() -> (w2949:dbl)
                        n1652 = Number To Fractional String(number=w2949) -> (F-format string=w2944:string)  [unwired: 3 in]
                        n1653 = Divide(x=w2943, y=3) -> (x/y=w2946:dbl)
                        n1654 = To Word Integer(number=w2946) -> (16bit integer=w2945:i16)
                        n1655 = Replace Array Subset(array=w2947, new element=w2944, index (row)=w2945, index (col)=1) -> (w2942:string[][])
                      }
                      frame True {
                        n1656 = local read "New: VT-Sat"() -> (w2957:dbl)
                        n1657 = Search 1D Array(1D array=w2953, element="Threshold V (V):") -> (index of element=w2952:i32)  [unwired: 1 in]
                        n1658 = Divide(x=w2952, y=3) -> (x/y=w2960:dbl)
                        n1659 = To Word Integer(number=w2960) -> (16bit integer=w2951:i16)
                        n1660 = Format Value(format string="%#g", value (0)=w2957) -> (output string=w2963:string)  [unwired: 1 in]
                        n1661 = Build Array(w2954, w2963) -> (w2959:string[])
                        n1662 = Replace Array Subset(array=w2956, new element=w2959, index (row)=w2951) -> (w2955:string[][])  [unwired: 1 in]
                      }
                    }
                    n1663 = local write "Save1 Array"(w2938) -> ()
                  }
                  frame #10 {
                    n1664 = local read "Save1 Array"() -> (w2964:string[][])
                    n1665 = Array Size(array=w2964) -> (size(s)=w2970:i32[])
                    n1666 = Array Subset(array=w2964, index (row)=0, index (col)=0, length (col)=3) -> (w2966:string[][])  [unwired: 1 in]
                    n1667 = Index Array(array=w2970, index=0) -> (element=w2972:i32)
                    n1668 = Reshape Array(w2966, w2972) -> (w2965:string[])
                    n1669 = Search 1D Array(1D array=w2965, element="VT-Lin (V):") -> (index of element=w2975:i32)  [unwired: 1 in]
                    n1670 = Equal?(x=w2975, y=-1) -> (x = y?=w2974:bool)
                    n1671 = case shown="False" w2974 {
                      tunnel: w2964 -> [w2985 w2988]
                      tunnel: w2975 -> [w2982 _]
                      tunnel: [w2981 w2988] -> w2973
                      frame False {
                        n1672 = local read "New: VT-Lin"() -> (w2979:dbl)
                        n1673 = Divide(x=w2982, y=3) -> (x/y=w2984:dbl)
                        n1674 = Format Value(format string="%#g", value (0)=w2979) -> (output string=w2978:string)  [unwired: 1 in]
                        n1675 = To Word Integer(number=w2984) -> (16bit integer=w2983:i16)
                        n1676 = Replace Array Subset(array=w2985, new element=w2978, index (row)=w2983, index (col)=1) -> (w2981:string[][])
                      }
                      frame True {
                      }
                    }
                    n1677 = local write "Save1 Array"(w2973) -> ()
                  }
                  frame #11 {
                    w2989 = "STS-Sat (V/decade):"
                    n1678 = local read "Save1 Array"() -> (w2991:string[][])
                    n1679 = Array Size(array=w2991) -> (size(s)=w2996:i32[])
                    n1680 = Array Subset(array=w2991, index (row)=0, index (col)=0, length (col)=3) -> (w2992:string[][])  [unwired: 1 in]
                    n1681 = Index Array(array=w2996, index=0) -> (element=w2998:i32)
                    n1682 = Reshape Array(w2992, w2998) -> (w2990:string[])
                    n1683 = Search 1D Array(1D array=w2990, element=w2989) -> (index of element=w3001:i32)  [unwired: 1 in]
                    n1684 = Equal?(x=w3001, y=-1) -> (x = y?=w3000:bool)
                    n1685 = case shown="True" w3000 {
                      tunnel: w2991 -> [w3010 w3016]
                      tunnel: w3001 -> [w3007 _]
                      tunnel: [w3006 w3017] -> w2999
                      tunnel: w2990 -> [_ w3015]
                      tunnel: w2989 -> [_ w3014]
                      frame False {
                        n1686 = local read "New: STS"() -> (w3004:dbl)
                        n1687 = Divide(x=w3007, y=3) -> (x/y=w3009:dbl)
                        n1688 = Format Value(format string="%#g", value (0)=w3004) -> (output string=w3003:string)  [unwired: 1 in]
                        n1689 = To Word Integer(number=w3009) -> (16bit integer=w3008:i16)
                        n1690 = Replace Array Subset(array=w3010, new element=w3003, index (row)=w3008, index (col)=1) -> (w3006:string[][])
                      }
                      frame True {
                        n1691 = local read "New: STS"() -> (w3018:dbl)
                        n1692 = Search 1D Array(1D array=w3015, element="S.T.S. (V/decade):") -> (index of element=w3021:i32)  [unwired: 1 in]
                        n1693 = Divide(x=w3021, y=3) -> (x/y=w3022:dbl)
                        n1694 = To Word Integer(number=w3022) -> (16bit integer=w3013:i16)
                        n1695 = Format Value(format string="%#g", value (0)=w3018) -> (output string=w3025:string)  [unwired: 1 in]
                        n1696 = Build Array(w3014, w3025) -> (w3020:string[])
                        n1697 = Replace Array Subset(array=w3016, new element=w3020, index (row)=w3013) -> (w3017:string[][])  [unwired: 1 in]
                      }
                    }
                    n1698 = local write "Save1 Array"(w2999) -> ()
                  }
                  frame #12 {
                    w3026 = "Trap Density-VT (Traps/Vcm^2):"
                    n1699 = local read "Save1 Array"() -> (w3028:string[][])
                    n1700 = Array Size(array=w3028) -> (size(s)=w3033:i32[])
                    n1701 = Array Subset(array=w3028, index (row)=0, index (col)=0, length (col)=3) -> (w3029:string[][])  [unwired: 1 in]
                    n1702 = Index Array(array=w3033, index=0) -> (element=w3035:i32)
                    n1703 = Reshape Array(w3029, w3035) -> (w3027:string[])
                    n1704 = Search 1D Array(1D array=w3027, element=w3026) -> (index of element=w3038:i32)  [unwired: 1 in]
                    n1705 = Equal?(x=w3038, y=-1) -> (x = y?=w3037:bool)
                    n1706 = case shown="True" w3037 {
                      tunnel: w3028 -> [w3047 w3052]
                      tunnel: w3038 -> [w3043 _]
                      tunnel: [w3042 w3053] -> w3036
                      tunnel: w3027 -> [_ w3051]
                      tunnel: w3026 -> [_ w3050]
                      frame False {
                        n1707 = local read "New: Trap Density-VT"() -> (w3041:dbl)
                        n1708 = Format Value(format string="%#g", value (0)=w3041) -> (output string=w3044:string)  [unwired: 1 in]
                        n1709 = Divide(x=w3043, y=3) -> (x/y=w3046:dbl)
                        n1710 = To Word Integer(number=w3046) -> (16bit integer=w3045:i16)
                        n1711 = Replace Array Subset(array=w3047, new element=w3044, index (row)=w3045, index (col)=1) -> (w3042:string[][])
                      }
                      frame True {
                        n1712 = local read "New: Trap Density-VT"() -> (w3063:dbl)
                        n1713 = Search 1D Array(1D array=w3051, element="STS-Sat (V/decade):") -> (index of element=w3058:i32)  [unwired: 1 in]
                        n1714 = Divide(x=w3058, y=3) -> (x/y=w3057:dbl)
                        n1715 = To Word Integer(number=w3057) -> (16bit integer=w3059:i16)
                        n1716 = Format Value(format string="%#g", value (0)=w3063) -> (output string=w3054:string)  [unwired: 1 in]
                        n1717 = Build Array(w3050, w3054) -> (w3061:string[])
                        n1718 = Increment(x=w3059) -> (x+1=w3060:i16)
                        n1719 = Insert Into Array(array=w3052, index (row)=w3060, new element=w3061) -> (w3053:string[][])  [unwired: 1 in]
                      }
                    }
                    n1720 = local write "Save1 Array"(w3036) -> ()
                  }
                  frame #13 {
                    w3065 = "Trap Density-STS (Traps/Vcm^2):"
                    n1721 = local read "Save1 Array"() -> (w3067:string[][])
                    n1722 = Array Size(array=w3067) -> (size(s)=w3072:i32[])
                    n1723 = Array Subset(array=w3067, index (row)=0, index (col)=0, length (col)=3) -> (w3068:string[][])  [unwired: 1 in]
                    n1724 = Index Array(array=w3072, index=0) -> (element=w3074:i32)
                    n1725 = Reshape Array(w3068, w3074) -> (w3066:string[])
                    n1726 = Search 1D Array(1D array=w3066, element=w3065) -> (index of element=w3076:i32)  [unwired: 1 in]
                    n1727 = Equal?(x=w3076, y=-1) -> (x = y?=w3075:bool)
                    n1728 = case shown="True" w3075 {
                      tunnel: w3067 -> [w3085 w3090]
                      tunnel: w3076 -> [w3082 _]
                      tunnel: [w3081 w3091] -> w3064
                      tunnel: w3066 -> [_ w3089]
                      tunnel: w3065 -> [_ w3088]
                      frame False {
                        n1729 = local read "New: Trap Density-STS"() -> (w3079:dbl)
                        n1730 = Divide(x=w3082, y=3) -> (x/y=w3084:dbl)
                        n1731 = To Word Integer(number=w3084) -> (16bit integer=w3083:i16)
                        n1732 = Format Value(format string="%#g", value (0)=w3079) -> (output string=w3078:string)  [unwired: 1 in]
                        n1733 = Replace Array Subset(array=w3085, new element=w3078, index (row)=w3083, index (col)=1) -> (w3081:string[][])
                      }
                      frame True {
                        n1734 = local read "New: Trap Density-STS"() -> (w3092:dbl)
                        n1735 = Search 1D Array(1D array=w3089, element="Trap Density-VT (Traps/Vcm^2):") -> (index of element=w3097:i32)  [unwired: 1 in]
                        n1736 = Divide(x=w3097, y=3) -> (x/y=w3098:dbl)
                        n1737 = To Word Integer(number=w3098) -> (16bit integer=w3096:i16)
                        n1738 = Format Value(format string="%#g", value (0)=w3092) -> (output string=w3101:string)  [unwired: 1 in]
                        n1739 = Build Array(w3088, w3101) -> (w3094:string[])
                        n1740 = Increment(x=w3096) -> (x+1=w3095:i16)
                        n1741 = Insert Into Array(array=w3090, index (row)=w3095, new element=w3094) -> (w3091:string[][])  [unwired: 1 in]
                      }
                    }
                    n1742 = local write "Save1 Array"(w3064) -> ()
                  }
                }
                n1743 = String To Path(string=w2638) -> (path=w2621:path)
                "No Image 2" <- w2621
              }
              frame #1 {
                n1744 = Equal?(x=w3105, y=w3104) -> (x = y?=w3103:bool)
                n1745 = case shown="False" w3103 {
                  tunnel: w3105 -> [w3109 _]
                  tunnel: w3104 -> [w3108 _]
                  frame False {
                    n1746 = Move(source path=w3109, 9:TRUE, 10:w3108) -> ()  [unwired: 2 in, 3 out]
                  }
                  frame True {
                  }
                }
              }
              frame #2 {
                n1747 = local write "Transfer File"(w3111) -> ()
                n1748 = call-poly <vilib>:"Write To Spreadsheet File.vi"("2D data"=w3110, "file path (dialog if empty)"=w3111) -> ()  [unwired: 6 in, 1 out]
              }
              frame #3 {
                w3134 = 0
                w3147 = "\\"
                w3148 = "TSP"
                w3285 = 0
                # "Transpose"
                # "Moves to next file and displays new image/data"
                n1749 = property on="Image Out" class="ImageControl"() -> (error out=w3248:errorcluster, "Image Center Position"=w3252:cluster{"X":u32, "Y":u32})  [unwired: 2 in, 1 out]
                n1750 = local read "Transfer File"() -> (w3290:path)
                n1751 = Strip Path(path=w3290) -> (stripped path=w3140:path, name=w3298:string)
                n1752 = Unbundle(w3252) -> ("X"=w3250:u32)  [unwired: 1 out]
                n1753 = Strip Path(path=w3140) -> (stripped path=w3143:path)  [unwired: 1 out]
                n1754 = local write "Transfer Folder"(w3140) -> ()
                n1755 = Bundle("X"=w3250, 0) -> (w3251:cluster{"X":u32, i32})  [unwired: 1 in]
                n1756 = local read "Folder Index"() -> (w3161:dbl)
                n1757 = Path To String(path=w3143) -> (string=w3146:string)
                n1758 = property on="Image Out" class="ImageControl"(error in=w3248, "Image Center Position"=w3251) -> ()  [unwired: 1 in, 2 out]
                n1759 = List Folder(path=w3140) -> (filenames=w3295:string[])  [unwired: 3 in, 3 out]
                n1760 = Search 1D Array(1D array=w3295, element=w3298) -> (index of element=w3292:i32)  [unwired: 1 in]
                n1761 = Array Size(array=w3295) -> (size(s)=w3291:i32)
                n1762 = Decrement(x=w3291) -> (x-1=w3293:i32)
                n1763 = Equal?(x=w3292, y=w3293) -> (x = y?=w3294:bool)
                n1764 = local read "Folder Index"() -> (w3244:dbl)
                n1765 = case shown="False" w3294 {
                  tunnel: w3244 -> [w3434 _]
                  tunnel: [w3433 0] -> w3243
                  frame False {
                    n1766 = Increment(x=w3434) -> (x+1=w3433:dbl)
                  }
                  frame True {
                  }
                }
                n1767 = invoke on="Image Out" class="ImageControl" method="Clear ROI"() -> ()  [unwired: 3 in, 3 out]
                n1768 = local write "Folder Index"(w3243) -> ()
                n1769 = Path To String(path=w3140) -> (string=w3299:string)
                n1770 = Index Array(array=w3295, index=w3243) -> (element=w3139:string)
                n1771 = String Subset(string=w3139, offset (0)=3) -> (substring=w3142:string)  [unwired: 1 in]
                n1772 = Concatenate Strings(w3148, w3142) -> (w3144:string)
                n1773 = Concatenate Strings(w3146, w3147, w3148, w3147, w3144) -> (w3145:string)
                n1774 = String To Path(string=w3145) -> (path=w3138:path)
                n1775 = local write "Transport File"(w3138) -> ()
                n1776 = Strip Path(path=w3138) -> (stripped path=w3160:path, name=w3151:string)
                n1777 = local write "Transport Folder"(w3160) -> ()
                n1778 = List Folder(path=w3160) -> (filenames=w3155:string[], error out=w3163:errorcluster)  [unwired: 3 in, 2 out]
                n1779 = Array Size(array=w3155) -> (size(s)=w3159:i32)
                n1780 = Search 1D Array(1D array=w3155, element=w3151) -> (index of element=w3158:i32)  [unwired: 1 in]
                n1781 = Decrement(x=w3159) -> (x-1=w3157:i32)
                n1782 = Equal?(x=w3158, y=w3157) -> (x = y?=w3156:bool)
                n1783 = case shown="False" w3156 {
                  tunnel: w3161 -> [w3302 _]
                  tunnel: [w3301 0] -> w3162
                  tunnel: w3163 -> [w3300 w3303]
                  tunnel: [w3300 w3303] -> _
                  frame False {
                    n1784 = Increment(x=w3302) -> (x+1=w3301:dbl)
                  }
                  frame True {
                  }
                }
                n1785 = local write "Folder Index"(w3162) -> ()
                n1786 = Path To String(path=w3160) -> (string=w3150:string)
                n1787 = Index Array(array=w3155, index=w3162) -> (element=w3154:string)
                n1788 = local write "Data Name:"(w3154) -> ()
                n1789 = Concatenate Strings(w3150, "\\", w3154) -> (w3152:string)
                n1790 = String To Path(string=w3152) -> (path=w3149:path)
                n1791 = Strip Path(path=w3149) -> ()  [unwired: 2 out]
                n1792 = call-poly <vilib>:"Read From Spreadsheet File.vi"("file path (dialog if empty)"=w3149) -> ("all rows"=w3177:string[][])  [unwired: 6 in, 4 out]
                n1793 = Array Size(array=w3177) -> (size(s)=w3183:i32[])
                n1794 = Array Subset(array=w3177, length (col)=1) -> (w3179:string[][])  [unwired: 3 in]
                n1795 = Index Array(array=w3183, index=0) -> (element=w3172:i32)
                n1796 = Reshape Array(w3179, w3172) -> (w3178:string[])
                n1797 = Search 1D Array(1D array=w3178, element="Vd") -> (index of element=w3176:i32)  [unwired: 1 in]
                n1798 = Increment(x=w3176) -> (x+1=w3175:i32)
                n1799 = Array Subset(array=w3177, index (row)=w3175) -> (w3173:string[][])  [unwired: 3 in]
                n1800 = local write "Data Name:"(w3139) -> ()
                n1801 = Fract/Exp String To Number(string=w3173, default (0 dbl)="default (0 dbl) 4") -> (number=w3165:ext[][])  [unwired: 2 in, 1 out]
                n1802 = Delete From Array(array=w3165) -> (array with subset deleted=w3164:ext[][])  [unwired: 3 in, 1 out]
                n1803 = Concatenate Strings(w3299, "\\", w3139) -> (w3297:string)
                n1804 = Delete From Array(array=w3164, index (col)=0 ("Deaktivierter Index (Spalte)")) -> (deleted portion=w3169:ext[], array with subset deleted=w3170:ext[][])  [unwired: 2 in]
                n1805 = String To Path(string=w3297) -> (path=w3112:path)
                n1806 = call "Recorded Values.vi"("Path"=w3112) -> ("Recorded Char"=w3199:T6, "Recorded Prop"=w3200:T7, "Fabrication Prop"=w3198:T8)  [unwired: 8 in]
                n1807 = Unbundle By Name(w3199) -> ("Mobility-Sat"=w3212:dbl, "Moblitity-Lin"=w3213:dbl, "On/Off"=w3214:dbl, "Off Current"=w3215:dbl, "Vt-Sat"=w3192:dbl, "STS"=w3216:dbl, "Trap Density-VT"=w3217:dbl, "Trap Density-STS"=w3218:dbl)
                n1808 = Unbundle By Name(w3200) -> ("Date Recorded"=w3208:string, "Index"=w3209:string, "Length"=w3210:dbl, "Width"=w3211:dbl, "Sample Temp"=w3195:dbl)
                n1809 = Unbundle By Name(w3198) -> ("Date Created"=w3219:string, "Material"=w3201:string, "Solvent"=w3202:string, "Concentration"=w3203:dbl, "Method"=w3204:string, "Dielectric (nm)"=w3205:dbl, "Treatment"=w3206:string, "Comments"=w3207:string)
                n1810 = local write "Rec: Off I-Sat"(w3215) -> ()
                n1811 = local write "Rec: Comments"(w3207) -> ()
                n1812 = local write "Rec: VT-Sat"(w3192) -> ()
                n1813 = local write "Date Created"(w3219) -> ()
                n1814 = local write "Rec: Material"(w3201) -> ()
                n1815 = local write "Rec: Solvent"(w3202) -> ()
                n1816 = local write "Rec: Concentration"(w3203) -> ()
                n1817 = local write "Rec: Method"(w3204) -> ()
                n1818 = local write "Rec: Dielectric (d)"(w3205) -> ()
                n1819 = local write "Surface Treatment:"(w3206) -> ()
                n1820 = local write "Index"(w3209) -> ()
                n1821 = local write "Rec: Mobility-Sat"(w3212) -> ()
                n1822 = local write "Rec: Mobility-Lin"(w3213) -> ()
                n1823 = local write "Rec: On/Off"(w3214) -> ()
                n1824 = local write "Rec: STS"(w3216) -> ()
                n1825 = local write "Rec: Trap Density-VT"(w3217) -> ()
                n1826 = local write "Rec: Trap Density-STS"(w3218) -> ()
                n1827 = local write "Date Recorded"(w3208) -> ()
                n1828 = local write "Rec: Length"(w3210) -> ()
                n1829 = local write "Rec: Width"(w3211) -> ()
                n1830 = local write "Rec: Temp"(w3195) -> ()
                n1831 = Equal To 0?(x=w3195) -> (x = 0?=w3196:bool)
                n1832 = case shown="False" w3196 {
                  tunnel: [w3311 w3312] -> w3193
                  tunnel: w3195 -> [w3311 _]
                  frame False {
                  }
                  frame True {
                    n1833 = local read "Room Temp"() -> (w3312:dbl)
                  }
                }
                n1834 = local read "NumPoints Log"() -> (w3240:dbl)
                n1835 = Transpose 2D Array(2D array=w3170) -> (transposed array=w3171:ext[][])
                n1836 = local write "Transfer File"(w3112) -> ()
                n1837 = local read "Num Pts"() -> (w3229:dbl)
                n1838 = local read "Num Pts"() -> (w3241:dbl)
                n1839 = for {
                  tunnel: w3169 -> [w3309]
                  tunnel: w3171 -> [w3310] mode=indexing
                  tunnel: [w3308] -> w3167 mode=indexing
                  n1840 = Bundle(w3309, w3310) -> (w3308:cluster{ext[], ext[]})  [unwired: 1 in]
                }
                n1841 = call-poly <vilib>:"Read From Spreadsheet File.vi"("file path (dialog if empty)"=w3112) -> ("all rows"=w3287:string[][])  [unwired: 6 in, 4 out]
                n1842 = call "Mobility-Vt Calculator-File.vi"("NumPts"=w3241, "Path"=w3112) -> ("Graph Cluster"=w3189:T9, "Output"=w3242:T10, "Index-Sat"=w3222:dbl, "Index-Lin"=w3228:dbl)  [unwired: 5 in, 1 out]
                n1843 = Unbundle By Name(w3189) -> ("Raw Sat"=w3186:cluster{dbl[], dbl[]}[], "Sqrt Sat"=w3188:cluster{dbl[], dbl[]}[], "Raw Lin"=w3185:cluster{dbl[], dbl[]}[], "Sqrt Lin"=w3187:cluster{dbl[], dbl[]}[], "Log Lin"=w3184:cluster{dbl[], dbl[]}[])  [unwired: 1 out]
                n1844 = Decimate 1D Array(w3187) -> (w3236:cluster{dbl[], dbl[]}[])  [unwired: 1 out]
                n1845 = Array To Cluster(array=w3236) -> (cluster=w3234:T11)
                n1846 = Unbundle(w3234) -> ("[0]"=w3235:cluster{dbl[], dbl[]})  [unwired: 8 out]
                n1847 = Unbundle(w3235) -> (w3233:dbl[], w3232:dbl[])
                n1848 = Array Subset(array=w3232, index=w3228, length=w3229) -> (w3230:dbl[])
                n1849 = Array Subset(array=w3233, index=w3228, length=w3229) -> (w3231:dbl[])
                n1850 = call "STS Calculator-File.vi"("NumPts"=w3240, "Path"=w3112) -> ("STS Index-Sat"=w3239:dbl, "XY Graph-Sat"=w3238:cluster{dbl[], dbl[]}[], "Ouput"=w3237:cluster{"STS-Sat":dbl, "STS-Lin":dbl})  [unwired: 5 in, 2 out]
                n1851 = local write "Transport"(w3167) -> ()
                n1852 = Array Size(array=w3167) -> (size(s)=w3166:i32)
                n1853 = local read "New: Dielectric"() -> (w3224:dbl)
                n1854 = local write "Sat-Trans Slider"(w3222) -> ()
                n1855 = for {
                  N: w3166 -> [_]
                  i -> [w3307]
                  n1856 = local read "Transport Line Color"() -> (w3306:u32)
                  n1857 = local read "Ring"() -> (w3305:u16)
                  n1858 = property on="Transport" class="XYGraph (strict)"("Active Plot"=w3307, "Plot.Plot Color"=w3306, "Plot.Line Width"=w3305) -> ()  [unwired: 2 in, 2 out]
                }
                n1859 = local write "Lin Id-Used"(w3230) -> ()
                n1860 = local write "Lin-Vg Array-Used"(w3231) -> ()
                n1861 = local write "MobVi Index"(w3222) -> ()
                n1862 = local write "Index 2"(w3239) -> ()
                n1863 = local write "Sqrt-Sat"(w3188) -> ()
                n1864 = local write "Sat-Log"(w3238) -> ()
                n1865 = Unbundle By Name(w3242) -> ("Mobility-Sat"=w3227:dbl, "Vt-Sat"=w3190:dbl, "Mobility-Lin"=w3226:dbl, "Mobility-Lin"=w3225:dbl, "Off I-Sat"=w3220:dbl, "On/Off I-Sat"=w3191:dbl)
                n1866 = local write "Sqrt-Lin"(w3187) -> ()
                n1867 = Array Size(array=w3287) -> (size(s)=w3286:i32[])
                n1868 = local write "Raw- Sat"(w3186) -> ()
                n1869 = local write "New: Temp"(w3193) -> ()
                n1870 = Unbundle By Name(w3237) -> ("STS-Sat"=w3223:dbl)
                n1871 = call "Trap Density_STS.vi"("Temp (T) [K]"=w3193, "S.T.S. (S)"=w3223, "Dielectric"=w3224) -> ("Trap Density (N)"=w3197:dbl)  [unwired: 8 in]
                n1872 = local write "Calc: Mobility-Lin"(w3226) -> ()
                n1873 = local write "Raw- Lin"(w3185) -> ()
                n1874 = local write "Calc: Mobility-Sat"(w3227) -> ()
                n1875 = local write "Log-Lin"(w3184) -> ()
                n1876 = local write "Calc: Off I-Sat"(w3220) -> ()
                n1877 = local write "Calc: VT-Sat"(w3190) -> ()
                n1878 = local write "New: VT-Lin"(w3225) -> ()
                n1879 = local write "New: Trap Density-STS"(w3197) -> ()
                n1880 = local write "Calc: Trap Density-STS"(w3197) -> ()
                n1881 = local read "Image Folder"() -> (w3276:path)
                n1882 = local read "New: Dielectric"() -> (w3221:dbl)
                n1883 = Decimate 1D Array(w3188) -> (w3271:cluster{dbl[], dbl[]}[])  [unwired: 1 out]
                n1884 = Decimate 1D Array(w3238) -> (w3261:cluster{dbl[], dbl[]}[])  [unwired: 1 out]
                n1885 = Index Array(array=w3286, index=w3285) -> (element=w3267:i32)
                n1886 = Array Subset(array=w3287, index (row)=w3285, index (col)=w3285, length (col)=3) -> (w3288:string[][])  [unwired: 1 in]
                n1887 = local write "Calc: STS"(w3223) -> ()
                n1888 = local write "New: VT-Sat"(w3190) -> ()
                n1889 = local write "New: Mobility-Sat"(w3227) -> ()
                n1890 = local write "Calc: On/Off"(w3191) -> ()
                n1891 = local write "New: Mobility-Lin"(w3226) -> ()
                n1892 = List Folder(path=w3276) -> (filenames=w3281:string[])  [unwired: 3 in, 3 out]
                n1893 = local write "New: VT-Lin"(w3225) -> ()
                n1894 = Array To Cluster(array=w3271) -> (cluster=w3273:T11)
                n1895 = Array To Cluster(array=w3261) -> (cluster=w3259:T11)
                n1896 = Reshape Array(w3288, w3267) -> (w3274:string[])
                n1897 = Subtract(x=w3267, y=20) -> (x-y=w3266:i32)
                n1898 = local write "New: STS"(w3223) -> ()
                n1899 = property on="Sat-Trans Slider" class="Slide (strict)"("Scale.Maximum"=w3266) -> ()  [unwired: 2 in, 2 out]
                n1900 = call "Trap Density_VT.vi"("VT"=w3190, "Dielectric"=w3221) -> ("Trap Density-VT"=w3194:dbl)
                n1901 = Unbundle(w3273) -> ("[0]"=w3272:cluster{dbl[], dbl[]})  [unwired: 8 out]
                n1902 = Unbundle(w3259) -> ("[0]"=w3260:cluster{dbl[], dbl[]})  [unwired: 8 out]
                n1903 = Search 1D Array(1D array=w3274, element="Index:") -> (index of element=w3282:i32)  [unwired: 1 in]
                n1904 = local write "New: Trap Density-VT"(w3194) -> ()
                n1905 = local write "Calc: Trap Density-VT"(w3194) -> ()
                n1906 = call-poly <vilib>:"Read From Spreadsheet File.vi"("file path (dialog if empty)"=w3112) -> ("all rows"=w3116:string[][])  [unwired: 6 in, 4 out]
                n1907 = Unbundle(w3272) -> (w3263:dbl[], w3262:dbl[])
                n1908 = Unbundle(w3260) -> (w3258:dbl[], w3257:dbl[])
                n1909 = Increment(x=w3282) -> (x+1=w3283:i32)
                n1910 = Array Size(array=w3116) -> (size(s)=w3135:i32[])
                n1911 = Array Subset(array=w3263, index=w3222, length=w3241) -> (w3270:dbl[])
                n1912 = Array Subset(array=w3262, index=w3222, length=w3241) -> (w3269:dbl[])
                n1913 = Array Subset(array=w3258, index=w3239, length=w3240) -> (w3265:dbl[])
                n1914 = Array Subset(array=w3257, index=w3239, length=w3240) -> (w3264:dbl[])
                n1915 = Index Array(array=w3274, index=w3283) -> (element=w3279:string)
                n1916 = local write "Vg Array-Log-Used"(w3264) -> ()
                n1917 = local write "Sat Id-Log-Used"(w3265) -> ()
                n1918 = local write "Sat Id-Used"(w3269) -> ()
                n1919 = local write "Index"(w3279) -> ()
                n1920 = Index Array(array=w3135, index=0) -> (element=w3133:i32)
                n1921 = local write "Sat Vg Array-Used"(w3270) -> ()
                n1922 = while {
                  tunnel: w3281 -> [w3320]
                  tunnel: w3279 -> [w3318]
                  tunnel: [w3317] -> _
                  tunnel: [w3317] -> w3280
                  tunnel: w3267 -> [w3316]
                  i -> [w3317]
                  stop <- w3313 stop-if-true
                  n1923 = Index Array(array=w3320, index=w3317) -> (element=w3321:string)
                  n1924 = xnode "Match Regular Expression"("input string"=w3321, "regular expression"=w3318) -> ("whole match"=w3319:string)  [unwired: 4 in, 4 out]
                  n1925 = Equal?(x=w3319, y=w3318) -> (x = y?=w3315:bool)
                  n1926 = Equal?(x=w3316, y=w3317) -> (x = y?=w3314:bool)
                  n1927 = Or(x=w3315, y=w3314) -> (x .or. y?=w3313:bool)
                }
                n1928 = Array Subset(array=w3116, index (row)=w3134, index (col)=w3134, length (col)=3) -> (w3136:string[][])  [unwired: 1 in]
                n1929 = Reshape Array(w3136, w3133) -> (w3118:string[])
                n1930 = Search 1D Array(1D array=w3118, element="Vg") -> (index of element=w3122:i32)  [unwired: 1 in]
                n1931 = Add(x=w3122, y=3) -> (x+y=w3120:i32)
                n1932 = Divide(x=w3120, y=3) -> (x/y=w3127:dbl)
                n1933 = Array Subset(array=w3116, index (row)=w3127, index (col)=0, length (col)=1) -> (w3126:string[][])  [unwired: 1 in]
                n1934 = Fract/Exp String To Number(string=w3126) -> (number=w3130:dbl[][])  [unwired: 3 in, 1 out]
                n1935 = Array Size(array=w3130) -> (size(s)=w3117:i32[])
                n1936 = Index Array(array=w3117, index=0) -> (element=w3128:i32)
                n1937 = Decrement(x=w3128) -> (x-1=w3131:i32)
                n1938 = Reshape Array(w3130, w3131) -> (w3115:dbl[])
                n1939 = local write "Data Length"(w3131) -> ()
                n1940 = local write "Vg Column"(w3115) -> ()
                n1941 = Array Max & Min(array=w3115) -> (max value=w3114:dbl, min value=w3113:dbl)  [unwired: 2 out]
                n1942 = Path To String(path=w3276) -> (string=w3278:string)
                n1943 = Index Array(array=w3281, index=w3280) -> (element=w3255:string)
                n1944 = local write "Image Name"(w3255) -> ()
                n1945 = property on="Sat-Trans Slider" class="Slide (strict)"("Scale.Maximum"=w3114, "Scale.Minimum"=w3113) -> ()  [unwired: 2 in, 2 out]
                n1946 = Empty String/Path?(string/path=w3255) -> (empty?=w3256:bool)
                n1947 = Concatenate Strings(w3278, "\\", w3255) -> (w3277:string)
                n1948 = String To Path(string=w3277) -> (path=w3254:path)
                n1949 = local read "No Image File"() -> (w3253:path)
                n1950 = Select(t=w3253, s=w3256, f=w3254) -> (s? t:f=w3247:path)
                n1951 = local write "Image File"(w3247) -> ()
                n1952 = local read "Image Out"() -> (w3245:T2)
                n1953 = call "IMAQ ReadFile"("File Path"=w3247, "Image"=w3245) -> ("Image Out"=w3246:T2)  [unwired: 5 in, 4 out]
                n1954 = local write "Image Out"(w3246) -> ()
                n1955 = local write "Image Out 2"(w3246) -> ()
              }
              frame #4 {
                # "Output ROI data"
                n1956 = local read "Image Folder"() -> (w3436:path)
                n1957 = Build Path(base path=w3436, name or relative path="ROI") -> (appended path=w3438:path)
                n1958 = local read "Index"() -> (w3437:string)
                n1959 = Build Path(base path=w3438, name or relative path=w3437) -> (appended path=w3443:path)
                n1960 = invoke on="Image Out" class="ImageControl" method="Clear ROI"() -> (error out=w3442:errorcluster)  [unwired: 3 in, 2 out]
                n1961 = call <vilib>:"Check if File or Folder Exists.vi"("error in (no error)"=w3442, "path"=w3443) -> ("file or folder exists?"=w3440:bool, "dup path"=w3441:path)  [unwired: 7 in, 1 out]
                n1962 = case shown="True" w3440 {
                  tunnel: w3441 -> [_ w3444]
                  frame False {
                  }
                  frame True {
                    n1963 = Read from Text File(file (use dialog)=w3444) -> (text=w3448:string)  [unwired: 3 in, 3 out]
                    n1964 = property on="Image Out" class="ImageControl"() -> ("ROI"=w3445:T12)  [unwired: 2 in, 2 out]
                    n1965 = Unflatten From String(type=w3445, binary string=w3448) -> (value=w3446:T12, error out=w3447:errorcluster)  [unwired: 3 in, 1 out]
                    n1966 = property on="Image Out" class="ImageControl"(error in=w3447, "ROI"=w3446) -> ()  [unwired: 1 in, 2 out]
                  }
                }
              }
            }
            n1967 = flat-sequence {
              tunnel: [w2578] -> w2565
              tunnel: w2565 -> [w2592]
              frame #0 {
                # "Makes Empty File for Transformer Data"
                n1968 = local read "Transfer Folder"() -> (w2567:path)
                n1969 = Build Path(base path=w2567, name or relative path="Stats") -> (appended path=w2569:path)
                n1970 = call <vilib>:"Check if File or Folder Exists.vi"("path"=w2569) -> ("file or folder exists?"=w2570:bool, "dup path"=w2571:path)  [unwired: 8 in, 1 out]
                n1971 = case shown="False" w2570 {
                  tunnel: [w2575 w2577] -> w2572
                  tunnel: w2571 -> [w2576 w2577]
                  frame False {
                    n1972 = Create Folder(path (use dialog)=w2576) -> (created path=w2575:path)  [unwired: 2 in, 2 out]
                  }
                  frame True {
                  }
                }
                n1973 = Build Path(base path=w2572, name or relative path="Tranformer Data.txt") -> (appended path=w2574:path)
                n1974 = call-poly <vilib>:"Write To Spreadsheet File.vi"("append to file? (new file:F)"=TRUE, "file path (dialog if empty)"=w2574) -> ()  [unwired: 6 in, 1 out]
              }
              frame #1 {
                # "Adds Headers if they don't exist"
                n1975 = local read "Transfer Folder"() -> (w2584:path)
                n1976 = Concatenate Strings("Stats\\", "Tranformer Data.txt") -> (w2585:string)
                n1977 = Build Path(base path=w2584, name or relative path=w2585) -> (appended path=w2578:path)
                n1978 = call-poly <vilib>:"Read From Spreadsheet File.vi"("file path (dialog if empty)"=w2578) -> ("first row"=w2583:string[])  [unwired: 6 in, 4 out]
                n1979 = Search 1D Array(1D array=w2583, element="DeviceID") -> (index of element=w2581:i32)  [unwired: 1 in]
                n1980 = Equal?(x=w2581, y=0) -> (x = y?=w2579:bool)
                n1981 = case shown="False" w2579 {
                  tunnel: w2578 -> [w2589 _]
                  frame False {
                    n1982 = local read "Transformer \nHeaders"() -> (w2588:string[])
                    n1983 = call-poly <vilib>:"Write To Spreadsheet File.vi"("1D data"=w2588, "file path (dialog if empty)"=w2589) -> ()  [unwired: 6 in, 1 out]
                  }
                  frame True {
                  }
                }
              }
              frame #2 {
                # "Adds current device if it doesn't exist"
                n1984 = local read "Current \nRecord"() -> (w2595:string[])
                n1985 = Index Array(array=w2595, index=0) -> (element=w2594:string)
                n1986 = local read "Transfer Folder"() -> (w2597:path)
                n1987 = Concatenate Strings("Stats\\", "Tranformer Data.txt") -> (w2598:string)
                n1988 = local write "Current Device ID"(w2594) -> ()
                n1989 = local read "Current Device ID"() -> (w2604:string)
                n1990 = Build Path(base path=w2597, name or relative path=w2598) -> (appended path=w2596:path)
                n1991 = call-poly <vilib>:"Read From Spreadsheet File.vi"("file path (dialog if empty)"=w2596) -> ("all rows"=w2591:string[][])  [unwired: 6 in, 4 out]
                n1992 = Index Array(array=w2591, index (col)=0) -> (element=w2602:string[])  [unwired: 1 in]
                n1993 = Search 1D Array(1D array=w2602, element=w2604) -> (index of element=w2590:i32)  [unwired: 1 in]
                n1994 = Equal?(x=w2590, y=-1) -> (x = y?=w2593:bool)
                n1995 = case shown="False" w2593 {
                  tunnel: w2592 -> [w2606 w2619]
                  tunnel: w2590 -> [w2611 _]
                  tunnel: w2591 -> [w2612 _]
                  frame False {
                    n1996 = local read "Current \nRecord"() -> (w2610:string[])
                    n1997 = Replace Array Subset(array=w2612, new element=w2610, index (row)=w2611) -> (w2607:string[][])  [unwired: 1 in]
                    n1998 = flat-sequence {
                      tunnel: [w2613] -> _
                      tunnel: [w2614] -> _
                      tunnel: [w2614] -> w2609
                      tunnel: [w2613] -> w2608
                      tunnel: w2607 -> [w2614]
                      tunnel: w2606 -> [w2613]
                      tunnel: w2609 -> [w2616]
                      tunnel: w2608 -> [w2615]
                      frame #0 {
                        n1999 = Delete(path (use dialog)=w2613) -> ()  [unwired: 4 in, 3 out]
                      }
                      frame #1 {
                        n2000 = call-poly <vilib>:"Write To Spreadsheet File.vi"("append to file? (new file:F)"=TRUE, "2D data"=w2616, "file path (dialog if empty)"=w2615) -> ()  [unwired: 5 in, 1 out]
                      }
                    }
                  }
                  frame True {
                    n2001 = local read "Current \nRecord"() -> (w2618:string[])
                    n2002 = call-poly <vilib>:"Write To Spreadsheet File.vi"("append to file? (new file:F)"=TRUE, "1D data"=w2618, "file path (dialog if empty)"=w2619) -> ()  [unwired: 5 in, 1 out]
                  }
                }
              }
            }
          }
          event "Export": Mouse Down {
            n2003 = event-data() -> ()  [unwired: 1 in, 7 out]
            n2004 = flat-sequence {
              frame #0 {
                n2005 = stacked-sequence {
                  frame #0 {
                    n2006 = local read "Independant Variable"() -> (w3450:string)
                    n2007 = Equal?(x=w3450, y="Length (um):") -> (x = y?=w3451:bool)
                    n2008 = case shown="True" w3451 {
                      frame False {
                      }
                      frame True {
                        n2009 = local write "X Axis Display Type"("1") -> ()
                        n2010 = local write "Opj X Axis"("2") -> ()
                      }
                    }
                  }
                  frame #1 {
                    n2011 = local read "Independant Variable"() -> (w3455:string)
                    n2012 = Equal?(x=w3455, y="Sample Temp (K):") -> (x = y?=w3456:bool)
                    n2013 = case shown="True" w3456 {
                      frame False {
                      }
                      frame True {
                        n2014 = local write "X Axis Display Type"("1") -> ()
                        n2015 = local write "Opj X Axis"("1") -> ()
                      }
                    }
                  }
                  frame #2 {
                    n2016 = local read "Independant Variable"() -> (w3460:string)
                    n2017 = Equal?(x=w3460, y="Mobility-Sat (cm^2/Vs):") -> (x = y?=w3461:bool)
                    n2018 = case shown="True" w3461 {
                      frame False {
                      }
                      frame True {
                        n2019 = local write "X Axis Display Type"("2") -> ()
                        n2020 = local write "Opj X Axis"("2") -> ()
                      }
                    }
                  }
                  frame #3 {
                    n2021 = local read "Independant Variable"() -> (w3465:string)
                    n2022 = Equal?(x=w3465, y="Mobility-Lin (cm^2/Vs):") -> (x = y?=w3466:bool)
                    n2023 = case shown="True" w3466 {
                      frame False {
                      }
                      frame True {
                        n2024 = local write "X Axis Display Type"("2") -> ()
                        n2025 = local write "Opj X Axis"("2") -> ()
                      }
                    }
                  }
                  frame #4 {
                    n2026 = local read "Independant Variable"() -> (w3470:string)
                    n2027 = Equal?(x=w3470, y="On/Off I-Sat:") -> (x = y?=w3471:bool)
                    n2028 = case shown="True" w3471 {
                      frame False {
                      }
                      frame True {
                        n2029 = local write "X Axis Display Type"("2") -> ()
                        n2030 = local write "Opj X Axis"("2") -> ()
                      }
                    }
                  }
                  frame #5 {
                    n2031 = local read "Independant Variable"() -> (w3475:string)
                    n2032 = Equal?(x=w3475, y="Off I-Sat (A):") -> (x = y?=w3476:bool)
                    n2033 = case shown="True" w3476 {
                      frame False {
                      }
                      frame True {
                        n2034 = local write "X Axis Display Type"("2") -> ()
                        n2035 = local write "Opj X Axis"("2") -> ()
                      }
                    }
                  }
                  frame #6 {
                    n2036 = local read "Independant Variable"() -> (w3480:string)
                    n2037 = Equal?(x=w3480, y="Vt-Sat (V):") -> (x = y?=w3481:bool)
                    n2038 = case shown="True" w3481 {
                      frame False {
                      }
                      frame True {
                        n2039 = local write "X Axis Display Type"("1") -> ()
                        n2040 = local write "Opj X Axis"("1") -> ()
                      }
                    }
                  }
                  frame #7 {
                    n2041 = local read "Independant Variable"() -> (w3485:string)
                    n2042 = Equal?(x=w3485, y="STS-Sat (V/decade):") -> (x = y?=w3486:bool)
                    n2043 = case shown="True" w3486 {
                      frame False {
                      }
                      frame True {
                        n2044 = local write "X Axis Display Type"("1") -> ()
                        n2045 = local write "Opj X Axis"("1") -> ()
                      }
                    }
                  }
                  frame #8 {
                    n2046 = local read "Independant Variable"() -> (w3490:string)
                    n2047 = Equal?(x=w3490, y="Trap Density-VT (Traps/Vcm^2):") -> (x = y?=w3491:bool)
                    n2048 = case shown="True" w3491 {
                      frame False {
                      }
                      frame True {
                        n2049 = local write "X Axis Display Type"("2") -> ()
                        n2050 = local write "Opj X Axis"("2") -> ()
                      }
                    }
                  }
                  frame #9 {
                    n2051 = local read "Independant Variable"() -> (w3495:string)
                    n2052 = Equal?(x=w3495, y="Trap Density-STS (Traps/Vcm^2):") -> (x = y?=w3496:bool)
                    n2053 = case shown="True" w3496 {
                      frame False {
                      }
                      frame True {
                        n2054 = local write "X Axis Display Type"("2") -> ()
                        n2055 = local write "Opj X Axis"("2") -> ()
                      }
                    }
                  }
                }
              }
              frame #1 {
                n2056 = local read "Transfer Folder"() -> (w3504:path)
                n2057 = Build Path(base path=w3504, name or relative path="Stats") -> (appended path=w3505:path)
                n2058 = local read "Origin Project File"() -> (w3516:path)
                n2059 = call <vilib>:"Check if File or Folder Exists.vi"("path"=w3505) -> ("file or folder exists?"=w3520:bool, "dup path"=w3519:path)  [unwired: 8 in, 1 out]
                n2060 = call <userlib>:"OA_ConnectToOrigin.vi"() -> ("error out"=w3517:errorcluster, "Origin.IOApplication"=w3518:refnum<k7>)  [unwired: 8 in]
                n2061 = case shown="False" w3520 {
                  tunnel: w3519 -> [w3693 w3694]
                  tunnel: [w3692 w3694] -> w3503
                  frame False {
                    n2062 = Create Folder(path (use dialog)=w3693) -> (created path=w3692:path)  [unwired: 2 in, 2 out]
                  }
                  frame True {
                  }
                }
                n2063 = call <userlib>:"OA_Load.vi"("error in (no error)"=w3517, "Path"=w3516, "Origin.IOApplication"=w3518) -> ("error out"=w3514:errorcluster, "Origin.IOApplication"=w3515:refnum<k7>)  [unwired: 1 out]
                n2064 = call "OAExecute.vi"("script"="document -m 3;", "Error IO"=w3514, "Origin.IOApplication"=w3515) -> ("Error IO Out"=w3512:errorcluster, "Origin.IOApplication"=w3513:refnum<k7>)  [unwired: 1 in, 1 out]
                n2065 = call "File Dialog"("start path"=w3505) -> ("selected path"=w3507:path)  [unwired: 11 in, 3 out]
                n2066 = local read "Independant Variable"() -> (w3500:string)
                n2067 = stacked-sequence {
                  tunnel: w3504 -> [w3531 w3561 w3573 w3595 w3615 w3636 w3657 w3680]
                  tunnel: w3503 -> [w3532 w3560 w3574 w3594 w3616 w3637 w3658 w3681]
                  tunnel: w3513 -> [w3534 w3558 w3576 w3597 w3618 w3639 w3660 w3683]
                  tunnel: w3512 -> [w3533 w3559 w3575 w3596 w3617 w3638 w3659 w3682]
                  tunnel: [_ _ _ _ _ _ _ w3678] -> w3502
                  tunnel: [_ _ _ _ _ _ _ w3679] -> w3501
                  tunnel: w3500 -> [w3530 w3551 w3572 w3593 w3614 w3635 w3656 w3677]
                  frame #0 {
                    n2068 = local read "X Axis Display Type"() -> (w3522:string)
                    n2069 = local read "Opj X Axis"() -> (w3527:string)
                    n2070 = Concatenate Strings("window -a MOBLGraph;\nlayer.x.type=", w3527, "; layer.x.label.numFormat = ", w3522, "; Y3 = 1; X3 = 1;", "window -a MOBLTable;\nwindow -s TV;") -> (w3525:string)
                    n2071 = call "Param_Analysis_7_24b_JW.vi"("Independant Variable"=w3530, "error in (no error)"=w3533, "Data Folder"=w3531, "Parameter String"="Mobility-Lin (cm^2/Vs):", "Parameter Name"="Mobility-Lin", "Stats Folder"=w3532) -> ("error out"=w3536:errorcluster, "Output Array"=w3538:string[][], "Variables"=w3529:T18)  [unwired: 2 in, 1 out]
                    n2072 = call "Origin_Export_7_27a_JW.vi"("Input Conditions"=w3529, "Analysis Array"=w3538, "error in (no error)"=w3536, "Parameter Worksheet Name"="[MOBLTable]Mobilities", "Parameter Folder Script"="pe_cd \"Mobility-Lin\";", "Origin.IOApplication"=w3534) -> ("error out"=w3535:errorcluster, "reference out"=w3537:refnum<k7>)  [unwired: 3 in, 1 out]
                    n2073 = call "OAExecute.vi"("script"=w3525, "Error IO"=w3535, "Origin.IOApplication"=w3537) -> ()  [unwired: 1 in, 3 out]
                  }
                  frame #1 {
                    n2074 = local read "X Axis Display Type"() -> (w3543:string)
                    n2075 = local read "Opj X Axis"() -> (w3548:string)
                    n2076 = Concatenate Strings("window -a MOBSGraph;\nlayer.x.type=", w3548, "; layer.x.label.numFormat = ", w3543, "; Y3 = 1; X3 = 1;", "window -a MOBSTable;\nwindow -s TV;") -> (w3546:string)
                    n2077 = call "Param_Analysis_7_24b_JW.vi"("Independant Variable"=w3551, "error in (no error)"=w3559, "Data Folder"=w3561, "Parameter String"="Mobility-Sat (cm^2/Vs):", "Parameter Name"="Mobility-Sat", "Stats Folder"=w3560) -> ("error out"=w3554:errorcluster, "Output Array"=w3552:string[][], "Variables"=w3550:T18)  [unwired: 2 in, 1 out]
                    n2078 = call "Origin_Export_7_27a_JW.vi"("Input Conditions"=w3550, "Analysis Array"=w3552, "error in (no error)"=w3554, "Parameter Worksheet Name"="[MOBSTable]Mobilities", "Parameter Folder Script"="pe_cd \"Mobility-Sat\";", "Origin.IOApplication"=w3558) -> ("error out"=w3553:errorcluster, "reference out"=w3555:refnum<k7>)  [unwired: 3 in, 1 out]
                    n2079 = call "OAExecute.vi"("script"=w3546, "Error IO"=w3553, "Origin.IOApplication"=w3555) -> ()  [unwired: 1 in, 3 out]
                  }
                  frame #2 {
                    n2080 = local read "X Axis Display Type"() -> (w3564:string)
                    n2081 = local read "Opj X Axis"() -> (w3569:string)
                    n2082 = Concatenate Strings("window -a NSTSGraph;\nlayer.x.type=", w3569, "; layer.x.label.numFormat = ", w3564, "; Y3 = 1; X3 = 1;", "window -a NSTSTable;\nwindow -s TV;") -> (w3567:string)
                    n2083 = call "Param_Analysis_7_24b_JW.vi"("Independant Variable"=w3572, "error in (no error)"=w3575, "Data Folder"=w3573, "Parameter String"="Trap Density-STS (Traps/Vcm^2):", "Parameter Name"="Trap Density-STS", "Stats Folder"=w3574) -> ("error out"=w3579:errorcluster, "Output Array"=w3577:string[][], "Variables"=w3571:T18)  [unwired: 2 in, 1 out]
                    n2084 = call "Origin_Export_7_27a_JW.vi"("Input Conditions"=w3571, "Analysis Array"=w3577, "error in (no error)"=w3579, "Parameter Worksheet Name"="[NSTSTable]Trap Densities", "Parameter Folder Script"="pe_cd \"N-STS\";", "Origin.IOApplication"=w3576) -> ("error out"=w3578:errorcluster, "reference out"=w3580:refnum<k7>)  [unwired: 3 in, 1 out]
                    n2085 = call "OAExecute.vi"("script"=w3567, "Error IO"=w3578, "Origin.IOApplication"=w3580) -> ()  [unwired: 1 in, 3 out]
                  }
                  frame #3 {
                    n2086 = local read "X Axis Display Type"() -> (w3585:string)
                    n2087 = local read "Opj X Axis"() -> (w3590:string)
                    n2088 = call "Param_Analysis_7_24b_JW.vi"("Independant Variable"=w3593, "error in (no error)"=w3596, "Data Folder"=w3595, "Parameter String"="Trap Density-VT (Traps/Vcm^2):", "Parameter Name"="Trap Density-Vt", "Stats Folder"=w3594) -> ("error out"=w3600:errorcluster, "Output Array"=w3598:string[][], "Variables"=w3592:T18)  [unwired: 2 in, 1 out]
                    n2089 = Concatenate Strings("window -a NVtGraph;\nlayer.x.type=", w3590, "; layer.x.label.numFormat = ", w3585, "; Y3 = 1; X3 = 1;", "window -a NVtTable;\nwindow -s TV;") -> (w3588:string)
                    n2090 = call "Origin_Export_7_27a_JW.vi"("Input Conditions"=w3592, "Analysis Array"=w3598, "error in (no error)"=w3600, "Parameter Worksheet Name"="[NVTTable]Trap Densities", "Parameter Folder Script"="pe_cd \"N-Vt\";", "Origin.IOApplication"=w3597) -> ("error out"=w3599:errorcluster, "reference out"=w3601:refnum<k7>)  [unwired: 3 in, 1 out]
                    n2091 = call "OAExecute.vi"("script"=w3588, "Error IO"=w3599, "Origin.IOApplication"=w3601) -> ()  [unwired: 1 in, 3 out]
                  }
                  frame #4 {
                    n2092 = local read "X Axis Display Type"() -> (w3606:string)
                    n2093 = local read "Opj X Axis"() -> (w3611:string)
                    n2094 = Concatenate Strings("window -a OffIGraph;\nlayer.x.type=", w3611, "; layer.x.label.numFormat = ", w3606, "; Y3 = 1; X3 = 1;", "window -a OffITable;\nwindow -s TV;") -> (w3609:string)
                    n2095 = call "Param_Analysis_7_24b_JW.vi"("Independant Variable"=w3614, "error in (no error)"=w3617, "Data Folder"=w3615, "Parameter String"="Off I-Sat (A):", "Parameter Name"="Off I-Sat", "Stats Folder"=w3616) -> ("error out"=w3621:errorcluster, "Output Array"=w3619:string[][], "Variables"=w3613:T18)  [unwired: 2 in, 1 out]
                    n2096 = call "Origin_Export_7_27a_JW.vi"("Input Conditions"=w3613, "Analysis Array"=w3619, "error in (no error)"=w3621, "Parameter Worksheet Name"="[OffItable]OffCurrents", "Parameter Folder Script"="pe_cd \"OffI-Sat\";", "Origin.IOApplication"=w3618) -> ("error out"=w3620:errorcluster, "reference out"=w3622:refnum<k7>)  [unwired: 3 in, 1 out]
                    n2097 = call "OAExecute.vi"("script"=w3609, "Error IO"=w3620, "Origin.IOApplication"=w3622) -> ()  [unwired: 1 in, 3 out]
                  }
                  frame #5 {
                    n2098 = local read "X Axis Display Type"() -> (w3627:string)
                    n2099 = local read "Opj X Axis"() -> (w3632:string)
                    n2100 = Concatenate Strings("window -a OnOffGraph;\nlayer.x.type=", w3632, "; layer.x.label.numFormat = ", w3627, "; Y3 = 1; X3 = 1;", "window -a OnOffTable;\nwindow -s TV;") -> (w3630:string)
                    n2101 = call "Param_Analysis_7_24b_JW.vi"("Independant Variable"=w3635, "error in (no error)"=w3638, "Data Folder"=w3636, "Parameter String"="On/Off I-Sat:", "Parameter Name"="OnOff Ratio", "Stats Folder"=w3637) -> ("error out"=w3642:errorcluster, "Output Array"=w3640:string[][], "Variables"=w3634:T18)  [unwired: 2 in, 1 out]
                    n2102 = call "Origin_Export_7_27a_JW.vi"("Input Conditions"=w3634, "Analysis Array"=w3640, "error in (no error)"=w3642, "Parameter Worksheet Name"="[OnOffTable]On/Off Ratios", "Parameter Folder Script"="pe_cd \"OnOff-Ratio\";", "Origin.IOApplication"=w3639) -> ("error out"=w3641:errorcluster, "reference out"=w3643:refnum<k7>)  [unwired: 3 in, 1 out]
                    n2103 = call "OAExecute.vi"("script"=w3630, "Error IO"=w3641, "Origin.IOApplication"=w3643) -> ()  [unwired: 1 in, 3 out]
                  }
                  frame #6 {
                    n2104 = local read "X Axis Display Type"() -> (w3648:string)
                    n2105 = local read "Opj X Axis"() -> (w3653:string)
                    n2106 = call "Param_Analysis_7_24b_JW.vi"("Independant Variable"=w3656, "error in (no error)"=w3659, "Data Folder"=w3657, "Parameter String"="STS-Sat (V/decade):", "Parameter Name"="STS-Sat", "Stats Folder"=w3658) -> ("error out"=w3663:errorcluster, "Output Array"=w3661:string[][], "Variables"=w3655:T18)  [unwired: 2 in, 1 out]
                    n2107 = Concatenate Strings("window -a SGraph;\nlayer.x.type=", w3653, "; layer.x.label.numFormat = ", w3648, "; Y3 = 1; X3 = 1;", "window -a STable;\nwindow -s TV;") -> (w3651:string)
                    n2108 = call "Origin_Export_7_27a_JW.vi"("Input Conditions"=w3655, "Analysis Array"=w3661, "error in (no error)"=w3663, "Parameter Worksheet Name"="[STable]Threshold Swing", "Parameter Folder Script"="pe_cd \"STS-Sat\";", "Origin.IOApplication"=w3660) -> ("error out"=w3662:errorcluster, "reference out"=w3664:refnum<k7>)  [unwired: 3 in, 1 out]
                    n2109 = call "OAExecute.vi"("script"=w3651, "Error IO"=w3662, "Origin.IOApplication"=w3664) -> ()  [unwired: 1 in, 3 out]
                  }
                  frame #7 {
                    n2110 = local read "X Axis Display Type"() -> (w3669:string)
                    n2111 = local read "Opj X Axis"() -> (w3674:string)
                    n2112 = Concatenate Strings("window -a VtGraph;\nlayer.x.type=", w3674, "; layer.x.label.numFormat = ", w3669, "; Y3 = 1; X3 = 1;", "window -a VtTable;\nwindow -s TV;") -> (w3672:string)
                    n2113 = call "Param_Analysis_7_24b_JW.vi"("Independant Variable"=w3677, "error in (no error)"=w3682, "Data Folder"=w3680, "Parameter String"="Vt-Sat (V):", "Parameter Name"="Vt-Sat", "Stats Folder"=w3681) -> ("error out"=w3686:errorcluster, "Output Array"=w3684:string[][], "Variables"=w3676:T18)  [unwired: 2 in, 1 out]
                    n2114 = call "Origin_Export_7_27a_JW.vi"("Input Conditions"=w3676, "Analysis Array"=w3684, "error in (no error)"=w3686, "Parameter Worksheet Name"="[VtTable]Threshold Voltages", "Parameter Folder Script"="pe_cd \"Vt-Sat\";", "Origin.IOApplication"=w3683) -> ("error out"=w3685:errorcluster, "reference out"=w3687:refnum<k7>)  [unwired: 3 in, 1 out]
                    n2115 = call "OAExecute.vi"("script"=w3672, "Error IO"=w3685, "Origin.IOApplication"=w3687) -> ("Error IO Out"=w3678:errorcluster, "Origin.IOApplication"=w3679:refnum<k7>)  [unwired: 1 in, 1 out]
                  }
                }
                n2116 = Path To String(path=w3507) -> (string=w3506:string)
                n2117 = call "OAExecute.vi"("script"="pe_cd /; ", "Error IO"=w3502, "Origin.IOApplication"=w3501) -> ("Error IO Out"=w3508:errorcluster, "Origin.IOApplication"=w3509:refnum<k7>)  [unwired: 1 in, 1 out]
                n2118 = call <userlib>:"OASaveProject.vi"("path"=w3506, "Error IO"=w3508, "Origin.IOApplication"=w3509) -> ()  [unwired: 3 out]
              }
            }
          }
          event "Blank Button": Mouse Down {
            n2119 = event-data() -> ()  [unwired: 1 in, 7 out]
            n2120 = local read "Transfer File"() -> (w3702:path)
            n2121 = disable-structure shown="Disabled" {
              frame Disabled {
                n2122 = local read "Folder Index"() -> (w3703:dbl)
                n2123 = Decrement(x=w3703) -> (x-1=w3704:dbl)
                n2124 = local write "Folder Index"(w3704) -> ()
              }
              frame Enabled {
              }
            }
            n2125 = Strip Path(path=w3702) -> (stripped path=w3698:path, name=w3700:string)
            n2126 = Path To String(path=w3698) -> (string=w3697:string)
            n2127 = Concatenate Strings(w3697, "\\", "X_", w3700) -> (w3696:string)
            n2128 = String To Path(string=w3696) -> (path=w3695:path)
            n2129 = Move(source path=w3702, 10:w3695) -> ()  [unwired: 3 in, 3 out]
            n2130 = local write "Transfer File"(w3695) -> ()
          }
          event "Cancel Button": Mouse Down {
            (unwired) 6
            n2131 = event-data() -> ()  [unwired: 1 in, 7 out]
            n2132 = call "Simulate_Keyboard.vi"("Action"=2, "Virtual Key"=162) -> ()  [unwired: 7 in, 1 out]
          }
        }
        n2133 = Multiply(x=w493, y=10) -> (x*y=w495:sgl)
        n2134 = case shown="\"0\"" w534 {
          tunnel: w508 -> [w673 w679 w683 w685 w689 w691 w693 w695 w697 w699 w701 w703 w705 w707 w709 w711 w713 w715 w717 w719 w721 w723 w725 w727 w729 w731 w733 w735 w737 w739 w741 w743 w745 w747 w749 w751 w753 w755 w757 w759 w761 w763 w765 w767 w769 w771 w773 w775 w777 w779 w781 w783 w785 w787 w789 w791 w793 w795 w797 w799 w801 w803 w805 w807 w809 w811 w813 w815 w817 w819 w821 w823 w825 w827 w829 w831 w833 w835 w837 w839 w841 w843 w845 w847 w849 w851 w853 w855 w857 w859 w861 w863 w865 w867 w869 w871 w873 w875 w877 w879 w881 w883 w885 w887 w889]
          tunnel: [w673 w678 w682 w685 w689 w691 w693 w695 w697 w699 w701 w703 w705 w707 w709 w711 w713 w715 w717 w719 w721 w723 w725 w727 w729 w731 w733 w735 w737 w739 w741 w743 w745 w747 w749 w751 w753 w755 w757 w759 w761 w763 w765 w767 w769 w771 w773 w775 w777 w779 w781 w783 w785 w787 w789 w791 w793 w795 w797 w799 w801 w803 w805 w807 w809 w811 w813 w815 w817 w819 w821 w823 w825 w827 w829 w831 w833 w835 w837 w839 w841 w843 w845 w847 w849 w851 w853 w855 w857 w859 w861 w863 w865 w867 w869 w871 w873 w875 w877 w879 w881 w883 w885 w887 w889] -> w533
          tunnel: w509 -> [w675 w677 w681 w687 w688 w690 w692 w694 w696 w698 w700 w702 w704 w706 w708 w710 w712 w714 w716 w718 w720 w722 w724 w726 w728 w730 w732 w734 w736 w738 w740 w742 w744 w746 w748 w750 w752 w754 w756 w758 w760 w762 w764 w766 w768 w770 w772 w774 w776 w778 w780 w782 w784 w786 w788 w790 w792 w794 w796 w798 w800 w802 w804 w806 w808 w810 w812 w814 w816 w818 w820 w822 w824 w826 w828 w830 w832 w834 w836 w838 w840 w842 w844 w846 w848 w850 w852 w854 w856 w858 w860 w862 w864 w866 w868 w870 w872 w874 w876 w878 w880 w882 w884 w886 w888]
          tunnel: [w674 w677 w681 w686 w688 w690 w692 w694 w696 w698 w700 w702 w704 w706 w708 w710 w712 w714 w716 w718 w720 w722 w724 w726 w728 w730 w732 w734 w736 w738 w740 w742 w744 w746 w748 w750 w752 w754 w756 w758 w760 w762 w764 w766 w768 w770 w772 w774 w776 w778 w780 w782 w784 w786 w788 w790 w792 w794 w796 w798 w800 w802 w804 w806 w808 w810 w812 w814 w816 w818 w820 w822 w824 w826 w828 w830 w832 w834 w836 w838 w840 w842 w844 w846 w848 w850 w852 w854 w856 w858 w860 w862 w864 w866 w868 w870 w872 w874 w876 w878 w880 w882 w884 w886 w888] -> w532
          tunnel: w495 -> [w672 w676 w680 w684 _ _ _ _ _ _ _ _ _ _ _ _ _ _ _ _ _ _ _ _ _ _ _ _ _ _ _ _ _ _ _ _ _ _ _ _ _ _ _ _ _ _ _ _ _ _ _ _ _ _ _ _ _ _ _ _ _ _ _ _ _ _ _ _ _ _ _ _ _ _ _ _ _ _ _ _ _ _ _ _ _ _ _ _ _ _ _ _ _ _ _ _ _ _ _ _ _ _ _ _ _]
          frame "DOWN" {
            n2135 = Add(x=w675, y=w672) -> (x+y=w674:sgl)
          }
          frame "LEFT" {
            n2136 = Subtract(x=w679, y=w676) -> (x-y=w678:sgl)
          }
          frame "RIGHT" {
            n2137 = Add(x=w683, y=w680) -> (x+y=w682:sgl)
          }
          frame "UP" {
            n2138 = Subtract(x=w687, y=w684) -> (x-y=w686:sgl)
          }
          frame "ENTER (num pad)" {
          }
          frame "' (quote)" {
          }
          frame "END" {
          }
          frame "EQUALS" {
          }
          frame "ESCAPE" {
          }
          frame "GRAVE (`)" {
          }
          frame "HOME" {
          }
          frame "INSERT" {
          }
          frame "LBRACKET" {
          }
          frame "LCONTROL" {
          }
          frame "L ALT" {
          }
          frame "LSHIFT" {
          }
          frame "LWIN" {
          }
          frame "MINUS" {
          }
          frame "MULTIPLY" {
          }
          frame "NEXT" {
          }
          frame "NUMLOCK" {
          }
          frame "NUMPAD_0" {
          }
          frame "NUMPAD_1" {
          }
          frame "NUMPAD_2" {
          }
          frame "NUMPAD_3" {
          }
          frame "NUMPAD_4" {
          }
          frame "NUMPAD_5" {
          }
          frame "NUMPAD_6" {
          }
          frame "NUMPAD_7" {
          }
          frame "NUMPAD_8" {
          }
          frame "NUMPAD_9" {
          }
          frame "PAUSE" {
          }
          frame "PERIOD" {
          }
          frame "PRIOR (PG UP)" {
          }
          frame "RBRACKET" {
          }
          frame "RCONTROL" {
          }
          frame "RETURN" {
          }
          frame "R ALT" {
          }
          frame "RSHIFT" {
          }
          frame "RWIN" {
          }
          frame "SCROLL" {
          }
          frame "SEMICOLON" {
          }
          frame "SLASH" {
          }
          frame "SPACE" {
          }
          frame "SUBTRACT" {
          }
          frame "TAB" {
          }
          frame "DIVIDE" {
          }
          frame "DELETE" {
          }
          frame "DECIMAL" {
          }
          frame "COMMA" {
          }
          frame "CAPITAL" {
          }
          frame "BACKSLASH" {
          }
          frame "BACK" {
          }
          frame "ADD" {
          }
          frame "F15" {
          }
          frame "F14" {
          }
          frame "F13" {
          }
          frame "F12" {
          }
          frame "F11" {
          }
          frame "F10" {
          }
          frame "F9" {
          }
          frame "F8" {
          }
          frame "F7" {
          }
          frame "F6" {
          }
          frame "F5" {
          }
          frame "F4" {
          }
          frame "F3" {
          }
          frame "F2" {
          }
          frame "F1" {
          }
          frame "Z" {
          }
          frame "Y" {
          }
          frame "X" {
          }
          frame "W" {
          }
          frame "V" {
          }
          frame "U" {
          }
          frame "T" {
          }
          frame "S" {
          }
          frame "R" {
          }
          frame "Q" {
          }
          frame "P" {
          }
          frame "O" {
          }
          frame "N" {
          }
          frame "M" {
          }
          frame "L" {
          }
          frame "K" {
          }
          frame "J" {
          }
          frame "I" {
          }
          frame "H" {
          }
          frame "G" {
          }
          frame "F" {
          }
          frame "E" {
          }
          frame "D" {
          }
          frame "C" {
          }
          frame "B" {
          }
          frame "A" {
          }
          frame "9" {
          }
          frame "8" {
          }
          frame "7" {
          }
          frame "6" {
          }
          frame "5" {
          }
          frame "4" {
          }
          frame "3" {
          }
          frame "2" {
          }
          frame "1" {
          }
          frame "0" {
          }
        }
        n2139 = Bundle(w511, w510, w525, w524, 0.0) -> (w523:cluster{dbl, dbl, dbl, dbl, dbl})  [unwired: 1 in]
        n2140 = Bundle("X"=w533, "Y"=w532) -> (w527:cluster{"X":sgl, "Y":sgl})  [unwired: 1 in]
        n2141 = Divide(x=20, y=w494) -> (x/y=w497:sgl)
        n2142 = property on="Image Out" class="ImageControl"("Image Center Position"=w527) -> ()  [unwired: 2 in, 2 out]
        n2143 = call "IMAQ Convert Rectangle to ROI (Polygon)"("Rectangle"=w523) -> ("ROI Descriptor"=w521:T4)  [unwired: 7 in, 2 out]
        n2144 = Bundle("Application Font", w497, w501, w501, w501, w501, w501, TRUE, w499) -> (w503:T19)  [unwired: 1 in]
        n2145 = property on="Image Out 2" class="ImageControl"("ROI"=w521) -> ()  [unwired: 2 in, 2 out]
        n2146 = Bundle(w499, w503, w499, w499) -> (w502:T20)  [unwired: 1 in]
        n2147 = property on="Image Out" class="ImageControl"() -> ("ROI"=w486:T12)  [unwired: 2 in, 2 out]
        n2148 = Unbundle By Name(w486) -> ("Contours"=w550:T16)
        n2149 = local read "Image Out"() -> (w505:T2)
        n2150 = call "IMAQ Clear Overlay"("Image"=w505) -> ("Image Out"=w504:T2)  [unwired: 9 in, 1 out]
        n2151 = Initialize Array(0) -> (w548:i32[])  [unwired: 1 in]
        n2152 = local read "Magnification"() -> (w539:u16)
        n2153 = Array Size(array=w550) -> (size(s)=w549:i32)
        n2154 = Build Array(0.505025, 0.252522, 0.127742, 0.050345, 0.031129) -> (w540:dbl[])
        n2155 = Array Subset(array=w540, index=w539, length=1) -> (w537:dbl[])
        n2156 = property on="Image Out" class="ImageControl"() -> ("ZoomInteger"=w529:cluster{"X":i32, "Y":i32})  [unwired: 2 in, 2 out]
        n2157 = To Double Precision Float(number=w537) -> (double precision float=w536:dbl[])
        n2158 = for {
          N: w549 -> [_]
          shift-right: [w912] -> _
          shift-left: w550 -> [w912]
          shift-right: [w910] -> w535
          shift-left: w548 -> [w909]
          tunnel: w536 -> [w908]
          shift-right: [w905] -> _
          shift-left: w504 -> [w907]
          tunnel: w502 -> [w900]
          i -> [w904]
          n2159 = Index Array(array=w912, index=w904) -> (element=w921:T21)
          n2160 = Unbundle(w921) -> ("Points"=w920:i32[])  [unwired: 2 out]
          n2161 = Array To Cluster(array=w920) -> (cluster=w919:T22)
          n2162 = Unbundle(w919) -> ("Points[0]"=w899:i32, "Points[1]"=w896:i32, "Points[2]"=w911:i32, "Points[3]"=w917:i32)  [unwired: 5 out]
          n2163 = Add(x=w899, y=10) -> (x+y=w897:i32)
          n2164 = Subtract(x=w896, y=w917) -> (x-y=w916:i32)
          n2165 = Subtract(x=w899, y=w911) -> (x-y=w918:i32)
          n2166 = Square(x=w916) -> (x^2=w914:i32)
          n2167 = Square(x=w918) -> (x^2=w915:i32)
          n2168 = Add(x=w915, y=w914) -> (x+y=w913:i32)
          n2169 = Square Root(x=w913) -> (sqrt(x)=w890:dbl)
          n2170 = Multiply(x=w890, y=0.5) -> (x*y=w893:dbl)
          n2171 = Add(x=w893, y=w896) -> (x+y=w895:dbl)
          n2172 = Bundle(w897, w895) -> (w906:cluster{i32, dbl})  [unwired: 1 in]
          n2173 = Multiply(x=w890, y=w908) -> (x*y=w903:dbl[])
          n2174 = Index Array(array=w903) -> (element=w902:dbl)  [unwired: 1 in]
          n2175 = Number To Fractional String(number=w902) -> (F-format string=w901:string)  [unwired: 3 in]
          n2176 = call "IMAQ Overlay Text"("BG Color (Transparent)"=u32 0, "Text Color (black)"=u32 16448250, "Font, Size & Style"=w900, "String"=w901, "Origin"=w906, "Image"=w907) -> ("Image Out"=w905:T2)  [unwired: 4 in, 1 out]
          n2177 = Build Array (concatenate)(w909, w903) -> (w910:dbl[])
          n2178 = local write "Numeric 3"(w890) -> ()
        }
        n2179 = local write "ROI Descriptor"(w486) -> ()
        n2180 = Unbundle(w529) -> ("X"=w528:i32)  [unwired: 1 out]
        n2181 = Add Array Elements(numeric array=w535) -> (sum=w546:dbl)
        n2182 = local write "Distances"(w535) -> ()
        n2183 = local write "Total Width"(w546) -> ()
        n2184 = local write "Zoom"(w528) -> ()
        n2185 = local read "Manual-Width"() -> (w452:bool)
        n2186 = local read "Total Width"() -> (w489:dbl)
        n2187 = local read "Rec: Width"() -> (w487:dbl)
        n2188 = case shown="False" w452 {
          frame False {
            n2189 = property on="New: Width" class="DigNum (strict)"("DisabledEnum"=1) -> ()  [unwired: 2 in, 2 out]
          }
          frame True {
            n2190 = property on="New: Width" class="DigNum (strict)"("DisabledEnum"=0) -> ()  [unwired: 2 in, 2 out]
          }
        }
        n2191 = Not(x=w452) -> (.not. x?=w484:bool)
        n2192 = Equal To 0?(x=w489) -> (x = 0?=w485:bool)
        n2193 = Or(x=w485, y=w452) -> (x .or. y?=w488:bool)
        n2194 = And(x=w485, y=w484) -> (x .and. y?=w483:bool)
        n2195 = case shown="True" w483 {
          tunnel: w487 -> [_ w648]
          frame False {
          }
          frame True {
            n2196 = local write "New: Width"(w648) -> ()
          }
        }
        n2197 = case shown="False" w488 {
          tunnel: w489 -> [w650 _]
          frame False {
            n2198 = local write "New: Width"(w650) -> ()
            n2199 = property on="New: Width" class="DigNum (strict)"("DisabledEnum"=1) -> ()  [unwired: 2 in, 2 out]
          }
          frame True {
            n2200 = property on="New: Width" class="DigNum (strict)"("DisabledEnum"=0) -> ()  [unwired: 2 in, 2 out]
          }
        }
        n2201 = local read "Manual Comments"() -> (w453:bool)
        n2202 = local read "Rec: Comments"() -> (w454:string)
        n2203 = local read "Manuel-Dielectric"() -> (w480:bool)
        n2204 = local read "Rec: Dielectric (d)"() -> (w479:dbl)
        n2205 = local read "Manuel-Length"() -> (w481:bool)
        n2206 = local read "Rec: Length"() -> (w482:dbl)
        n2207 = case shown="True" w453 {
          tunnel: w454 -> [w631 _]
          frame False {
            n2208 = local write "Comments:"(w631) -> ()
            n2209 = property on="Comments:" class="Str"("DisabledEnum"=1) -> ()  [unwired: 2 in, 2 out]
          }
          frame True {
            n2210 = property on="Comments:" class="Str"("DisabledEnum"=0) -> ()  [unwired: 2 in, 2 out]
          }
        }
        n2211 = case shown="True" w481 {
          tunnel: w482 -> [w646 _]
          frame False {
            n2212 = local write "New: Length"(w646) -> ()
            n2213 = property on="New: Length" class="DigNum (strict)"("DisabledEnum"=1) -> ()  [unwired: 2 in, 2 out]
          }
          frame True {
            n2214 = property on="New: Length" class="DigNum (strict)"("DisabledEnum"=0) -> ()  [unwired: 2 in, 2 out]
          }
        }
        n2215 = case shown="True" w480 {
          tunnel: w479 -> [w643 _]
          frame False {
            n2216 = local write "New: Dielectric"(w643) -> ()
            n2217 = property on="New: Dielectric" class="DigNum (strict)"("DisabledEnum"=1) -> ()  [unwired: 2 in, 2 out]
          }
          frame True {
            n2218 = property on="New: Dielectric" class="DigNum (strict)"("DisabledEnum"=0) -> ()  [unwired: 2 in, 2 out]
          }
        }
      }
    }
  }
  n2219 = disable-structure shown="Disabled" {
    frame Disabled {
      # "Transformer Work"
      n2220 = Build Array("DeviceID", "Fabricator", "Deposition", "Date", "Sample", "Row", "Column", "L (um)", "W (um)", "Material", "Treatment", "TC (mM)", "Solvent", "C (%)", "ST (C)", "Drops", "Wait (s)", "RT (F)", "RH (%)", "Ramp (s)", "RPM", "Accel (RPM/s)", "Time (s)", "Mobility", "On/Off", "Vt", "S.T.S") -> (→"Transformer \nHeaders":string[])
    }
    frame Enabled {
    }
  }
